vi "Main.vi"() -> ()   [LabVIEW 2018]
uses:
  <vilib>/picture/picture.llb/imagedata.ctl
  <vilib>/Utility/miscctls.llb/LVPoint32TypeDef.ctl
  <vilib>/Utility/miscctls.llb/LVMouseTypeDef.ctl
  <vilib>/Utility/miscctls.llb/LVPositionTypeDef.ctl
  <vilib>/Utility/miscctls.llb/LVPointTypeDef.ctl
  <vilib>/Utility/miscctls.llb/LVRectTypeDef.ctl
  Shared Variables/Alarm Cluster (UI).ctl
  Shared Variables/Alarm Cluster.ctl
  Drag and Drop/State Cluster.ctl
  support/Message Queue/Message Cluster.ctl
  Drag and Drop/Thumbnail Cluster.ctl
  Drag and Drop/Object Cluster.ctl
  Drag and Drop/Object Type Enum.ctl
  Config Module/Controls/Main Config Cluster.ctl
  OPC/OPC Module Config.ctl
  Scale Module Folder/Measure Instrument/State Enum.ctl
  OPC/OPC Settings.ctl
  OPC/Variable Data Cluster.ctl
  <vilib>/OPCUA/controls/NodeId.ctl
  <vilib>/OPCUA/controls/OPC UA StatusCode.ctl
  <vilib>/OPCUA/controls/Subscription ID.ctl
  <vilib>/OPCUA/controls/OPC UA Client Refnum.ctl
  <vilib>/OPCUA/controls/Subscription Data Change.ctl
  <vilib>/OPCUA/controls/Data Type.ctl
  OPC/OPC Tag Data.ctl
  Feed Module/Controls/Feed Module Config Cluster.ctl
  Feed Module/Controls/Feed Module Settings Cluster.ctl
  Ismatec ISM 831C/Controls/Ismatech ISM831C Settings Cluster.ctl
  Masterflex 7550-30/Controls/Settings Cluster.ctl
  Mettler Toledo/Controls/Settings Cluster.ctl
  Bronkhorst M13 Flow Meter/Settings Cluster.ctl
  Measure Instrument/PID 2 Parameters Cluster.ctl
  Measure Instrument/PID Input Enum.ctl
  Measure Instrument/PID 2 Output Enum.ctl
  Tacmina QI/Tacmina QI DAQ Setting.ctl
  KNF Pump/Settings Cluster plus SIMDOS.ctl
  ASIA Pump/Pump Settings.ctl
  VICI M50 Party Mode/Settings Cluster.ctl
  FLOM Pump/Settings Cluster.ctl
  SSI PR Class/SSI PR or LD Settings Cluster.ctl
  Masterflex 75211/Masterflex 75211 DAQ Setting.ctl
  SSI PR Class/SSI P40 Settings Cluster.ctl
  Ismatec 78001/Ismatec 4083.ctl
  Bronkhorst M14 Flow Meter/Settings Cluster.ctl
  TT Module/Controls/TT Module Config Cluster.ctl
  Tag VIs/Numeric Alarm Settings Cluster.ctl
  Acquisition/Hardware Configuration.ctl
  Acquisition/Task Cluster.ctl
  PT Module/Controls/PT Module Config Cluster.ctl
  Scale Module Folder/Feed Module/Controls/Scale Module Config Cluster.ctl
  Scale Module Folder/Feed Module/Controls/Scale Module Settings Cluster.ctl
  Pump Module Folder/Pump Module Config Cluster.ctl
  Pump Module Folder/Pump Module Settings Cluster.ctl
  LabJack Module/Controls/U3 Module Config Cluster.ctl
  Decoration Module/Decoration Module Config Cluster.ctl
  Flow Module Folder/Feed Module/Controls/Flow Module Config Cluster.ctl
  Flow Module Folder/Feed Module/Controls/Flow Module Settings Cluster.ctl
  TCU Module/TCU Module Folder/TCU Module Config Cluster.ctl
  TCU Module/TCU Module Folder/TCU Module Settings Cluster.ctl
  TCU Module/TCU Module Folder/Measure Instrument/Output Devices.ctl
  Huber TCU/Huber Settings.ctl
  Lauda Integral XT-150 TCU/Lauda Settings.ctl
  Julabo Type 1 TCU/Julabo Type 1 TCU Folder/Julabo FP-50 Settings.ctl
  Huber Unistat 410 TCU/Huber Unistat 410 RS485 Settings.ctl
  D-O Module Folder/Not Sure Where this is Used.ctl
  Sequencing/Squence Control.ctl
  D-O Module Folder/D-O Module Config Cluster.ctl
  D-O Module Folder/Valve Clusters.ctl
  D-O Module Folder/D-O Module Settings Cluster.ctl
  D-O Module Folder/D-O Device Settings Cluster.ctl
  VICI Electronic Actuator/VICI Electronic Actuator Settings.ctl
  Pressure Regulator Control Module/Pressure Regulator/Controls/4-20mA Module Config Cluster.ctl
  Pressure Regulator Control Module/Pressure Regulator/Controls/4-20mA Module Settings Cluster.ctl
  Pressure Transmitter/Pressure Transmitter Device Settings.ctl
  Pressure Reg Module/Pressure Regulator Device Settings.ctl
  Sonicator Module Folder/Feed Module/Controls/Sonicator Module Config Cluster.ctl
  Sonicator Module Folder/Feed Module/Controls/Sonicator Module Settings Cluster.ctl
  Sonic Systems P100/Sonic Systems P100 Settings.ctl
  Agitator Module Folder/Feed Module/Controls/Agitator Module Config Cluster.ctl
  Agitator Module Folder/Feed Module/Controls/Agitator Module Settings Cluster.ctl
  Tag VIs/Tag FGV Operation Enum.ctl
  Shared Variables/Alarm Log Operation Enum.ctl
  Drag and Drop/Drop Parameters Cluster.ctl
  Drag and Drop/Module Instance Number Operation Enum.ctl
  Drag and Drop/Module Type Enum.ctl
  <vilib>/Utility/error.llb/DialogType.ctl
  Config Module/Controls/Config File Operation Enum.ctl
  Waveform Loop/Start Params Cluster.ctl
  Ismatec 78001/Ismatec 4083 Global.ctl
  Ismatec 78001/Ismatec 4083 Global Element.ctl
  Pump Calibration Program/Pump Calibration Config.ctl
  support/Message Queue/Enqueue Message (Single).vi
  <vilib>/Utility/cursorutil.llb/Set Cursor (Icon Pict).vi
  Main/Main Globals.vi
  LabJack Module/U3 (Main).vit
  D-O Module Folder/D-O Module (Main).vi
  TCU Module/TCU Module Folder/TCU Module (Main).vi
  Flow Module Folder/Flow Module (Main).vi
  Sonicator Module Folder/Sonicator Module (Main).vi
  Agitator Module Folder/Agitator Module (Main).vi
  <vilib>/Utility/cursorutil.llb/Set Cursor (Cursor ID).vi
  support/Message Queue/Message Queue.lvlib
  support/User Event - Stop/User Event - Stop.lvlib
  support/Support Library.lvlib
  Drag and Drop/Drag and Drop.lvlib
  Feed Module/Feed Module.lvlib
  TT Module/TT Module.lvlib
  History Graph/History Graph.lvlib
  Waveform Loop/Waveform Loop.lvlib
  CSV Log/CSV Log.lvlib
  TDMS Log/TDMS Log.lvlib
  Shared Variables/Dynamic Shared Variables.lvlib
  DAQ/DAQ.lvlib
  Config Module/Config Module.lvlib
  Bronkhorst M13 Flow Meter/Bronkhorst M13 Flow Meter.lvlib
  Mettler Toledo/Mettler Toledo.lvlib
  Masterflex 7550-30/Masterflex 7550-30.lvlib
  Ismatec ISM 831C/Ismatec ISM 831C.lvlib
  PT Module/PT Module.lvlib
  Scale Module Folder/Scale Module.lvlib
  Pump Module Folder/Pump Module.lvlib
  <vilib>/lvdsc/NI_DSC.lvlib
  LabJack Module/U3 Module.lvlib
  Flow Module Folder/Flow Module.lvlib
  Tacmina QI/Tacmina QI.lvlib
  KNF Pump/KNF SIMDOS.lvlib
  Huber TCU/Huber Ministat 230 TCU.lvlib
  TCU Module/TCU Module Folder/TCU Module.lvlib
  Lauda Integral XT-150 TCU/Lauda TCU.lvlib
  Julabo Type 1 TCU/Julabo Type 1 TCU Folder/Julabo Type FP-50 TCU.lvlib
  ASIA Pump.lvlib
  Sequencing/Sequencing Library.lvlib
  VICI M50 Party Mode/VICI M6 M50 Party Mode.lvlib
  D-O Module Folder/D-O Module.lvlib
  Pressure Regulator Control Module/Pressure Regulator/4-20mA Module.lvlib
  Pressure Reg Module/Pressure Regulator Library.lvlib
  Pressure Transmitter/Pressure Transmitter Library.lvlib
  FLOM Pump/FLOM Pump.lvlib
  support/Command Log VIs/Command Logging.lvlib
  Calibration VIs/Calibration.lvlib
  Lauda Integral XT-150 TCU/TCP Library.lvlib
  SSI PR Class/SSI PR or LD Pump.lvlib
  Scale Module Folder/Measure Instrument/Scale Module Engine.lvlib
  OPC/OPC UA.lvlib
  D-O Module Folder/DIO Valve/VICI Electronic Actuator.lvlib
  subVIs/Main SubVIs.lvlib
  Masterflex 75211/Masterflex 75211.lvlib
  SSI PR Class/SSI P40 Pump.lvlib
  Huber Unistat 410 TCU/Huber Unistat 410 TCU.lvlib
  Ismatec 78001/Ismatec 4308.lvlib
  Bronkhorst M14 Flow Meter/Bronkhorst M14 Flow Meter.lvlib
  Sonicator Module Folder/Sonicator Module.lvlib
  Sonic Systems P100/Sonic Systems P100.lvlib
  Agitator Module Folder/Agitator Module.lvlib
panel:
  out "Cluster":T1 {"Main Config"."PR Module Configs"."Settings"."PID 2 Parameters"."output range"."output low" format="%.2f"; "Main Config"."PR Module Configs"."Settings"."PID 2 Parameters"."output range"."output high" min=0.0 max=100.0 format="%.2f"; "Main Config"."PR Module Configs"."Settings"."PID 2 Parameters"."PID gains"."derivative time (Td, min)" format="%.3f"; "Main Config"."PR Module Configs"."Settings"."PID 2 Parameters"."PID gains"."integral time (Ti, min)" format="%.3f"; "Main Config"."PR Module Configs"."Settings"."PID 2 Parameters"."PID gains"."proportional gain (Kc)" format="%.3f"; "Main Config"."Steps"."Control" items=["Pump %", "Setpoint"]; "Main Config"."TCU Module Configs"."Settings"."Huber Unistat 410 Settings"."Address" min=0 max=99 format="%02.0f"; "Main Config"."TCU Module Configs"."Settings"."Julabo FP-50 Settings"."Pump Power" min=0 max=8 step=1; "Main Config"."TCU Module Configs"."Settings"."Lauda Settings"."Pump Power" min=0 max=8 step=1; "Main Config"."Flow Module Configs"."Settings"."Bronkhorst M14 Settings"."Smoothing Steps" min=1 step=1; "Main Config"."Flow Module Configs"."Settings"."Bronkhorst M13 Settings"."Smoothing Steps" min=1 step=1; "Main Config"."Pump Module Configs"."Settings"."Ismatech 3 Channel Settings"."Channel Number" min=0 max=3; "Main Config"."Pump Module Configs"."Settings"."Ismatech 3 Channel Settings"."Pump Number" min=1; "Main Config"."Pump Module Configs"."Settings"."ASIA Pump C"."channel" min=0 max=1 step=1; "Main Config"."Pump Module Configs"."Settings"."Masterflex"."Pump Number" min=1.0 max=20.0 step=1.0; "Main Config"."Pump Module Configs"."Settings"."Ismatech"."Pump Number" min=1.0 max=20.0 step=1.0; "Main Config"."Feed Module Configs"."Settings"."Bronkhorst M14 Settings"."Smoothing Steps" min=1 step=1; "Main Config"."Feed Module Configs"."Settings"."Ismatech 3 Channel Settings"."Channel Number" min=0 max=3; "Main Config"."Feed Module Configs"."Settings"."Ismatech 3 Channel Settings"."Pump Number" min=1; "Main Config"."Feed Module Configs"."Settings"."output range"."output low" min=0.0 max=100.0 format="%.2f"; "Main Config"."Feed Module Configs"."Settings"."output range"."output high" format="%.2f"; "Main Config"."Feed Module Configs"."Settings"."PID 2 Parameters"."PID gains"."derivative time (Td, min)" format="%.3f"; "Main Config"."Feed Module Configs"."Settings"."PID 2 Parameters"."PID gains"."integral time (Ti, min)" format="%.3f"; "Main Config"."Feed Module Configs"."Settings"."PID 2 Parameters"."PID gains"."proportional gain (Kc)" format="%.3f"; "Main Config"."Feed Module Configs"."Settings"."Bronkhorst M13 Flow Meter"."Smoothing Steps" min=1 step=1; "Main Config"."Feed Module Configs"."Settings"."ASIA Pump C"."channel" min=0 max=1 step=1; "Main Config"."Feed Module Configs"."Settings"."Ismatech"."Pump Number" min=1.0 max=20.0 step=1.0; "Main Config"."Feed Module Configs"."Settings"."Masterflex"."Pump Number" min=1.0 max=20.0 step=1.0}
  in  "Alarm History Button":bool
  out "Alarm Model":T73[](array[typedef]) {"Alarm"."value" format="%.2f"; "Alarm"."setpoint" format="%.2f"; "Alarm"."clear time" format="%<%X\n%x>T"; "Alarm"."ack time" format="%<%X\n%x>T"; "Alarm"."set time" format="%<%X\n%x>T"}
  in  "UI Alarms":T74[](array[typedef])
  out "Message Data":variant
  out "data":errorcluster
  in  "End Program":bool
  out "CSV Log File":path
  out "error out":errorcluster
  in  "E-Stop":bool
  out "x-y":T4
  out "Front Panel Window:Panel Bounds":T4
  out "Drop Offset":T6
  out "Origin":T75
  out "Position":T6
  out "output cluster":cluster{"Coords":T10, "Mouse":T76}
  out "Mouse Position":cluster{"X":i32, "Y":i32}
  out "Path":path
  out "index of element":i32
  out "image data":T77
  in  "Notebook":string="Test"
  in  "Exit":bool
  in  "Settings":bool
  in  "Pause Log Button":bool
  in  "Force Trigger":bool
  in  "Start Log":bool
  out "Canvas":picture
  out "Palette":picture
  in  "?":T1 {"Main Config"."PR Module Configs"."Settings"."PID 2 Parameters"."output range"."output low" format="%.2f"; "Main Config"."PR Module Configs"."Settings"."PID 2 Parameters"."output range"."output high" min=0.0 max=100.0 format="%.2f"; "Main Config"."PR Module Configs"."Settings"."PID 2 Parameters"."PID gains"."derivative time (Td, min)" format="%.3f"; "Main Config"."PR Module Configs"."Settings"."PID 2 Parameters"."PID gains"."integral time (Ti, min)" format="%.3f"; "Main Config"."PR Module Configs"."Settings"."PID 2 Parameters"."PID gains"."proportional gain (Kc)" format="%.3f"; "Main Config"."Steps"."Control" items=["Pump %", "Setpoint"]; "Main Config"."TCU Module Configs"."Settings"."Huber Unistat 410 Settings"."Address" min=0 max=99 format="%02.0f"; "Main Config"."TCU Module Configs"."Settings"."Julabo FP-50 Settings"."Pump Power" min=0 max=8 step=1; "Main Config"."TCU Module Configs"."Settings"."Lauda Settings"."Pump Power" min=0 max=8 step=1; "Main Config"."Flow Module Configs"."Settings"."Bronkhorst M14 Settings"."Smoothing Steps" min=1 step=1; "Main Config"."Flow Module Configs"."Settings"."Bronkhorst M13 Settings"."Smoothing Steps" min=1 step=1; "Main Config"."Pump Module Configs"."Settings"."Ismatech 3 Channel Settings"."Channel Number" min=0 max=3; "Main Config"."Pump Module Configs"."Settings"."Ismatech 3 Channel Settings"."Pump Number" min=1; "Main Config"."Pump Module Configs"."Settings"."ASIA Pump C"."channel" min=0 max=1 step=1; "Main Config"."Pump Module Configs"."Settings"."Masterflex"."Pump Number" min=1.0 max=20.0 step=1.0; "Main Config"."Pump Module Configs"."Settings"."Ismatech"."Pump Number" min=1.0 max=20.0 step=1.0; "Main Config"."Feed Module Configs"."Settings"."Bronkhorst M14 Settings"."Smoothing Steps" min=1 step=1; "Main Config"."Feed Module Configs"."Settings"."Ismatech 3 Channel Settings"."Channel Number" min=0 max=3; "Main Config"."Feed Module Configs"."Settings"."Ismatech 3 Channel Settings"."Pump Number" min=1; "Main Config"."Feed Module Configs"."Settings"."output range"."output low" min=0.0 max=100.0 format="%.2f"; "Main Config"."Feed Module Configs"."Settings"."output range"."output high" format="%.2f"; "Main Config"."Feed Module Configs"."Settings"."PID 2 Parameters"."PID gains"."derivative time (Td, min)" format="%.3f"; "Main Config"."Feed Module Configs"."Settings"."PID 2 Parameters"."PID gains"."integral time (Ti, min)" format="%.3f"; "Main Config"."Feed Module Configs"."Settings"."PID 2 Parameters"."PID gains"."proportional gain (Kc)" format="%.3f"; "Main Config"."Feed Module Configs"."Settings"."Bronkhorst M13 Flow Meter"."Smoothing Steps" min=1 step=1; "Main Config"."Feed Module Configs"."Settings"."ASIA Pump C"."channel" min=0 max=1 step=1; "Main Config"."Feed Module Configs"."Settings"."Ismatech"."Pump Number" min=1.0 max=20.0 step=1.0; "Main Config"."Feed Module Configs"."Settings"."Masterflex"."Pump Number" min=1.0 max=20.0 step=1.0}
  # "little pump\ncentrifigual pump\nflow rate\npressure\nS or P to the left\nsolvent or process"
  # "Question: how do we make the live VI, such as the feed module graphic\nsized right for the picture that is loaded?\n\nProbably should standarize each module size. Then the  flow sheet\ndrawings will all just match the size and we don't have to worry about\nscale."
  # "Tasks\n1. Load graphic\n2. Drag and drop onto picture control\n3. Picture control draws hot spot\n4. If drag and drop on picture control, then resize and redraw the nearest hotspot\n5. When operator turns \"ON\" the system, then the hotspots are replaced with actual VIs."
  # "vertical or horizontal lines\nextendable"
  # "as much drawing room as possible"
  # "Agitator Settings"
  # "Sonicator Settings"
  # "Instrument Settings"
  # "Instrument Settings"
  # "Output Instruments"
  # "Flow Meter Settings"
  # "Output Instruments"
  # "Scale Settings"
  # "Output Instruments"
  # "Input Instruments"
  # "Agitator Settings"
  # "Sonicator Settings"
  # "Instrument Settings"
  # "Instrument Settings"
  # "Output Instruments"
  # "Flow Meter Settings"
  # "Output Instruments"
  # "Scale Settings"
  # "Output Instruments"
  # "Input Instruments"
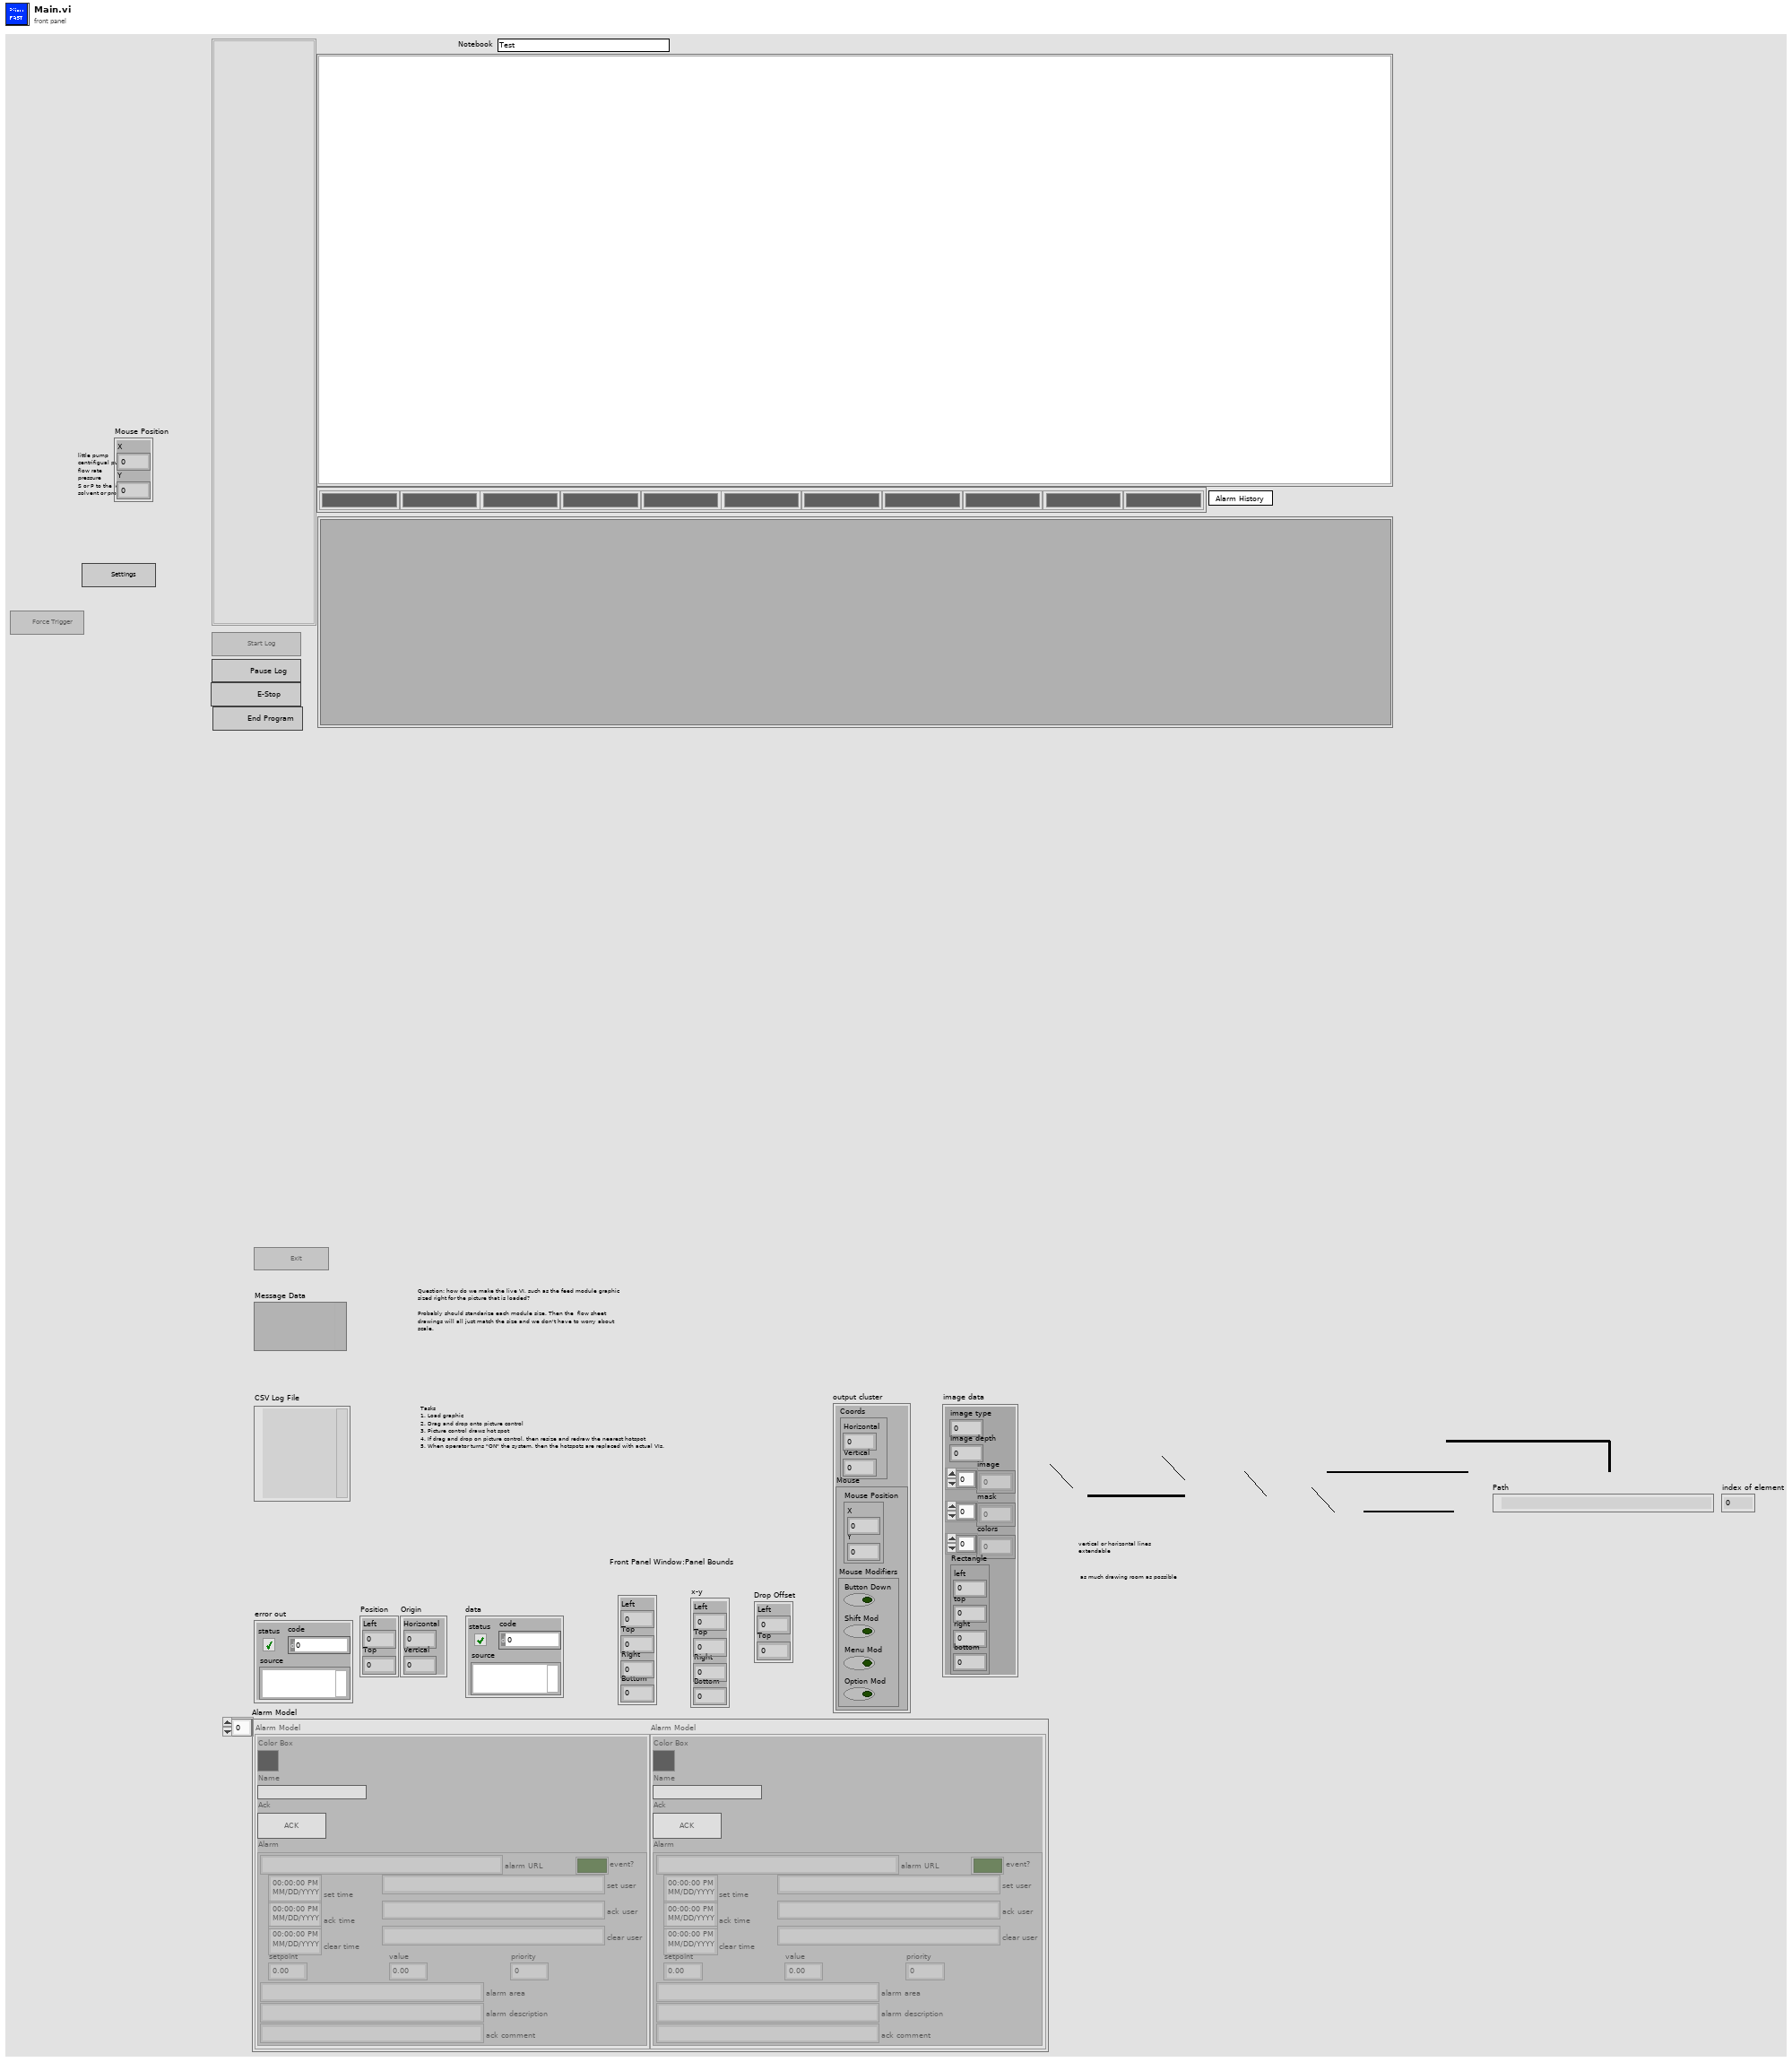
[diagram p1: front panel]
types:
  T1 = typedef "Drag and Drop.lvlib/State Cluster.ctl" = cluster{"VI refs":refnum<vi>[], "Queues":refnum<queue>[], "[Thumbnails]":T2[], "Drag Object Idx":i32, "[Objects]":T3[], "Active Object":i32, "Drop Offset":T6, "Process Name":string, "Main Config":T7, "Campaign Filepath":path, "Config Changed?":bool}
  T2 = typedef "Thumbnail Cluster.ctl" = cluster{"Path":path, "Rectangle":cluster{"left":i16, "top":i16, "right":i16, "bottom":i16}}
  T3 = typedef "Object Cluster.ctl" = cluster{"BMP Path":path, "Anchor Position":cluster{"X":i32, "Y":i32}, "Hot Spot":T4, "Type":T5, "Parameters":variant}
  T4 = typedef "LVRectTypeDef.ctl" = cluster{"Left":i16, "Top":i16, "Right":i16, "Bottom":i16}
  T5 = typedef "Object Type Enum.ctl" = enum16{"Icon", "Line", "Text", "Feed Module"}
  T6 = typedef "LVPositionTypeDef.ctl" = cluster{"Left":i32, "Top":i32}
  T7 = typedef "Config Module.lvlib/Main Config Cluster.ctl" = cluster{"Notebook":string, "OPC Module Configs":T8[], "Feed Module Configs":T18[], "Log File Path":path, "TT Module Configs":T37[], "DAQ Config":T39, "PT Module Configs":T41[], "Scale Module Configs":T42[], "Pump Module Configs":T44[], "U3 Module Configs":T46[], "Decoration Module Configs":T47[], "Flow Module Configs":T48[], "TCU Module Configs":T50[], "Steps":T57, "Abort":bool, "DO Module Configs":T59[], "PR Module Configs":T64[], "SC Module Configs":T68[], "AM Module Configs":T71[], "Cycle Period":dbl}
  T8 = typedef "OPC UA.lvlib/OPC Module Config.ctl" = cluster{"State":T9, "GUID":string, "Drop Coords":T10, "Configuration":T11, "First Iteration":bool, "Data":cluster{"Object Name":string, "Variable Array":T12[]}[], "Process Name":string, "Load Count":i32, "Log Started":bool, "subscription ID out":T15, "OPC UA client refnum out":T16, "Event Registration Refnum":refnum<event-registration>, "Start Time":timestamp, "Current Time":timestamp, "Tag Data":T17[]}
  T9 = typedef "Scale Module.lvlib/Scale Module Engine.lvlib/State Enum.ctl" = enum16{"Measuring", "Idle"}
  T10 = typedef "LVPoint32TypeDef.ctl" = cluster{"Horizontal":i32, "Vertical":i32}
  T11 = typedef "OPC UA.lvlib/OPC Settings.ctl" = cluster{"Cycle Period":dbl, "server endpoint URL":string, "security policy":cluster{"message mode":enum16{"None", "Sign", "Sign and Encrypt"}, "security":enum16{"Basic256", "Basic128Rsa15"}}, "Trust Any Server":bool}
  T12 = typedef "OPC UA.lvlib/Variable Data Cluster.ctl" = cluster{"node ID":T13, "browse name":string, "status":T14, "timestamp":timestamp, "value ":variant}
  T13 = typedef "NodeId.ctl" = string
  T14 = typedef "OPC UA StatusCode.ctl" = u32
  T15 = typedef "Subscription ID.ctl" = u32
  T16 = typedef "OPC UA Client Refnum.ctl" = refnum<k21>
  T17 = typedef "OPC UA.lvlib/OPC Tag Data.ctl" = cluster{"Include this Device":bool, "Device Name":string, "OPC Tag Data":cluster{"Tag":string, "Value":variant, "Time Stamp":timestamp}[]}
  T18 = typedef "Feed Module.lvlib/Feed Module Config Cluster.ctl" = cluster{"GUID":string, "Drop Coords":T10, "Process Name":string, "Queue Name":string, "Settings":T19, "Settings Load Count":i32, "OP Load Count":i32}
  T19 = typedef "Feed Module.lvlib/Feed Module Settings Cluster.ctl" = cluster{"Cycle Period":dbl, "Ismatech":T20, "Masterflex":T21, "Mettler":T22, "Bronkhorst M13 Flow Meter":T23, "PID 2 Parameters":T24, "Manual Entry":dbl, "Auto?":bool, "output range":cluster{"output high":dbl, "output low":dbl}, "Tacmina Settings":T27, "KNF SIMDOS Settings":T28, "ASIA Pump C":T29, "VICI Settings":T30, "FLOM Settings":T31, "SSI PR/LD Settings":T32, "Masterflex 75211 Settings":T33, "SSI P40 Settings":T34, "Ismatech 3 Channel Settings":T35, "Bronkhorst M14 Settings":T36}
  T20 = typedef "Ismatec ISM 831C.lvlib/Ismatech ISM831C Settings Cluster.ctl" = cluster{"VISA resource name":refnum<visa-resource-name>, "Simulated?":bool, "Pump Number":dbl, "Reverse?":bool}
  T21 = typedef "Masterflex 7550-30.lvlib/Settings Cluster.ctl" = cluster{"VISA resource name":refnum<visa-resource-name>, "Simulated?":bool, "Pump Number":dbl, "Reverse?":bool}
  T22 = typedef "Mettler Toledo.lvlib/Settings Cluster.ctl" = cluster{"VISA resource name":refnum<visa-resource-name>, "Simulated?":bool}
  T23 = typedef "Bronkhorst M13 Flow Meter.lvlib/Settings Cluster.ctl" = cluster{"VISA resource name":refnum<visa-resource-name>, "Simulated?":bool, "Smoothing Steps":i32}
  T24 = typedef "PID 2 Parameters Cluster.ctl" = cluster{"Input Device":T25, "Output Device":T26, "Setpoint":dbl, "PID gains":cluster{"proportional gain (Kc)":dbl, "integral time (Ti, min)":dbl, "derivative time (Td, min)":dbl}}
  T25 = typedef "PID Input Enum.ctl" = enum16{"Default", "Bronkhorst M13", "Bronkhorst M14", "Scale Rate of Change"}
  T26 = typedef "PID 2 Output Enum.ctl" = enum16{"Default", "Ismatec ISM 4308", "Ismatec ISM 831C", "Masterflex 7550-30", "VICI", "Tacmina QI", "KNF SIMDOS", "ASIA Type C", "FLOM UI-22-11", "SSI PR/LD", "SSI P40", "Masterflex 75211-70"}
  T27 = typedef "Tacmina QI.lvlib/Tacmina QI DAQ Setting.ctl" = cluster{"Analog DAQ Task":refnum<k21>, "Digital DAQ Task":refnum<k21>}
  T28 = typedef "KNF SIMDOS.lvlib/Settings Cluster plus SIMDOS.ctl" = cluster{"VISA resource name":refnum<visa-resource-name>, "Simulated?":bool}
  T29 = typedef "ASIA Pump.lvlib/Pump Settings.ctl" = cluster{"ASIA Pump #":i32, "channel":i32, "Simulated":bool}
  T30 = typedef "VICI M6 M50 Party Mode.lvlib/Settings Cluster.ctl" = cluster{"VISA resource name":refnum<visa-resource-name>, "Simulated?":bool, "Pump Letter":string, "Reverse?":bool}
  T31 = typedef "FLOM Pump.lvlib/Settings Cluster.ctl" = cluster{"VISA resource name":refnum<visa-resource-name>, "Simulated?":bool, "Pump Number":dbl}
  T32 = typedef "SSI PR or LD Pump.lvlib/SSI PR or LD Settings Cluster.ctl" = cluster{"VISA resource name":refnum<visa-resource-name>, "Simulated?":bool}
  T33 = typedef "Masterflex 75211.lvlib/Masterflex 75211 DAQ Setting.ctl" = cluster{"Analog DAQ Task":refnum<k21>, "Digital DAQ Task":refnum<k21>}
  T34 = typedef "SSI P40 Pump.lvlib/SSI P40 Settings Cluster.ctl" = cluster{"VISA resource name":refnum<visa-resource-name>, "Simulated?":bool}
  T35 = typedef "Ismatec 4308.lvlib/Ismatec 4083.ctl" = cluster{"VISA resource name":refnum<visa-resource-name>, "Pump Number":i16, "Channel Number":i16, "Simulated?":bool, "Reverse?":bool}
  T36 = typedef "Bronkhorst M14 Flow Meter.lvlib/Settings Cluster.ctl" = cluster{"VISA resource name":refnum<visa-resource-name>, "Simulated?":bool, "Smoothing Steps":i32}
  T37 = typedef "TT Module.lvlib/TT Module Config Cluster.ctl" = cluster{"GUID":string, "Drop Coords":T10, "Input Channel Tag Name ":string, "Process Name":string, "Queue Name":string, "Input Channel Numeric Alarm Settings":T38[]}
  T38 = typedef "Numeric Alarm Settings Cluster.ctl" = cluster{"enable? (F)":bool, "name":string, "alarm type":enum16{"HI_HI", "HI", "LO", "LO_LO"}, "level/change":dbl, "deadband/time":dbl, "alarm delay":dbl, "priority":u32, "ack type":enum16{"Auto", "User", "None", "Each Occurrence"}, "area":string, "description":string, "log? (T)":bool}
  T39 = typedef "DAQ.lvlib/Hardware Configuration.ctl" = cluster{"Tasks":T40[]}
  T40 = typedef "Task Cluster.ctl" = cluster{"DAQmx Task":refnum<k21>, "Read-Write Radio":enum32{"Read", "Write"}}
  T41 = typedef "PT Module.lvlib/PT Module Config Cluster.ctl" = cluster{"GUID":string, "Drop Coords":T10, "Input Channel Tag Name ":string, "Process Name":string, "Queue Name":string, "Input Channel Numeric Alarm Settings":T38[]}
  T42 = typedef "Scale Module.lvlib/Scale Module Config Cluster.ctl" = cluster{"GUID":string, "Drop Coords":T10, "Process Name":string, "Queue Name":string, "Settings":T43, "Load Count":i32}
  T43 = typedef "Scale Module.lvlib/Scale Module Settings Cluster.ctl" = cluster{"Cycle Period":dbl, "Mettler":T22, "Scale Type":string}
  T44 = typedef "Pump Module.lvlib/Pump Module Config Cluster.ctl" = cluster{"GUID":string, "Drop Coords":T10, "Process Name":string, "Queue Name":string, "Settings":T45, "Load Count":i32}
  T45 = typedef "Pump Module.lvlib/Pump Module Settings Cluster.ctl" = cluster{"Cycle Period":dbl, "Manual Entry":dbl, "Output Device":T26, "Ismatech":T20, "Ismatech 3 Channel Settings":T35, "Masterflex":T21, "VICI Settings":T30, "Tacmina Settings":T27, "KNF SIMDOS Settings":T28, "ASIA Pump C":T29, "FLOM Settings":T31, "SSI PR/LD Settings":T32, "SSI P40 Settings":T32, "Masterflex 75211 Settings":T33, "Pump Calibration File":path, "Calibration Slope":dbl, "Calibration Y Intercept":dbl, "Pump Cal Enum":u16}
  T46 = typedef "U3 Module.lvlib/U3 Module Config Cluster.ctl" = cluster{"GUID":string, "Drop Coords":T10, "AI Channel Number":enum16{"Default", "AI0", "AI1", "AI2", "AI3", "AI4", "AI5", "AI6", "AI7"}, "Process Name":string, "Queue Name":string, "Input Channel Numeric Alarm Settings":T38[]}
  T47 = typedef "Decoration Module Config Cluster.ctl" = cluster{"GUID":string, "Drop Coords":T10, "Decoration Filepath":path}
  T48 = typedef "Flow Module.lvlib/Flow Module Config Cluster.ctl" = cluster{"GUID":string, "Drop Coords":T10, "Process Name":string, "Queue Name":string, "Settings":T49, "Load Count":i32}
  T49 = typedef "Flow Module.lvlib/Flow Module Settings Cluster.ctl" = cluster{"Cycle Period":dbl, "Flow Meter Type":string, "Bronkhorst M13 Settings":T23, "Bronkhorst M14 Settings":T36}
  T50 = typedef "TCU Module.lvlib/TCU Module Config Cluster.ctl" = cluster{"GUID":string, "Drop Coords":T10, "Process Name":string, "Queue Name":string, "Settings":T51, "Load Count":i32, "Power Level Changed":bool}
  T51 = typedef "TCU Module.lvlib/TCU Module Settings Cluster.ctl" = cluster{"Cycle Period":dbl, "Setpoint Entry":dbl, "Output Device":T52, "Huber Ministat 230 Settings":T53, "Lauda Settings":T54, "Julabo FP-50 Settings":T55, "Internal Control?":bool, "Huber Unistat 410 Settings":T56}
  T52 = typedef "Output Devices.ctl" = enum16{"Default", "Huber Ministat 230", "Huber Unistat 410", "Lauda XT-150", "Julabo FP-50"}
  T53 = typedef "Huber Ministat 230 TCU.lvlib/Huber Settings.ctl" = cluster{"VISA resource name":refnum<visa-resource-name>, "Simulated?":bool}
  T54 = typedef "Lauda TCU.lvlib/Lauda Settings.ctl" = cluster{"VISA resource name":refnum<visa-resource-name>, "Simulated?":bool, "Pump Power":i32}
  T55 = typedef "Julabo Type FP-50 TCU.lvlib/Julabo FP-50 Settings.ctl" = cluster{"VISA resource name":refnum<visa-resource-name>, "Simulated?":bool, "Pump Power":i32}
  T56 = typedef "Huber Unistat 410 TCU.lvlib/Huber Unistat 410 RS485 Settings.ctl" = cluster{"VISA resource name":refnum<visa-resource-name>, "Address":i8, "Simulated?":bool}
  T57 = typedef "Not Sure Where this is Used.ctl" = T58[]
  T58 = typedef "Sequencing Library.lvlib/Squence Control.ctl" = cluster{"Module":string, "Control":u16, "Value":dbl, "Wait (sec)":dbl}
  T59 = typedef "D-O Module.lvlib/D-O Module Config Cluster.ctl" = cluster{"GUID":string, "Drop Coords":T10, "Process Name":string, "Queue Name":string, "Settings":T60, "Load Count":i32}
  T60 = typedef "D-O Module.lvlib/Valve Clusters.ctl" = cluster{"Valve Settings":T61, "Valve Type":enum16{"Default", "Digital Output Valve", "VICI Electronic Actuator"}, "Time On (Sec)":dbl, "Time Off (Sec)":dbl, "Run?":bool}
  T61 = typedef "D-O Module.lvlib/D-O Module Settings Cluster.ctl" = cluster{"D-O Settings":T62, "VICI Electronic Actuator":T63}
  T62 = typedef "D-O Module.lvlib/D-O Device Settings Cluster.ctl" = cluster{"DAQmx Task Name":refnum<k21>, "Output Channel":u16, "Output Channel Names":string[]}
  T63 = typedef "VICI Electronic Actuator.lvlib/VICI Electronic Actuator Settings.ctl" = cluster{"VISA resource name":refnum<visa-resource-name>, "Mode":enum16{"Two Positions With Stops", "Two Positions Without Stops", "Mutiposition"}, "Simulated":bool}
  T64 = typedef "4-20mA Module.lvlib/4-20mA Module Config Cluster.ctl" = cluster{"GUID":string, "Drop Coords":T10, "Process Name":string, "Queue Name":string, "Settings":T65, "Settings Load Count":i32}
  T65 = typedef "4-20mA Module.lvlib/4-20mA Module Settings Cluster.ctl" = cluster{"Cycle Period":dbl, "PID 2 Parameters":cluster{"Input Device":enum16{"Default", "4-20mA"}, "Output Device":enum16{"Default", "Equilibar Pressure Reg", "Flow Regulator"}, "Setpoint":dbl, "PID gains":cluster{"proportional gain (Kc)":dbl, "integral time (Ti, min)":dbl, "derivative time (Td, min)":dbl}, "output range":cluster{"output low":dbl, "output high":dbl}}, "Manual Entry":dbl, "Auto?":bool, "4-20mA Input Settings":T66, "4-20mA Out Settings":T67, "Input Channel Tag Name ":string}
  T66 = typedef "Pressure Transmitter Library.lvlib/Pressure Transmitter Device Settings.ctl" = cluster{"Input Channel ":u16}
  T67 = typedef "Pressure Regulator Library.lvlib/Pressure Regulator Device Settings.ctl" = cluster{"Output DAQ Task":refnum<k21>}
  T68 = typedef "Sonicator Module.lvlib/Sonicator Module Config Cluster.ctl" = cluster{"GUID":string, "Drop Coords":T10, "Process Name":string, "Queue Name":string, "Settings":T69, "Load Count":i32}
  T69 = typedef "Sonicator Module.lvlib/Sonicator Module Settings Cluster.ctl" = cluster{"Cycle Period":dbl, "Sonicator Type":string, "SS P100 Settings":T70, "Setpoint (µm)":dbl, "Cutoff (W)":dbl}
  T70 = typedef "Sonic Systems P100.lvlib/Sonic Systems P100 Settings.ctl" = cluster{"VISA resource name":refnum<visa-resource-name>, "Simulated?":bool}
  T71 = typedef "Agitator Module.lvlib/Agitator Module Config Cluster.ctl" = cluster{"GUID":string, "Drop Coords":T10, "Process Name":string, "Queue Name":string, "Settings":T72, "Load Count":i32}
  T72 = typedef "Agitator Module.lvlib/Agitator Module Settings Cluster.ctl" = cluster{"Cycle Period":dbl, "Agitator Type":string, "Setpoint (µm)":dbl}
  T73 = typedef "Dynamic Shared Variables.lvlib/Alarm Cluster.ctl" = cluster{"Color Box":u32, "Name":string, "Ack":bool, "Alarm":cluster{"alarm URL":string, "set time":timestamp, "set user":string, "ack time":timestamp, "ack user":string, "clear time":timestamp, "clear user":string, "setpoint":dbl, "value":dbl, "priority":u32, "alarm area":string, "alarm description":string, "ack comment":string, "event?":bool, "Refnum":u64}}
  T74 = typedef "Dynamic Shared Variables.lvlib/Alarm Cluster (UI).ctl" = cluster{"Color Box":u32, "Name":string, "Ack":bool}
  T75 = typedef "LVPointTypeDef.ctl" = cluster{"Horizontal":i16, "Vertical":i16}
  T76 = typedef "LVMouseTypeDef.ctl" = cluster{"Mouse Position":cluster{"X":i32, "Y":i32}, "Mouse Modifiers":cluster{"Button Down":bool, "Shift Mod":bool, "Menu Mod":bool, "Option Mod":bool}}
  T77 = typedef "imagedata.ctl" = cluster{"image type":i32, "image depth":i32, "image":u8[], "mask":u8[], "colors":u32[], "Rectangle":cluster{"left":i16, "top":i16, "right":i16, "bottom":i16}}
  T78 = typedef "Tag FGV Operation Enum.ctl" = enum16{"Init", "Set Notification Queue", "Create Tag", "Commit", "Write Tag (Numeric)", "Write Tag (Boolean)", "Read All Tags", "Read One Tag", "Delete Tag Category", "Set Alarm Parameters (Numeric)", "Set Alarm Parameters (Boolean)", "Enable All Alarms", "Disable All Alarms", "Delete All Tags", "Read Alarms", "Ack Alarm", "Read Alarm Parameters (Numeric)", "Read Alarm Parameters (Boolean)"}
  T79 = cluster{"Down":bool, "Mouse":T76, "Drag":bool, "Canvas":bool}
  T80 = cluster{"Busy":bool, "ChannelCnt":dbl, "Initialized":bool, "Current Channel":dbl, "Initialized Channels":dbl[]}[]
  T81 = cluster{"Busy":bool, "PumpCnt":dbl, "RemoteEntered":bool, "OverpressureSet":bool}[]
  T82 = typedef "Main Queue Cluster.ctl" = cluster{"UI":refnum<queue>, "Waveform Loop":refnum<queue>, "CSV Log":refnum<queue>, "TDMS Log":refnum<queue>, "Graphs":refnum<queue>[], "DAQ":refnum<queue>, "Sequence":refnum<queue>, "TCP Write":refnum<queue>, "Sequence UI":refnum<queue>, "OPC UA Log":refnum<queue>, "TCP Read":refnum<queue>}
  T83 = cluster{"Event Registration Refnum":refnum<event-registration>, "Stop Event Registration Refnum":refnum<event-registration>}
  T84 = typedef "Drag and Drop.lvlib/Module Type Enum.ctl" = enum16{"<unknown module>", "Feed", "TT", "PT", "Scale", "Flow", "Pump", "U3", "TCU", "DO", "PR", "OPC", "SC", "AM"}
  T85 = typedef "Module Instance Number Operation Enum.ctl" = enum16{"Init", "Next Instance Number"}
  T86 = typedef "Drop Parameters Cluster.ctl" = cluster{"Module VI Filepath":path, "Process Name":string, "Main UI Message Queue":refnum<queue>, "Drop Coords":T10, "Module Parameters":variant, "Name of Parent Window":string}
  T87 = enum8{"Enabled", "Disabled", "Disabled and Grayed Out"}
  T88 = typedef "Config Module.lvlib/Config File Operation Enum.ctl" = enum16{"Read", "Write"}
  T89 = typedef "Alarm Log Operation Enum.ctl" = enum16{"Create Log", "Log Alarm", "Close Log"}
  T90 = typedef "Waveform Loop.lvlib/Start Params Cluster.ctl" = cluster{"dt (seconds)":dbl, "CSV Logfile path":path, "TDMS Logfile path":path}
  T91 = typedef "Ismatec 4308.lvlib/Ismatec 4083 Global.ctl" = T92[]
  T92 = typedef "Ismatec 4308.lvlib/Ismatec 4083 Global Element.ctl" = cluster{"Busy":bool, "ChannelCnt":dbl, "Initialized":bool, "Current Channel":dbl, "Initialized Channels":dbl[]}
  T93 = typedef "Calibration.lvlib/Pump Calibration Config.ctl" = cluster{"Settings":cluster{"Cycle Period":dbl, "Ismatech":T20, "Masterflex":T21, "Bronkhorst M13 Settings":T23, "PID 2 Parameters":cluster{"Input Device":T25, "Output Device":T26}, "Tacmina Settings":T27, "KNF SIMDOS Settings":T28, "VICI M50 Settings":T30, "FLOM Settings":T31, "Calibration Limits":cluster{"Minimum (ml/min)":dbl, "Maximum (ml/min)":dbl, "Steps":dbl}, "SSI PR Settings":T32, "Ismatech 4308 Settings":T35, "Bronkhorst M14 Settings":T36}, "Flowmeter Output":dbl, "Density":dbl, "FL Temp":dbl, "Speed %":dbl, "File Refnum":refnum<file>, "Pump On?":enum16{"Off", "On", "Not Initialized"}}
  T94 = typedef "DialogType.ctl" = u16
  T95 = enum32{"Invalid", "Standard", "Closed", "Hidden", "Minimized", "Maximized"}
  T96 = cluster{"alarm URL":string, "set time":timestamp, "set user":string, "ack time":timestamp, "ack user":string, "clear time":timestamp, "clear user":string, "setpoint":dbl, "value":dbl, "priority":u32, "alarm area":string, "alarm description":string, "ack comment":string, "event?":bool, "Refnum":u64}[]
  T97 = cluster{"alarm URL":string, "set time":timestamp, "set user":string, "ack time":timestamp, "ack user":string, "clear time":timestamp, "clear user":string, "setpoint":dbl, "value":dbl, "priority":u32, "alarm area":string, "alarm description":string, "ack comment":string, "event?":bool, "Refnum":u64}
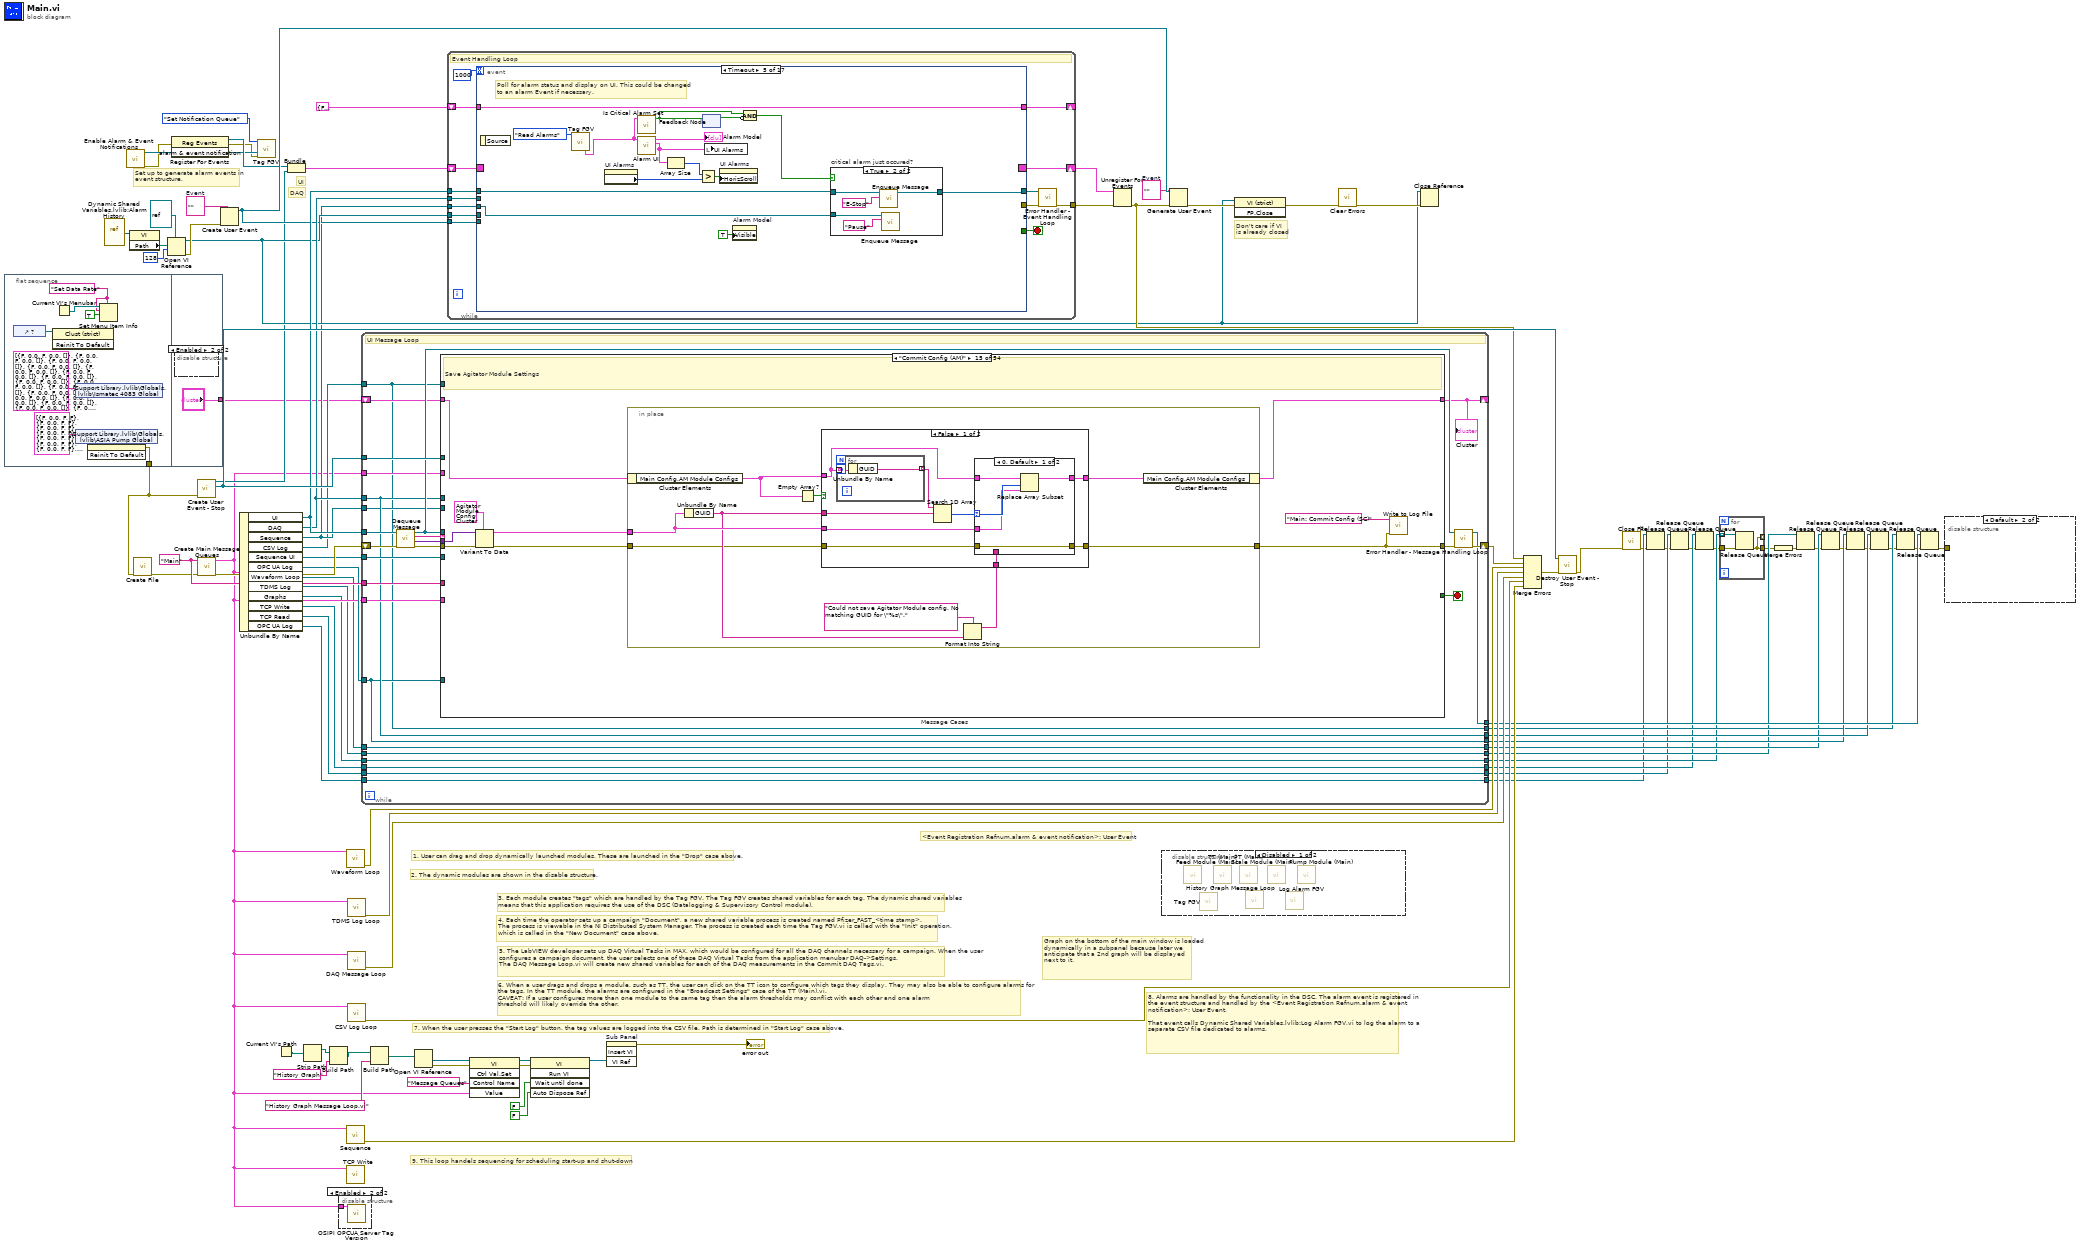
[diagram p0: block diagram]
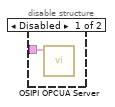
[diagram p2: hidden frame]
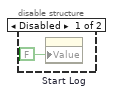
[diagram p3: hidden frame]
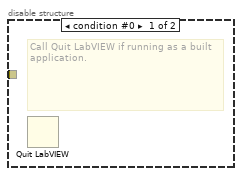
[diagram p4: hidden frame]
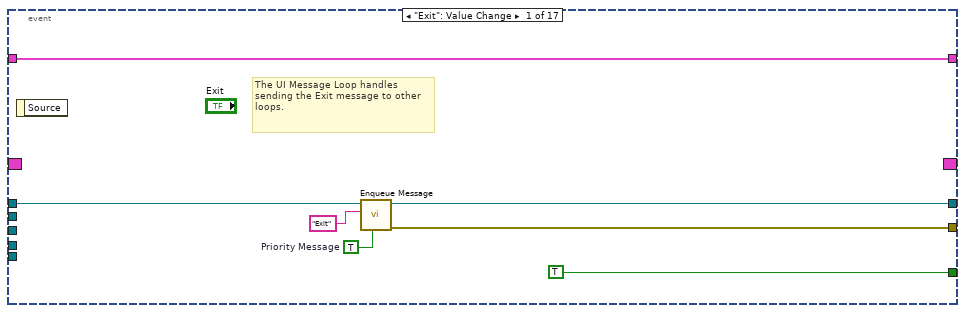
[diagram p6: hidden frame]
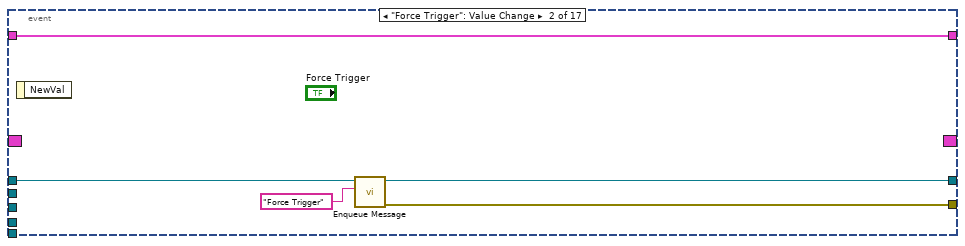
[diagram p7: hidden frame]
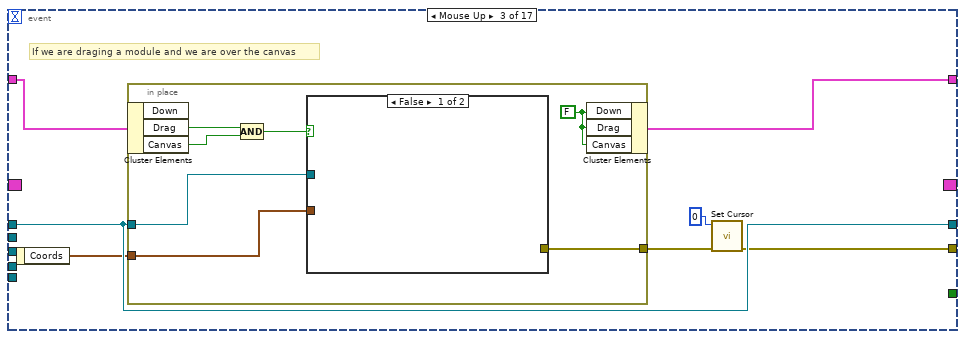
[diagram p8: hidden frame]
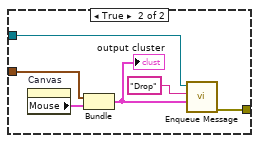
[diagram p9: hidden frame]
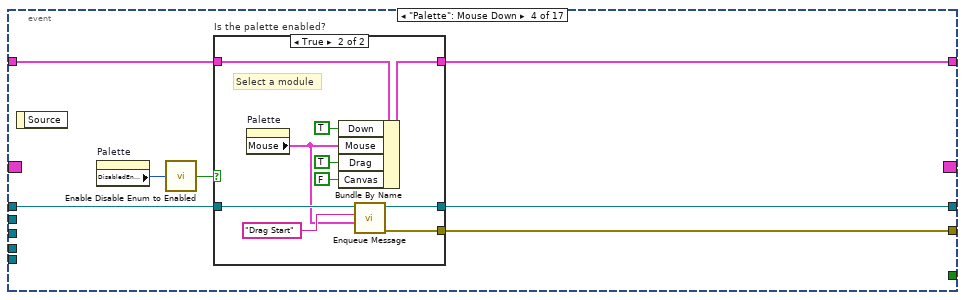
[diagram p10: hidden frame]
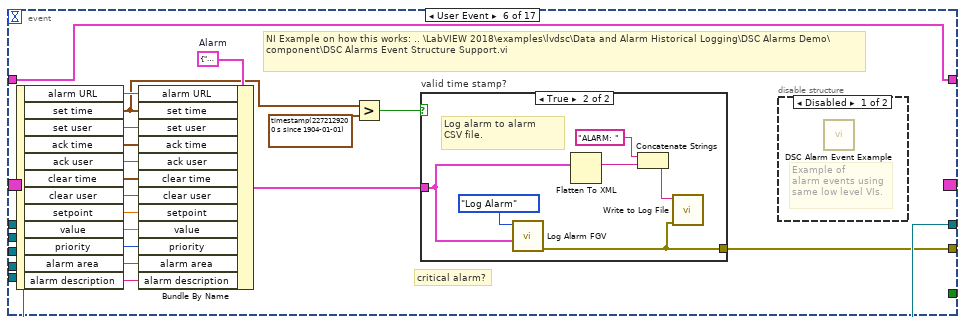
[diagram p13: hidden frame]
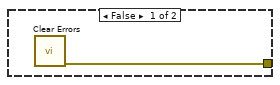
[diagram p15: hidden frame]
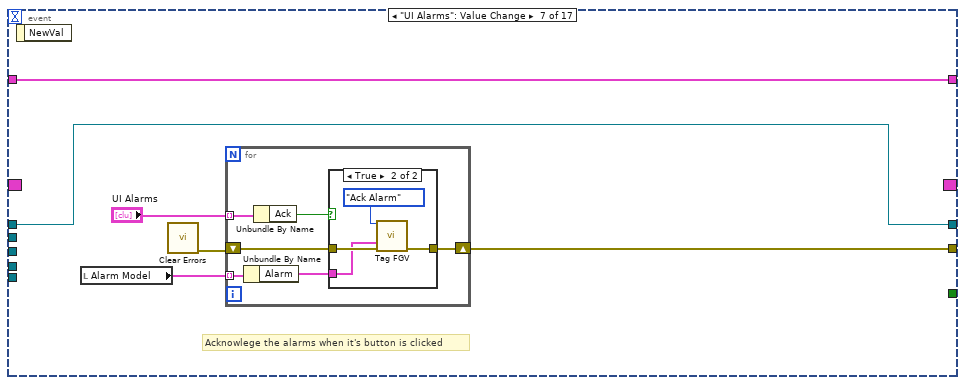
[diagram p16: hidden frame]
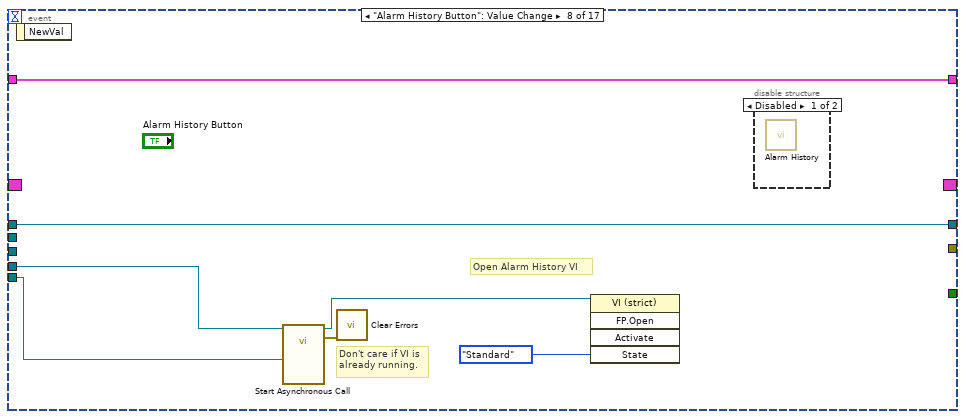
[diagram p18: hidden frame]
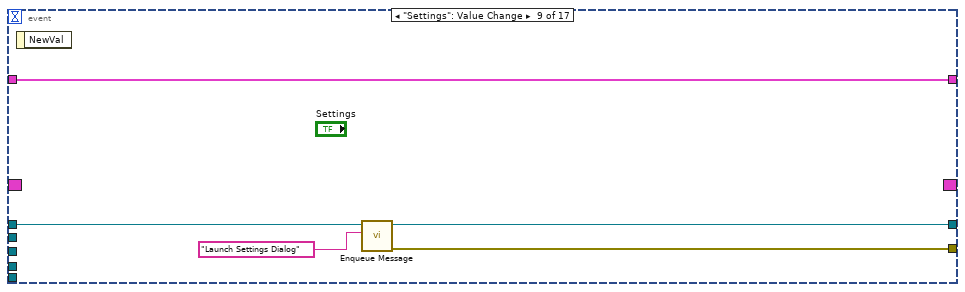
[diagram p20: hidden frame]
diagram:
  w50 = ""  # Event
  w57 = ""  # Event
  w80 = "Main" ("Process Name")
  # "<Event Registration Refnum.alarm & event notification>: User Event"
  # "9. This loop handels sequencing for scheduling start-up and shut-down"
  # "6. When a user drags and drops a module, such as TT, the user can click on the TT icon to configure which tags they display. They may also be able to configure alarms for\nthe tags. In the TT module, the alarms are configured in the \"Broadcast Settings\" case of the TT (Main).vi.\nCAVEAT: If a user configures more than one module to the same tag then the alarm thresholds may conflict with each other and one alarm\nthreshold will likely override the other."
  # "8. Alarms are handled by the functionality in the DSC. The alarm event is registered in the event structure and handled by the <Event Registration Refnum.alarm & event notification>: User Event.\n\nThat event calls Dynamic Shared Variables.lvlib:Log Alarm FGV.vi to log the alarm to a separate CSV file dedicated to alarms."
  # "Graph on the bottom of the main window is loaded dynamically in a subpanel because later we anticipate that a 2nd graph will be displayed\nnext to it."
  # "7. When the user presses the \"Start Log\" button, the tag values are logged into the CSV file. Path is determined in \"Start Log\" case above."
  # "5. The LabVIEW developer sets up DAQ Virtual Tasks in MAX, which would be configured for all the DAQ channels necessary for a campaign. When the user configures a campaign document, the user selects one of these DAQ Virtual Tasks from the application menubar DAQ->Settings.\nThe DAQ Message Loop.vi will create new shared variables for each of the DAQ measurements in the Commit DAQ Tags.vi."
  # "4. Each time the operator sets up a campaign \"Document\", a new shared variable process is created named Pfizer_FAST_<time stamp>.\nThe process is viewable in the NI Distributed System Manager. The process is created each time the Tag FGV.vi is called with the \"Init\" operation,\nwhich is called in the \"New Document\" case above."
  # "3. Each module creates \"tags\" which are handled by the Tag FGV. The Tag FGV creates shared variables for each tag. The dynamic shared variables\nmeans that this application requires the use of the DSC (Datalogging & Supervisory Control module)."
  # "2. The dynamic modules are shown in the disable structure."
  # "1. User can drag and drop dynamically launched modules. These are launched in the \"Drop\" case above."
  # "Set up to generate alarm events in\nevent structure."
  # "Don't care if VI\nis already closed"
  # "DAQ"
  # "UI"
  n1 = flat-sequence {
    tunnel: [w92] -> w39
    tunnel: ["?"] -> w40
    frame #0 {
      w90 = "Set Data Rate" ("item tag")
      n2 = control-ref of="?"() -> (w94:refnum<vi>)
      n3 = invoke class="Clust (strict)" method="Reinit To Default"(reference=w94) -> ()  [unwired: 2 in, 3 out]
      n4 = Current VI's Menubar() -> (w91:refnum<k9>)
      n5 = shared-variable ".\\Support Library.lvlib\\Globals.lvlib\\Ismatec 4083 Global"(T80 [{"Busy"=FALSE, "ChannelCnt"=0.0, "Initialized"=FALSE, "Current Channel"=0.0, "Initialized Channels"=[]}, {"Busy"=FALSE, "ChannelCnt"=0.0, "Initialized"=FALSE, "Current Channel"=0.0, "Initialized Channels"=[]}, {"Busy"=FALSE, "ChannelCnt"=0.0, "Initialized"=FALSE, "Current Channel"=0.0, "Initialized Channels"=[]}, {"Busy"=FALSE, "ChannelCnt"=0.0, "Initialized"=FALSE, "Current Channel"=0.0, "Initialized Channels"=[]}, {"Busy"=FALSE, "ChannelCnt"=0.0, "Initialized"=FALSE, "Current Channel"=0.0, "Initialized Channels"=[]}, {"Busy"=FALSE, "ChannelCnt"=0.0, "Initialized"=FALSE, "Current Channel"=0.0, "Initialized Channels"=[]}, {"Busy"=FALSE, "ChannelCnt"=0.0, "Initialized"=FALSE, "Current Channel"=0.0, "Initialized Channels"=[]}, {"Busy"=FALSE, "ChannelCnt"=0.0, "Initialized"=FALSE, "Current Channel"=0.0, "Initialized Channels"=[]}, {"Busy"=FALSE, "ChannelCnt"=0.0, "Initialized"=FALSE, "Current Channel"=0.0, "Initialized Channels"=[]}, {"Busy"=FALSE, "ChannelCnt"=0.0, "Initialized"=FALSE, "Current Channel"=0.0, "Initialized Channels"=[]}, {"Busy"=FALSE, "ChannelCnt"=0.0, "Initialized"=FALSE, "Current Channel"=0.0, "Initialized Channels"=[]}, {"Busy"=FALSE, "ChannelCnt"=0.0, "Initialized"=FALSE, "Current Channel"=0.0, "Initialized Channels"=[]}, {"Busy"=FALSE, "ChannelCnt"=0.0, "Initialized"=FALSE, "Current Channel"=0.0, "Initialized Channels"=[]}, {"Busy"=FALSE, "ChannelCnt"=0.0, "Initialized"=FALSE, "Current Channel"=0.0, "Initialized Channels"=[]}, {"Busy"=FALSE, "ChannelCnt"=0.0, "Initialized"=FALSE, "Current Channel"=0.0, "Initialized Channels"=[]}, {"Busy"=FALSE, "ChannelCnt"=0.0, "Initialized"=FALSE, "Current Channel"=0.0, "Initialized Channels"=[]}] ("Ismatec 4083 Global")) -> ()  [unwired: 1 in, 1 out]
      n6 = shared-variable ".\\Support Library.lvlib\\Globals.lvlib\\ASIA Pump Global"(T81 [{"Busy"=FALSE, "PumpCnt"=0.0, "RemoteEntered"=FALSE, "OverpressureSet"=FALSE}, {"Busy"=FALSE, "PumpCnt"=0.0, "RemoteEntered"=FALSE, "OverpressureSet"=FALSE}, {"Busy"=FALSE, "PumpCnt"=0.0, "RemoteEntered"=FALSE, "OverpressureSet"=FALSE}, {"Busy"=FALSE, "PumpCnt"=0.0, "RemoteEntered"=FALSE, "OverpressureSet"=FALSE}, {"Busy"=FALSE, "PumpCnt"=0.0, "RemoteEntered"=FALSE, "OverpressureSet"=FALSE}, {"Busy"=FALSE, "PumpCnt"=0.0, "RemoteEntered"=FALSE, "OverpressureSet"=FALSE}, {"Busy"=FALSE, "PumpCnt"=0.0, "RemoteEntered"=FALSE, "OverpressureSet"=FALSE}, {"Busy"=FALSE, "PumpCnt"=0.0, "RemoteEntered"=FALSE, "OverpressureSet"=FALSE}, {"Busy"=FALSE, "PumpCnt"=0.0, "RemoteEntered"=FALSE, "OverpressureSet"=FALSE}, {"Busy"=FALSE, "PumpCnt"=0.0, "RemoteEntered"=FALSE, "OverpressureSet"=FALSE}, {"Busy"=FALSE, "PumpCnt"=0.0, "RemoteEntered"=FALSE, "OverpressureSet"=FALSE}] ("ASIA Pump Global")) -> ()  [unwired: 1 in, 1 out]
      n7 = invoke class="Clust (strict)" method="Reinit To Default"() -> (error out=w92:errorcluster)  [unwired: 3 in, 2 out]
      n8 = Set Menu Item Info(7:w90, 9:TRUE ("enabled"), 10:w90, 11:w91) -> ()  [unwired: 3 in, 2 out]
    }
    frame #1 {
      n9 = disable-structure shown="Enabled" {
        frame Disabled {
          n10 = property on="Start Log" class="Bool"("Value"=FALSE) -> ()  [unwired: 2 in, 2 out]
        }
        frame Enabled {
        }
      }
    }
  }
  n11 = vi-ref "Dynamic Shared Variables.lvlib:Alarm History.vi"() -> (w61:refnum<vi>)
  n12 = call <vilib>:"Enable Alarm & Event Notifications.vi"() -> ("error out"=w44:errorcluster, "alarm & event notification"=w45:refnum<user-event>)  [unwired: 10 in]
  n13 = property class="VI"(reference=w61) -> ("Path"=w62:path)  [unwired: 1 in, 2 out]
  n14 = call "Create File.vi"("error in"=w39) -> ("error out"=w37:errorcluster)  [unwired: 10 in]
  n15 = Open VI Reference(type specifier VI Refnum (for type only)=refnum<vi> refnum, vi path=w62, options=128) -> (vi reference=w52:refnum<vi>, error out=w58:errorcluster)  [unwired: 3 in]
  n16 = register-events(error in=w44, w45) -> (reference out=w49:refnum<event-registration>, error out=w43:errorcluster)  [unwired: 1 in]
  n17 = call "Create User Event - Stop.vi"("error in (no error)"=w39) -> ("User Event - Stop"=w84:refnum<user-event>, "Stop Event Registration Refnum"=w48:refnum<event-registration>)  [unwired: 8 in, 1 out]
  n18 = call "Create Main Message Queues.vi"("error in (no error)"=w37, "Process Name"=w80) -> ("error out"=w81:errorcluster, "Message Queues out"=w29:T82)  [unwired: 8 in]
  n19 = Create User Event(user event datatype=w57, error in=w58) -> (user event=w51:refnum<user-event>)  [unwired: 1 out]
  n20 = Unbundle By Name(w29) -> ("UI"=w82:refnum<queue>, "DAQ"=w64:refnum<queue>, "Sequence"=w42:refnum<queue>, "CSV Log"=w41:refnum<queue>, "Sequence UI"=w31:refnum<queue>, "OPC UA Log"=w30:refnum<queue>, "Waveform Loop"=w24:refnum<queue>, "TDMS Log"=w23:refnum<queue>, "Graphs"=w22:refnum<queue>[], "TCP Write"=w21:refnum<queue>, "TCP Read"=w20:refnum<queue>, "OPC UA Log"=w19:refnum<queue>)
  n21 = call "Tag FGV.vi"("Operation"=Tag_FGV_Operation_Enum."Set Notification Queue", "Data"=w45, "error in (no error)"=w43) -> ()  [unwired: 5 in, 8 out]
  n22 = Current VI's Path() -> (path=w78:path)
  n23 = Bundle("Event Registration Refnum"=w49, "Stop Event Registration Refnum"=w48) -> (w47:T83)  [unwired: 1 in]
  n24 = Strip Path(path=w78) -> (stripped path=w68:path)  [unwired: 1 out]
  n25 = Build Path(base path=w68, name or relative path="History Graph") -> (appended path=w66:path)
  n26 = disable-structure shown="Enabled" {
    disable-tunnel: w29 -> [w97 w98]
    frame Disabled {
      n27 = call "OSIPI OPCUA Server.vi"("Main Queue Cluster"=w97) -> ()  [unwired: 11 in]
    }
    frame Enabled {
      n28 = call "OSIPI OPCUA Server Tag Version.vi"("Main Queue Cluster"=w98) -> ()  [unwired: 11 in]
    }
  }
  n29 = call "Sequence.vi"("Message Queues in"=w29) -> ("error out"=w32:errorcluster)  [unwired: 10 in]
  n30 = call "Waveform Loop.vi"("Message Queues out"=w29) -> ("error out"=w36:errorcluster)  [unwired: 10 in]
  n31 = call "TCP Write.vi"("Message Queues out"=w29) -> ()  [unwired: 11 in]
  n32 = call "TDMS Log Loop.vi"("Message Queues"=w29) -> ("error out"=w35:errorcluster)  [unwired: 10 in]
  n33 = call "DAQ Message Loop.vi"("Message Queues"=w29) -> ("error out"=w34:errorcluster)  [unwired: 10 in]
  n34 = call "CSV Log Loop.vi"("Message Queues"=w29) -> ("error out"=w33:errorcluster)  [unwired: 10 in]
  n35 = while {
    tunnel: w82 -> [w119]
    tunnel: w84 -> [w124]
    shift-right: [w117] -> w87
    shift-left: w81 -> [w123]
    tunnel: w80 -> [w115]
    tunnel: w29 -> [w114]
    shift-right: [w112] -> _
    shift-left: w40 -> [w113]
    tunnel: w29 -> [w111]
    tunnel: w64 -> [w108]
    tunnel: w42 -> [w107]
    tunnel: w41 -> [w105]
    tunnel: w31 -> [w109]
    tunnel: w30 -> [w106]
    tunnel: [w110] -> w28
    tunnel: [w108] -> w27
    tunnel: [w106] -> w26
    tunnel: [w105] -> w25
    tunnel: w24 -> [w104]
    tunnel: w23 -> [w103]
    tunnel: w22 -> [w102]
    tunnel: w21 -> [w101]
    tunnel: w20 -> [w100]
    tunnel: w19 -> [w99]
    tunnel: [w104] -> w18
    tunnel: [w103] -> w17
    tunnel: [w102] -> w16
    tunnel: [w101] -> w15
    tunnel: [w100] -> w14
    tunnel: [w99] -> w13
    stop <- w125 stop-if-true
    # "UI Message Loop"
    n36 = call "Dequeue Message.vi"("error in (no error)"=w123, "Message Queue"=w119) -> ("error out"=w122:errorcluster, "Message Data"=w120:variant, "Message"=w121:string, "dup Message Queue"=w116:refnum<queue>)  [unwired: 6 in]
    n37 = case "Message Cases" shown="\"Commit Config (AM)\"" w121 {
      selector: w121 -> [_ _ _ _ _ _ _ _ _ _ _ _ _ _ _ _ _ _ _ _ _ _ _ _ _ _ _ _ _ _ _ _ _ _ _ _ _ _ _ _ _ _ w1337 _ _ _ _ _ _ _ _ _ w1550 _]
      tunnel: w116 -> [_ _ _ _ _ _ _ _ _ _ _ _ _ _ _ _ _ w738 w762 w786 w810 w834 w858 w882 w906 w930 w954 w978 w1002 w1026 _ _ w1088 _ w1153 _ _ w1223 _ w1270 w1317 _ _ w1376 _ _ _ _ _ _ _ _ _ _]
      tunnel: w122 -> [w128 w136 w155 w200 w245 w290 w332 w375 w418 w461 w503 w546 w589 w633 w676 w720 w730 w737 w761 w785 w809 w833 w857 w881 w905 w929 w953 w977 w1001 w1025 w1049 w1080 w1095 w1136 _ w1175 w1210 w1222 w1259 w1283 _ w1327 w1343 w1379 w1457 w1463 w1475 w1507 w1511 w1516 w1541 w1547 _ w1559]
      tunnel: [w127 w129 w147 w192 w237 w282 w327 w370 w413 w456 w499 w542 w585 w629 w672 w714 w728 w735 w759 w783 w807 w831 w855 w879 w903 w927 w951 w975 w999 w1023 w1047 w1066 w1087 w1134 w1145 w1167 w1206 w1214 w1253 w1268 w1313 w1322 w1331 w1372 w1449 w1463 w1465 w1506 w1510 w1514 w1539 w1543 w1549 w1559] -> w118
      tunnel: [_ _ _ _ _ _ _ _ _ _ _ _ _ _ _ _ _ _ _ _ _ _ _ _ _ _ _ _ _ _ _ _ _ FALSE _ TRUE _ _ _ _ _ _ _ _ _ _ _ _ _ _ _ _ _ _] -> w125
      tunnel: w120 -> [_ w137 w156 w201 w246 w291 w333 w376 w419 w462 w504 w547 w590 w634 w677 w721 _ _ _ _ _ _ _ _ _ _ _ _ _ _ _ w1079 w1097 _ w1155 _ _ _ _ _ _ _ _ _ _ _ _ _ _ _ _ _ _ _]
      tunnel: w124 -> [_ _ _ _ _ _ _ _ _ _ _ _ _ _ _ _ _ _ _ _ _ _ _ _ _ _ _ _ _ _ _ _ _ _ _ w1191 _ _ _ _ _ _ _ _ _ _ _ _ _ _ _ _ _ _]
      tunnel: w115 -> [_ _ _ _ _ _ _ _ _ _ _ _ _ _ _ _ _ _ _ _ _ _ _ _ _ _ _ _ _ _ _ _ _ _ _ _ _ _ _ _ _ _ _ _ _ _ _ _ _ _ _ _ _ _]
      tunnel: w114 -> [_ _ _ _ _ _ _ _ _ _ _ _ _ _ _ _ _ _ _ _ _ _ _ _ _ _ _ _ _ _ _ _ _ _ _ _ _ _ _ _ _ _ _ _ _ _ _ _ _ _ _ _ _ _]
      tunnel: w113 -> [w126 w134 w146 w191 w236 w281 w326 w369 w412 w455 w498 w541 w584 w628 w671 w713 w732 w741 w765 w789 w813 w837 w861 w885 w909 w933 w957 w981 w1005 w1029 w1050 w1071 w1094 w1139 w1151 w1179 w1209 w1211 w1267 w1273 w1316 w1325 w1330 w1370 w1458 w1462 w1468 w1504 w1509 w1522 w1538 w1546 w1558 w1561]
      tunnel: [w126 w135 w145 w190 w235 w280 w325 w368 w411 w454 w497 w540 w583 w627 w670 w712 w732 w742 w766 w790 w814 w838 w862 w886 w910 w934 w958 w982 w1006 w1030 w1050 w1072 w1082 w1138 w1151 w1161 w1205 w1245 w1267 w1274 w1316 w1326 w1338 w1370 w1458 w1462 w1472 w1505 w1509 w1522 w1538 w1546 w1558 w1561] -> w112
      tunnel: w111 -> [_ _ _ _ _ _ _ _ _ _ _ _ _ _ _ _ _ _ _ _ _ _ _ _ _ _ _ _ _ _ _ _ _ _ _ w1190 _ _ _ _ _ _ _ w1382 w1460 _ _ _ w1512 _ _ _ _ _]
      tunnel: w108 -> [_ _ _ _ _ _ _ _ _ _ _ _ _ _ _ _ w733 _ _ _ _ _ _ _ _ _ _ _ _ _ _ _ _ _ _ _ _ _ w1263 w1269 _ _ _ _ _ _ _ _ _ _ _ _ _ _]
      tunnel: w107 -> [_ _ _ _ _ _ _ _ _ _ _ _ _ _ _ _ _ _ _ _ _ _ _ _ _ _ _ _ _ _ _ _ _ _ _ _ _ _ _ _ _ _ _ _ _ _ w1470 _ _ _ _ _ _ _]
      tunnel: w105 -> [_ _ _ _ _ _ _ _ _ _ _ _ _ _ _ _ _ _ _ _ _ _ _ _ _ _ _ _ _ _ _ _ _ _ _ _ _ _ _ _ _ _ _ _ _ _ _ _ _ _ _ w1548 _ _]
      tunnel: w109 -> [_ _ _ _ _ _ _ _ _ _ _ _ _ _ _ _ _ _ _ _ _ _ _ _ _ _ _ _ _ _ _ _ _ _ _ _ _ _ _ _ _ _ _ _ _ _ w1464 _ _ _ _ _ _ _]
      tunnel: w106 -> [_ _ _ _ _ _ _ _ _ _ _ _ _ _ _ _ _ _ _ _ _ _ _ _ _ _ _ _ _ _ _ _ _ _ _ _ _ _ _ _ _ _ _ w1371 _ _ _ _ _ _ _ _ _ _]
      frame "---Copy This Frame---" {
        # "Duplicate this frame when creating new messages.  Change this comment in the duplicated frame to describe this message."
        n38 = Merge Errors(w128) -> (w127:errorcluster)
      }
      frame "Commit Config (DAQ)" {
        # "Save DAQ Settings"
        n39 = Unbundle By Name(w134) -> ("Main Config.DAQ Config"=w133:T39)
        n40 = Variant To Data(error in=w136, type=w133, Variant=w137) -> (data=w131:T39, error out=w132:errorcluster)
        n41 = case shown="No Error" w132 {
          selector: w132 -> [w138 w143]
          tunnel: [w142 w144] -> w135
          tunnel: w134 -> [w141 w144]
          tunnel: w131 -> [w140 _]
          tunnel: [w138 w143] -> w129
          frame No Error {
            n42 = Bundle By Name(cluster=w141, "Main Config.DAQ Config"=w140, "Config Changed?"=TRUE) -> (w142:T1)
          }
          frame Error {
          }
        }
        n43 = call "Write to Log File.vi"("error in"=w129, "text"="Main: Commit Config (DAQ)") -> ()  [unwired: 9 in, 1 out]
      }
      frame "Commit Config (Feed Module)" {
        # "Save Feed Module Settings"
        n44 = Variant To Data(error in=w155, type=T18 {"GUID"="", "Drop Coords"={"Horizontal"=0, "Vertical"=0}, "Process Name"="", "Queue Name"="", "Settings"={"Cycle Period"=500.0, "Ismatech"={"VISA resource name"="", "Simulated?"=TRUE, "Pump Number"=1.0, "Reverse?"=FALSE}, "Masterflex"={"VISA resource name"="", "Simulated?"=TRUE, "Pump Number"=1.0, "Reverse?"=FALSE}, "Mettler"={"VISA resource name"="", "Simulated?"=FALSE}, "Bronkhorst M13 Flow Meter"={"VISA resource name"="", "Simulated?"=TRUE, "Smoothing Steps"=1}, "PID 2 Parameters"={"Input Device"=enum."Default", "Output Device"=enum."Default", "Setpoint"=0.0, "PID gains"={"proportional gain (Kc)"=1.0, "integral time (Ti, min)"=0.01, "derivative time (Td, min)"=0.0}}, "Manual Entry"=0.0, "Auto?"=TRUE, "output range"={"output high"=100.0, "output low"=0.0}, "Tacmina Settings"={"Analog DAQ Task"="", "Digital DAQ Task"=""}, "KNF SIMDOS Settings"={"VISA resource name"="", "Simulated?"=TRUE}, "ASIA Pump C"={"ASIA Pump #"=0, "channel"=0, "Simulated"=FALSE}, "VICI Settings"={"VISA resource name"="", "Simulated?"=TRUE, "Pump Letter"="", "Reverse?"=FALSE}, "FLOM Settings"={"VISA resource name"="", "Simulated?"=TRUE, "Pump Number"=0.0}, "SSI PR/LD Settings"={"VISA resource name"="", "Simulated?"=FALSE}, "Masterflex 75211 Settings"={"Analog DAQ Task"="", "Digital DAQ Task"=""}, "SSI P40 Settings"={"VISA resource name"="", "Simulated?"=TRUE}, "Ismatech 3 Channel Settings"={"VISA resource name"="", "Pump Number"=1, "Channel Number"=0, "Simulated?"=TRUE, "Reverse?"=FALSE}, "Bronkhorst M14 Settings"={"VISA resource name"="", "Simulated?"=FALSE, "Smoothing Steps"=1}}, "Settings Load Count"=0, "OP Load Count"=0} ("Feed Module Config"), Variant=w156) -> (data=w154:T18, error out=w150:errorcluster)
        n45 = Unbundle By Name(w154) -> ("GUID"=w151:string)
        n46 = Format Into String(format string="Could not save Feed Module config. No matching GUID for \"%s\"." ("error message (\"\")"), w151) -> (resulting string=w152:string)  [unwired: 2 in, 1 out]
        n47 = in-place {
          in-place-border: w154 -> [w163]
          in-place-border: w152 -> [w162]
          in-place-border: w151 -> [w161]
          in-place-border: w150 -> [w160]
          in-place-border: [w159] -> w147
          n48 = in-place-cluster #1(w146) -> ("Main Config.Feed Module Configs"=w158:T18[])
          n49 = Empty Array?(array=w158) -> (empty?=w164:bool)
          n50 = case shown="False" w164 {
            tunnel: w161 -> [w172 _]
            tunnel: w158 -> [w170 w189]
            tunnel: w163 -> [w169 w188]
            tunnel: [w168 w187] -> w157
            tunnel: w162 -> [w167 _]
            tunnel: w160 -> [w166 w186]
            tunnel: [w165 w186] -> w159
            frame False {
              n51 = for {
                tunnel: w170 -> [w185] mode=indexing
                tunnel: [w184] -> w173 mode=indexing
                n52 = Unbundle By Name(w185) -> ("GUID"=w184:string)
              }
              n53 = Search 1D Array(1D array=w173, element=w172) -> (index of element=w171:i32)  [unwired: 1 in]
              n54 = case shown="0, Default" w171 {
                selector: w171 -> [w177 _]
                tunnel: w170 -> [w178 w183]
                tunnel: w169 -> [w176 _]
                tunnel: [w175 w183] -> w168
                tunnel: w167 -> [_ w181]
                tunnel: w166 -> [w174 w180]
                tunnel: [w174 w179] -> w165
                frame 0, Default {
                  n55 = Replace Array Subset(array=w178, new element=w176, index=w177) -> (w175:T18[])
                }
                frame -1 {
                  n56 = call <vilib>:"Error Cluster From Error Code.vi"("error in (no error)"=w180, "error message (\"\")"=w181, "error code (0)"=7004) -> ("error out"=w179:errorcluster)  [unwired: 6 in]
                }
              }
            }
            frame True {
              n57 = Build Array (concatenate)(w189, w188) -> (w187:T18[])
            }
          }
          n58 = in-place-cluster #1("Main Config.Feed Module Configs"=w157) -> (w145:T1)
        }
        n59 = call "Write to Log File.vi"("error in"=w147, "text"="Main: Commit Config (Feed Module)") -> ()  [unwired: 9 in, 1 out]
      }
      frame "Commit Config (OPC Module)" {
        # "Save Feed Module Settings"
        n60 = Variant To Data(error in=w200, type=T8 {"State"=enum."Idle", "GUID"="", "Drop Coords"={"Horizontal"=0, "Vertical"=0}, "Configuration"={"Cycle Period"=500.0, "server endpoint URL"="opc.tcp://10.131.1.22:4840", "security policy"={"message mode"=enum."Sign", "security"=enum."Basic256"}, "Trust Any Server"=FALSE}, "First Iteration"=FALSE, "Data"=[], "Process Name"="", "Load Count"=0, "Log Started"=FALSE, "subscription ID out"=0, "OPC UA client refnum out"="", "Event Registration Refnum"=refnum, "Start Time"=timestamp(0 s since 1904-01-01), "Current Time"=timestamp(0 s since 1904-01-01), "Tag Data"=[]} ("OPC Module Config"), Variant=w201) -> (data=w199:T8, error out=w195:errorcluster)
        n61 = Unbundle By Name(w199) -> ("GUID"=w196:string)
        n62 = Format Into String(format string="Could not save OPCUA Module config. No matching GUID for \"%s\"." ("error message (\"\")"), w196) -> (resulting string=w197:string)  [unwired: 2 in, 1 out]
        n63 = in-place {
          in-place-border: w199 -> [w208]
          in-place-border: w197 -> [w207]
          in-place-border: w196 -> [w206]
          in-place-border: w195 -> [w205]
          in-place-border: [w204] -> w192
          n64 = in-place-cluster #2(w191) -> ("Main Config.OPC Module Configs"=w203:T8[])
          n65 = Empty Array?(array=w203) -> (empty?=w209:bool)
          n66 = case shown="False" w209 {
            tunnel: w206 -> [w217 _]
            tunnel: w203 -> [w215 w234]
            tunnel: w208 -> [w214 w233]
            tunnel: [w213 w232] -> w202
            tunnel: w207 -> [w212 _]
            tunnel: w205 -> [w211 w231]
            tunnel: [w210 w231] -> w204
            frame False {
              n67 = for {
                tunnel: w215 -> [w230] mode=indexing
                tunnel: [w229] -> w218 mode=indexing
                workers-P: _ -> [_]
                n68 = Unbundle By Name(w230) -> ("GUID"=w229:string)
              }
              n69 = Search 1D Array(1D array=w218, element=w217) -> (index of element=w216:i32)  [unwired: 1 in]
              n70 = case shown="0, Default" w216 {
                selector: w216 -> [w222 _]
                tunnel: w215 -> [w223 w228]
                tunnel: w214 -> [w221 _]
                tunnel: [w220 w228] -> w213
                tunnel: w212 -> [_ w226]
                tunnel: w211 -> [w219 w225]
                tunnel: [w219 w224] -> w210
                frame 0, Default {
                  n71 = Replace Array Subset(array=w223, new element=w221, index=w222) -> (w220:T8[])
                }
                frame -1 {
                  n72 = call <vilib>:"Error Cluster From Error Code.vi"("error in (no error)"=w225, "error message (\"\")"=w226, "error code (0)"=7004) -> ("error out"=w224:errorcluster)  [unwired: 6 in]
                }
              }
            }
            frame True {
              n73 = Build Array (concatenate)(w234, w233) -> (w232:T8[])
            }
          }
          n74 = in-place-cluster #2("Main Config.OPC Module Configs"=w202) -> (w190:T1)
        }
        n75 = call "Write to Log File.vi"("error in"=w192, "text"="Main: Commit Config (Feed Module)") -> ()  [unwired: 9 in, 1 out]
      }
      frame "Commit Config (Pump Module)" {
        # "Save Pump Module Settings"
        n76 = Variant To Data(error in=w245, type=T44 {"GUID"="", "Drop Coords"={"Horizontal"=0, "Vertical"=0}, "Process Name"="", "Queue Name"="", "Settings"={"Cycle Period"=500.0, "Manual Entry"=0.0, "Output Device"=enum."Default", "Ismatech"={"VISA resource name"="", "Simulated?"=TRUE, "Pump Number"=1.0, "Reverse?"=FALSE}, "Ismatech 3 Channel Settings"={"VISA resource name"="", "Pump Number"=1, "Channel Number"=0, "Simulated?"=TRUE, "Reverse?"=FALSE}, "Masterflex"={"VISA resource name"="", "Simulated?"=TRUE, "Pump Number"=1.0, "Reverse?"=FALSE}, "VICI Settings"={"VISA resource name"="", "Simulated?"=TRUE, "Pump Letter"="", "Reverse?"=FALSE}, "Tacmina Settings"={"Analog DAQ Task"="", "Digital DAQ Task"=""}, "KNF SIMDOS Settings"={"VISA resource name"="", "Simulated?"=TRUE}, "ASIA Pump C"={"ASIA Pump #"=0, "channel"=0, "Simulated"=FALSE}, "FLOM Settings"={"VISA resource name"="", "Simulated?"=TRUE, "Pump Number"=0.0}, "SSI PR/LD Settings"={"VISA resource name"="", "Simulated?"=FALSE}, "SSI P40 Settings"={"VISA resource name"="", "Simulated?"=FALSE}, "Masterflex 75211 Settings"={"Analog DAQ Task"="", "Digital DAQ Task"=""}, "Pump Calibration File"=path "", "Calibration Slope"=0.0, "Calibration Y Intercept"=0.0, "Pump Cal Enum"=0}, "Load Count"=0} ("Pump Module Config"), Variant=w246) -> (data=w239:T44, error out=w241:errorcluster)
        n77 = Unbundle By Name(w239) -> ("GUID"=w242:string)
        n78 = Format Into String(format string="Could not save Pump Module config. No matching GUID for \"%s\"." ("error message (\"\")"), w242) -> (resulting string=w243:string)  [unwired: 2 in, 1 out]
        n79 = in-place {
          in-place-border: w243 -> [w253]
          in-place-border: w242 -> [w252]
          in-place-border: w241 -> [w251]
          in-place-border: w239 -> [w250]
          in-place-border: [w249] -> w237
          n80 = in-place-cluster #3(w236) -> ("Main Config.Pump Module Configs"=w248:T44[])
          n81 = Empty Array?(array=w248) -> (empty?=w254:bool)
          n82 = case shown="True" w254 {
            tunnel: w252 -> [w262 _]
            tunnel: w248 -> [w260 w279]
            tunnel: w250 -> [w259 w276]
            tunnel: [w258 w278] -> w247
            tunnel: w253 -> [w257 _]
            tunnel: w251 -> [w256 w277]
            tunnel: [w255 w277] -> w249
            frame False {
              n83 = for {
                tunnel: w260 -> [w275] mode=indexing
                tunnel: [w274] -> w263 mode=indexing
                workers-P: _ -> [_]
                n84 = Unbundle By Name(w275) -> ("GUID"=w274:string)
              }
              n85 = Search 1D Array(1D array=w263, element=w262) -> (index of element=w261:i32)  [unwired: 1 in]
              n86 = case shown="0, Default" w261 {
                selector: w261 -> [w267 _]
                tunnel: w260 -> [w268 w273]
                tunnel: w259 -> [w264 _]
                tunnel: [w266 w273] -> w258
                tunnel: w257 -> [_ w271]
                tunnel: w256 -> [w265 w270]
                tunnel: [w265 w269] -> w255
                frame 0, Default {
                  n87 = Replace Array Subset(array=w268, new element=w264, index=w267) -> (w266:T44[])
                }
                frame -1 {
                  n88 = call <vilib>:"Error Cluster From Error Code.vi"("error in (no error)"=w270, "error message (\"\")"=w271, "error code (0)"=7004) -> ("error out"=w269:errorcluster)  [unwired: 6 in]
                }
              }
            }
            frame True {
              n89 = Build Array (concatenate)(w279, w276) -> (w278:T44[])
            }
          }
          n90 = in-place-cluster #3("Main Config.Pump Module Configs"=w247) -> (w235:T1)
        }
        n91 = call "Write to Log File.vi"("error in"=w237, "text"="Main: Commit Config (Pump Module)") -> ()  [unwired: 9 in, 1 out]
      }
      frame "Commit Config (DO)" {
        # "Save Digital Output Module Settings"
        n92 = Variant To Data(error in=w290, type=T59 {"GUID"="", "Drop Coords"={"Horizontal"=0, "Vertical"=0}, "Process Name"="", "Queue Name"="", "Settings"={"Valve Settings"={"D-O Settings"={"DAQmx Task Name"="", "Output Channel"=0, "Output Channel Names"=[]}, "VICI Electronic Actuator"={"VISA resource name"="", "Mode"=enum."Two Positions With Stops", "Simulated"=FALSE}}, "Valve Type"=enum."Default", "Time On (Sec)"=0.0, "Time Off (Sec)"=0.0, "Run?"=FALSE}, "Load Count"=0} ("D-O Module Config"), Variant=w291) -> (data=w289:T59, error out=w285:errorcluster)
        n93 = Unbundle By Name(w289) -> ("GUID"=w286:string)
        n94 = Format Into String(format string="Could not save Digital Out Module config. No matching GUID for \"%s\"." ("error message (\"\")"), w286) -> (resulting string=w287:string)  [unwired: 2 in, 1 out]
        n95 = in-place {
          in-place-border: w289 -> [w298]
          in-place-border: w287 -> [w297]
          in-place-border: w286 -> [w296]
          in-place-border: w285 -> [w295]
          in-place-border: [w294] -> w282
          n96 = in-place-cluster #4(w281) -> ("Main Config.DO Module Configs"=w293:T59[])
          n97 = Empty Array?(array=w293) -> (empty?=w299:bool)
          n98 = case shown="False" w299 {
            tunnel: w296 -> [w307 _]
            tunnel: w293 -> [w305 w324]
            tunnel: w298 -> [w304 w323]
            tunnel: [w303 w322] -> w292
            tunnel: w297 -> [w302 _]
            tunnel: w295 -> [w301 w321]
            tunnel: [w300 w321] -> w294
            frame False {
              n99 = for {
                tunnel: w305 -> [w320] mode=indexing
                tunnel: [w319] -> w308 mode=indexing
                workers-P: _ -> [_]
                n100 = Unbundle By Name(w320) -> ("GUID"=w319:string)
              }
              n101 = Search 1D Array(1D array=w308, element=w307) -> (index of element=w306:i32)  [unwired: 1 in]
              n102 = case shown="0, Default" w306 {
                selector: w306 -> [w312 _]
                tunnel: w305 -> [w313 w318]
                tunnel: w304 -> [w311 _]
                tunnel: [w310 w318] -> w303
                tunnel: w302 -> [_ w316]
                tunnel: w301 -> [w309 w315]
                tunnel: [w309 w314] -> w300
                frame 0, Default {
                  n103 = Replace Array Subset(array=w313, new element=w311, index=w312) -> (w310:T59[])
                }
                frame -1 {
                  n104 = call <vilib>:"Error Cluster From Error Code.vi"("error in (no error)"=w315, "error message (\"\")"=w316, "error code (0)"=7004) -> ("error out"=w314:errorcluster)  [unwired: 6 in]
                }
              }
            }
            frame True {
              n105 = Build Array (concatenate)(w324, w323) -> (w322:T59[])
            }
          }
          n106 = in-place-cluster #4("Main Config.DO Module Configs"=w292) -> (w280:T1)
        }
        n107 = call "Write to Log File.vi"("error in"=w282, "text"="Main: Commit Config (DO)") -> ()  [unwired: 9 in, 1 out]
      }
      frame "Commit Config (PR Module)" {
        # "Save Pressure Regulator Module Settings"
        n108 = Variant To Data(error in=w332, type=T64 {"GUID"="", "Drop Coords"={"Horizontal"=0, "Vertical"=0}, "Process Name"="", "Queue Name"="", "Settings"={"Cycle Period"=500.0, "PID 2 Parameters"={"Input Device"=enum."Default", "Output Device"=enum."Default", "Setpoint"=0.0, "PID gains"={"proportional gain (Kc)"=1.0, "integral time (Ti, min)"=0.01, "derivative time (Td, min)"=0.0}, "output range"={"output low"=0.0, "output high"=100.0}}, "Manual Entry"=0.0, "Auto?"=TRUE, "4-20mA Input Settings"={"Input Channel "=0}, "4-20mA Out Settings"={"Output DAQ Task"=""}, "Input Channel Tag Name "=""}, "Settings Load Count"=0} ("Feed Module Config"), Variant=w333) -> (data=w331:T64, error out=w330:errorcluster)
        n109 = in-place {
          in-place-border: w331 -> [w341]
          in-place-border: w330 -> [w337]
          in-place-border: [w336] -> w327
          n110 = in-place-cluster #5(w326) -> ("Main Config.PR Module Configs"=w335:T64[])
          n111 = Unbundle By Name(w341) -> ("GUID"=w338:string)
          n112 = Empty Array?(array=w335) -> (empty?=w342:bool)
          n113 = Format Into String(format string="Could not save Digital Out Module config. No matching GUID for \"%s\"." ("error message (\"\")"), w338) -> (resulting string=w339:string)  [unwired: 2 in, 1 out]
          n114 = case shown="True" w342 {
            tunnel: w338 -> [w350 _]
            tunnel: w335 -> [w348 w367]
            tunnel: w341 -> [w347 w364]
            tunnel: [w346 w366] -> w334
            tunnel: w339 -> [w345 _]
            tunnel: w337 -> [w344 w365]
            tunnel: [w343 w365] -> w336
            frame False {
              n115 = for {
                tunnel: w348 -> [w363] mode=indexing
                tunnel: [w362] -> w351 mode=indexing
                workers-P: _ -> [_]
                n116 = Unbundle By Name(w363) -> ("GUID"=w362:string)
              }
              n117 = Search 1D Array(1D array=w351, element=w350) -> (index of element=w349:i32)  [unwired: 1 in]
              n118 = case shown="-1" w349 {
                selector: w349 -> [w355 _]
                tunnel: w348 -> [w356 w361]
                tunnel: w347 -> [w354 _]
                tunnel: [w353 w361] -> w346
                tunnel: w345 -> [_ w359]
                tunnel: w344 -> [w352 w358]
                tunnel: [w352 w357] -> w343
                frame 0, Default {
                  n119 = Replace Array Subset(array=w356, new element=w354, index=w355) -> (w353:T64[])
                }
                frame -1 {
                  n120 = call <vilib>:"Error Cluster From Error Code.vi"("error in (no error)"=w358, "error message (\"\")"=w359, "error code (0)"=7004) -> ("error out"=w357:errorcluster)  [unwired: 6 in]
                }
              }
            }
            frame True {
              n121 = Build Array (concatenate)(w367, w364) -> (w366:T64[])
            }
          }
          n122 = in-place-cluster #5("Main Config.PR Module Configs"=w334) -> (w325:T1)
        }
        n123 = call "Write to Log File.vi"("error in"=w327, "text"="Main: Commit Config (PR Module)") -> ()  [unwired: 9 in, 1 out]
      }
      frame "Commit Config (TCU Module)" {
        # "Save Temperature Control Unit Module Settings"
        n124 = Variant To Data(error in=w375, type=T50 {"GUID"="", "Drop Coords"={"Horizontal"=0, "Vertical"=0}, "Process Name"="", "Queue Name"="", "Settings"={"Cycle Period"=500.0, "Setpoint Entry"=0.0, "Output Device"=enum."Default", "Huber Ministat 230 Settings"={"VISA resource name"="", "Simulated?"=FALSE}, "Lauda Settings"={"VISA resource name"="", "Simulated?"=FALSE, "Pump Power"=2}, "Julabo FP-50 Settings"={"VISA resource name"="", "Simulated?"=FALSE, "Pump Power"=2}, "Internal Control?"=FALSE, "Huber Unistat 410 Settings"={"VISA resource name"="", "Address"=0, "Simulated?"=FALSE}}, "Load Count"=0, "Power Level Changed"=FALSE} ("TCU Module Config"), Variant=w376) -> (data=w374:T50, error out=w373:errorcluster)
        n125 = in-place {
          in-place-border: w374 -> [w384]
          in-place-border: w373 -> [w380]
          in-place-border: [w379] -> w370
          n126 = in-place-cluster #6(w369) -> ("Main Config.TCU Module Configs"=w378:T50[])
          n127 = Unbundle By Name(w384) -> ("GUID"=w381:string)
          n128 = Empty Array?(array=w378) -> (empty?=w385:bool)
          n129 = Format Into String(format string="Could not save TCU Module config. No matching GUID for \"%s\"." ("error message (\"\")"), w381) -> (resulting string=w382:string)  [unwired: 2 in, 1 out]
          n130 = case shown="False" w385 {
            tunnel: w381 -> [w393 _]
            tunnel: w378 -> [w391 w410]
            tunnel: w384 -> [w390 w409]
            tunnel: [w389 w408] -> w377
            tunnel: w382 -> [w388 _]
            tunnel: w380 -> [w387 w407]
            tunnel: [w386 w407] -> w379
            frame False {
              n131 = for {
                tunnel: w391 -> [w406] mode=indexing
                tunnel: [w405] -> w394 mode=indexing
                workers-P: _ -> [_]
                n132 = Unbundle By Name(w406) -> ("GUID"=w405:string)
              }
              n133 = Search 1D Array(1D array=w394, element=w393) -> (index of element=w392:i32)  [unwired: 1 in]
              n134 = case shown="0, Default" w392 {
                selector: w392 -> [w398 _]
                tunnel: w391 -> [w399 w404]
                tunnel: w390 -> [w397 _]
                tunnel: [w396 w404] -> w389
                tunnel: w388 -> [_ w402]
                tunnel: w387 -> [w395 w401]
                tunnel: [w395 w400] -> w386
                frame 0, Default {
                  n135 = Replace Array Subset(array=w399, new element=w397, index=w398) -> (w396:T50[])
                }
                frame -1 {
                  n136 = call <vilib>:"Error Cluster From Error Code.vi"("error in (no error)"=w401, "error message (\"\")"=w402, "error code (0)"=7004) -> ("error out"=w400:errorcluster)  [unwired: 6 in]
                }
              }
            }
            frame True {
              n137 = Build Array (concatenate)(w410, w409) -> (w408:T50[])
            }
          }
          n138 = in-place-cluster #6("Main Config.TCU Module Configs"=w377) -> (w368:T1)
        }
        n139 = call "Write to Log File.vi"("error in"=w370, "text"="Main: Commit Config (TCU)") -> ()  [unwired: 9 in, 1 out]
      }
      frame "Commit Config (Scale Module)" {
        w415 = T42 {"GUID"="", "Drop Coords"={"Horizontal"=0, "Vertical"=0}, "Process Name"="", "Queue Name"="", "Settings"={"Cycle Period"=500.0, "Mettler"={"VISA resource name"="", "Simulated?"=FALSE}, "Scale Type"=""}, "Load Count"=0}  # Scale Module Config
        # "Save Scale Module Settings"
        n140 = Variant To Data(error in=w418, type=w415, Variant=w419) -> (data=w417:T42, error out=w416:errorcluster)
        n141 = in-place {
          in-place-border: w417 -> [w427]
          in-place-border: w416 -> [w423]
          in-place-border: [w422] -> w413
          n142 = in-place-cluster #7(w412) -> ("Main Config.Scale Module Configs"=w421:T42[])
          n143 = Unbundle By Name(w427) -> ("GUID"=w424:string)
          n144 = Empty Array?(array=w421) -> (empty?=w428:bool)
          n145 = Format Into String(format string="Could not save Scale Module config. No matching GUID for \"%s\"." ("error message (\"\")"), w424) -> (resulting string=w425:string)  [unwired: 2 in, 1 out]
          n146 = case shown="True" w428 {
            tunnel: w424 -> [w436 _]
            tunnel: w421 -> [w434 w453]
            tunnel: w427 -> [w433 w452]
            tunnel: [w432 w451] -> w420
            tunnel: w425 -> [w431 _]
            tunnel: w423 -> [w430 w450]
            tunnel: [w429 w450] -> w422
            frame False {
              n147 = for {
                tunnel: w434 -> [w449] mode=indexing
                tunnel: [w448] -> w437 mode=indexing
                workers-P: _ -> [_]
                n148 = Unbundle By Name(w449) -> ("GUID"=w448:string)
              }
              n149 = Search 1D Array(1D array=w437, element=w436) -> (index of element=w435:i32)  [unwired: 1 in]
              n150 = case shown="0, Default" w435 {
                selector: w435 -> [w441 _]
                tunnel: w434 -> [w442 w447]
                tunnel: w433 -> [w440 _]
                tunnel: [w439 w447] -> w432
                tunnel: w431 -> [_ w445]
                tunnel: w430 -> [w438 w444]
                tunnel: [w438 w443] -> w429
                frame 0, Default {
                  n151 = Replace Array Subset(array=w442, new element=w440, index=w441) -> (w439:T42[])
                }
                frame -1 {
                  n152 = call <vilib>:"Error Cluster From Error Code.vi"("error in (no error)"=w444, "error message (\"\")"=w445, "error code (0)"=7004) -> ("error out"=w443:errorcluster)  [unwired: 6 in]
                }
              }
            }
            frame True {
              n153 = Build Array (concatenate)(w453, w452) -> (w451:T42[])
            }
          }
          n154 = in-place-cluster #7("Main Config.Scale Module Configs"=w420) -> (w411:T1)
        }
        n155 = call "Write to Log File.vi"("error in"=w413, "text"="Main: Commit Config (Scale Module)") -> ()  [unwired: 9 in, 1 out]
      }
      frame "Commit Config (Flow Module)" {
        w458 = T48 {"GUID"="", "Drop Coords"={"Horizontal"=0, "Vertical"=0}, "Process Name"="", "Queue Name"="", "Settings"={"Cycle Period"=500.0, "Flow Meter Type"="", "Bronkhorst M13 Settings"={"VISA resource name"="", "Simulated?"=FALSE, "Smoothing Steps"=1}, "Bronkhorst M14 Settings"={"VISA resource name"="", "Simulated?"=FALSE, "Smoothing Steps"=1}}, "Load Count"=0}  # Flow Module Config
        # "Save Flow Module Settings"
        n156 = Variant To Data(error in=w461, type=w458, Variant=w462) -> (data=w460:T48, error out=w459:errorcluster)
        n157 = in-place {
          in-place-border: w460 -> [w470]
          in-place-border: w459 -> [w466]
          in-place-border: [w465] -> w456
          n158 = in-place-cluster #8(w455) -> ("Main Config.Flow Module Configs"=w463:T48[])
          n159 = Unbundle By Name(w470) -> ("GUID"=w467:string)
          n160 = Empty Array?(array=w463) -> (empty?=w471:bool)
          n161 = Format Into String(format string="Could not save Scale Module config. No matching GUID for \"%s\"." ("error message (\"\")"), w467) -> (resulting string=w468:string)  [unwired: 2 in, 1 out]
          n162 = case shown="True" w471 {
            tunnel: w467 -> [w479 _]
            tunnel: w463 -> [w477 w496]
            tunnel: w470 -> [w476 w495]
            tunnel: [w475 w494] -> w464
            tunnel: w468 -> [w474 _]
            tunnel: w466 -> [w473 w493]
            tunnel: [w472 w493] -> w465
            frame False {
              n163 = for {
                tunnel: w477 -> [w492] mode=indexing
                tunnel: [w491] -> w480 mode=indexing
                workers-P: _ -> [_]
                n164 = Unbundle By Name(w492) -> ("GUID"=w491:string)
              }
              n165 = Search 1D Array(1D array=w480, element=w479) -> (index of element=w478:i32)  [unwired: 1 in]
              n166 = case shown="0, Default" w478 {
                selector: w478 -> [w484 _]
                tunnel: w477 -> [w485 w490]
                tunnel: w476 -> [w483 _]
                tunnel: [w482 w490] -> w475
                tunnel: w474 -> [_ w488]
                tunnel: w473 -> [w481 w487]
                tunnel: [w481 w486] -> w472
                frame 0, Default {
                  n167 = Replace Array Subset(array=w485, new element=w483, index=w484) -> (w482:T48[])
                }
                frame -1 {
                  n168 = call <vilib>:"Error Cluster From Error Code.vi"("error in (no error)"=w487, "error message (\"\")"=w488, "error code (0)"=7004) -> ("error out"=w486:errorcluster)  [unwired: 6 in]
                }
              }
            }
            frame True {
              n169 = Build Array (concatenate)(w496, w495) -> (w494:T48[])
            }
          }
          n170 = in-place-cluster #8("Main Config.Flow Module Configs"=w464) -> (w454:T1)
        }
        n171 = call "Write to Log File.vi"("error in"=w456, "text"="Main: Commit Config (Flow Module)") -> ()  [unwired: 9 in, 1 out]
      }
      frame "Commit Config (TT)" {
        # "Save Temperature Transmitter Module Settings"
        n172 = Variant To Data(error in=w503, type=T37 {"GUID"="", "Drop Coords"={"Horizontal"=0, "Vertical"=0}, "Input Channel Tag Name "="", "Process Name"="", "Queue Name"="", "Input Channel Numeric Alarm Settings"=[]} ("TT Module Config"), Variant=w504) -> (data=w502:T37, error out=w501:errorcluster)
        n173 = in-place {
          in-place-border: w502 -> [w513]
          in-place-border: w501 -> [w509]
          in-place-border: [w508] -> w499
          n174 = in-place-cluster #9(w498) -> ("Main Config.TT Module Configs"=w506:T37[])
          n175 = Unbundle By Name(w513) -> ("GUID"=w510:string)
          n176 = Empty Array?(array=w506) -> (empty?=w514:bool)
          n177 = Format Into String(format string="Could not save TT Module config. No matching GUID for \"%s\"." ("error message (\"\")"), w510) -> (resulting string=w511:string)  [unwired: 2 in, 1 out]
          n178 = case shown="True" w514 {
            tunnel: w510 -> [w522 _]
            tunnel: w506 -> [w520 w539]
            tunnel: w513 -> [w519 w538]
            tunnel: [w518 w537] -> w507
            tunnel: w511 -> [w517 _]
            tunnel: w509 -> [w516 w536]
            tunnel: [w515 w536] -> w508
            frame False {
              n179 = for {
                tunnel: w520 -> [w535] mode=indexing
                tunnel: [w534] -> w523 mode=indexing
                workers-P: _ -> [_]
                n180 = Unbundle By Name(w535) -> ("GUID"=w534:string)
              }
              n181 = Search 1D Array(1D array=w523, element=w522) -> (index of element=w521:i32)  [unwired: 1 in]
              n182 = case shown="0, Default" w521 {
                selector: w521 -> [w527 _]
                tunnel: w520 -> [w528 w533]
                tunnel: w519 -> [w526 _]
                tunnel: [w525 w533] -> w518
                tunnel: w517 -> [_ w531]
                tunnel: w516 -> [w524 w530]
                tunnel: [w524 w529] -> w515
                frame 0, Default {
                  n183 = Replace Array Subset(array=w528, new element=w526, index=w527) -> (w525:T37[])
                }
                frame -1 {
                  n184 = call <vilib>:"Error Cluster From Error Code.vi"("error in (no error)"=w530, "error message (\"\")"=w531, "error code (0)"=7003) -> ("error out"=w529:errorcluster)  [unwired: 6 in]
                }
              }
            }
            frame True {
              n185 = Build Array (concatenate)(w539, w538) -> (w537:T37[])
            }
          }
          n186 = in-place-cluster #9("Main Config.TT Module Configs"=w507) -> (w497:T1)
        }
        n187 = call "Write to Log File.vi"("error in"=w499, "text"="Main: Commit Config (TT)") -> ()  [unwired: 9 in, 1 out]
      }
      frame "Commit Config (PT)" {
        # "Save Pressure Transmitter Module Settings"
        n188 = Variant To Data(error in=w546, type=T41 {"GUID"="", "Drop Coords"={"Horizontal"=0, "Vertical"=0}, "Input Channel Tag Name "="", "Process Name"="", "Queue Name"="", "Input Channel Numeric Alarm Settings"=[]} ("TT Module Config"), Variant=w547) -> (data=w545:T41, error out=w544:errorcluster)
        n189 = in-place {
          in-place-border: w545 -> [w556]
          in-place-border: w544 -> [w552]
          in-place-border: [w551] -> w542
          n190 = in-place-cluster #10(w541) -> ("Main Config.PT Module Configs"=w550:T41[])
          n191 = Unbundle By Name(w556) -> ("GUID"=w553:string)
          n192 = Empty Array?(array=w550) -> (empty?=w557:bool)
          n193 = Format Into String(format string="Could not save PT Module config. No matching GUID for \"%s\"." ("error message (\"\")"), w553) -> (resulting string=w554:string)  [unwired: 2 in, 1 out]
          n194 = case shown="True" w557 {
            tunnel: w553 -> [w565 _]
            tunnel: w550 -> [w563 w582]
            tunnel: w556 -> [w562 w581]
            tunnel: [w561 w580] -> w549
            tunnel: w554 -> [w560 _]
            tunnel: w552 -> [w559 w579]
            tunnel: [w558 w579] -> w551
            frame False {
              n195 = for {
                tunnel: w563 -> [w578] mode=indexing
                tunnel: [w577] -> w566 mode=indexing
                workers-P: _ -> [_]
                n196 = Unbundle By Name(w578) -> ("GUID"=w577:string)
              }
              n197 = Search 1D Array(1D array=w566, element=w565) -> (index of element=w564:i32)  [unwired: 1 in]
              n198 = case shown="0, Default" w564 {
                selector: w564 -> [w570 _]
                tunnel: w563 -> [w571 w576]
                tunnel: w562 -> [w569 _]
                tunnel: [w568 w576] -> w561
                tunnel: w560 -> [_ w574]
                tunnel: w559 -> [w567 w573]
                tunnel: [w567 w572] -> w558
                frame 0, Default {
                  n199 = Replace Array Subset(array=w571, new element=w569, index=w570) -> (w568:T41[])
                }
                frame -1 {
                  n200 = call <vilib>:"Error Cluster From Error Code.vi"("error in (no error)"=w573, "error message (\"\")"=w574, "error code (0)"=7005) -> ("error out"=w572:errorcluster)  [unwired: 6 in]
                }
              }
            }
            frame True {
              n201 = Build Array (concatenate)(w582, w581) -> (w580:T41[])
            }
          }
          n202 = in-place-cluster #10("Main Config.PT Module Configs"=w549) -> (w540:T1)
        }
        n203 = call "Write to Log File.vi"("error in"=w542, "text"="Main: Commit Config (PT)") -> ()  [unwired: 9 in, 1 out]
      }
      frame "Commit Config (U3)" {
        # "Save LabJack U3 Module Settings"
        n204 = Variant To Data(error in=w589, type=T46 {"GUID"="", "Drop Coords"={"Horizontal"=0, "Vertical"=0}, "AI Channel Number"=enum."Default", "Process Name"="", "Queue Name"="", "Input Channel Numeric Alarm Settings"=[]} ("TT Module Config"), Variant=w590) -> (data=w588:T46, error out=w587:errorcluster)
        n205 = in-place {
          in-place-border: w588 -> [w599]
          in-place-border: w587 -> [w595]
          in-place-border: [w594] -> w585
          n206 = in-place-cluster #11(w584) -> ("Main Config.U3 Module Configs"=w593:T46[])
          n207 = Unbundle By Name(w599) -> ("GUID"=w596:string)
          n208 = Empty Array?(array=w593) -> (empty?=w600:bool)
          n209 = Format Into String(format string="Could not save U3 Module config. No matching GUID for \"%s\"." ("error message (\"\")"), w596) -> (resulting string=w597:string)  [unwired: 2 in, 1 out]
          n210 = case shown="True" w600 {
            tunnel: w596 -> [w608 _]
            tunnel: w593 -> [w606 w625]
            tunnel: w599 -> [w605 w624]
            tunnel: [w604 w623] -> w592
            tunnel: w597 -> [w603 _]
            tunnel: w595 -> [w602 w622]
            tunnel: [w601 w622] -> w594
            frame False {
              n211 = for {
                tunnel: w606 -> [w621] mode=indexing
                tunnel: [w620] -> w609 mode=indexing
                workers-P: _ -> [_]
                n212 = Unbundle By Name(w621) -> ("GUID"=w620:string)
              }
              n213 = Search 1D Array(1D array=w609, element=w608) -> (index of element=w607:i32)  [unwired: 1 in]
              n214 = case shown="-1" w607 {
                selector: w607 -> [w613 _]
                tunnel: w606 -> [w614 w619]
                tunnel: w605 -> [w612 _]
                tunnel: [w611 w619] -> w604
                tunnel: w603 -> [_ w617]
                tunnel: w602 -> [w610 w616]
                tunnel: [w610 w615] -> w601
                frame 0, Default {
                  n215 = Replace Array Subset(array=w614, new element=w612, index=w613) -> (w611:T46[])
                }
                frame -1 {
                  n216 = call <vilib>:"Error Cluster From Error Code.vi"("error in (no error)"=w616, "error message (\"\")"=w617, "error code (0)"=7005) -> ("error out"=w615:errorcluster)  [unwired: 6 in]
                }
              }
            }
            frame True {
              n217 = Build Array (concatenate)(w625, w624) -> (w623:T46[])
            }
          }
          n218 = in-place-cluster #11("Main Config.U3 Module Configs"=w592) -> (w583:T1)
        }
        n219 = call "Write to Log File.vi"("error in"=w585, "text"="Main: Commit Config (U3)") -> ()  [unwired: 9 in, 1 out]
      }
      frame "Commit Config (SC)" {
        # "Save Sonicator Module Settings"
        n220 = Variant To Data(error in=w633, type=T68 {"GUID"="", "Drop Coords"={"Horizontal"=0, "Vertical"=0}, "Process Name"="", "Queue Name"="", "Settings"={"Cycle Period"=500.0, "Sonicator Type"="", "SS P100 Settings"={"VISA resource name"="", "Simulated?"=FALSE}, "Setpoint (µm)"=0.0, "Cutoff (W)"=0.0}, "Load Count"=0} ("Scale Module Config"), Variant=w634) -> (data=w632:T68, error out=w631:errorcluster)
        n221 = in-place {
          in-place-border: w632 -> [w642]
          in-place-border: w631 -> [w638]
          in-place-border: [w637] -> w629
          n222 = in-place-cluster #12(w628) -> ("Main Config.SC Module Configs"=w636:T68[])
          n223 = Unbundle By Name(w642) -> ("GUID"=w639:string)
          n224 = Empty Array?(array=w636) -> (empty?=w643:bool)
          n225 = Format Into String(format string="Could not save SC Module config. No matching GUID for \"%s\"." ("error message (\"\")"), w639) -> (resulting string=w640:string)  [unwired: 2 in, 1 out]
          n226 = case shown="True" w643 {
            tunnel: w639 -> [w651 _]
            tunnel: w636 -> [w649 w668]
            tunnel: w642 -> [w648 w667]
            tunnel: [w647 w666] -> w635
            tunnel: w640 -> [w646 _]
            tunnel: w638 -> [w645 w665]
            tunnel: [w644 w665] -> w637
            frame False {
              n227 = for {
                tunnel: w649 -> [w664] mode=indexing
                tunnel: [w663] -> w652 mode=indexing
                workers-P: _ -> [_]
                n228 = Unbundle By Name(w664) -> ("GUID"=w663:string)
              }
              n229 = Search 1D Array(1D array=w652, element=w651) -> (index of element=w650:i32)  [unwired: 1 in]
              n230 = case shown="-1" w650 {
                selector: w650 -> [w656 _]
                tunnel: w649 -> [w657 w662]
                tunnel: w648 -> [w655 _]
                tunnel: [w654 w662] -> w647
                tunnel: w646 -> [_ w660]
                tunnel: w645 -> [w653 w659]
                tunnel: [w653 w658] -> w644
                frame 0, Default {
                  n231 = Replace Array Subset(array=w657, new element=w655, index=w656) -> (w654:T68[])
                }
                frame -1 {
                  n232 = call <vilib>:"Error Cluster From Error Code.vi"("error in (no error)"=w659, "error message (\"\")"=w660, "error code (0)"=7005) -> ("error out"=w658:errorcluster)  [unwired: 6 in]
                }
              }
            }
            frame True {
              n233 = Build Array (concatenate)(w668, w667) -> (w666:T68[])
            }
          }
          n234 = in-place-cluster #12("Main Config.SC Module Configs"=w635) -> (w627:T1)
        }
        n235 = call "Write to Log File.vi"("error in"=w629, "text"="Main: Commit Config (SC)") -> ()  [unwired: 9 in, 1 out]
      }
      frame "Commit Config (AM)" {
        # "Save Agitator Module Settings"
        n236 = Variant To Data(error in=w676, type=T71 {"GUID"="", "Drop Coords"={"Horizontal"=0, "Vertical"=0}, "Process Name"="", "Queue Name"="", "Settings"={"Cycle Period"=500.0, "Agitator Type"="", "Setpoint (µm)"=0.0}, "Load Count"=0} ("Agitator Module Config"), Variant=w677) -> (data=w675:T71, error out=w674:errorcluster)
        n237 = in-place {
          in-place-border: w675 -> [w685]
          in-place-border: w674 -> [w681]
          in-place-border: [w680] -> w672
          n238 = in-place-cluster #13(w671) -> ("Main Config.AM Module Configs"=w679:T71[])
          n239 = Unbundle By Name(w685) -> ("GUID"=w682:string)
          n240 = Empty Array?(array=w679) -> (empty?=w686:bool)
          n241 = Format Into String(format string="Could not save Agitator Module config. No matching GUID for \"%s\"." ("error message (\"\")"), w682) -> (resulting string=w683:string)  [unwired: 2 in, 1 out]
          n242 = case shown="False" w686 {
            tunnel: w682 -> [w694 _]
            tunnel: w679 -> [w692 w711]
            tunnel: w685 -> [w691 w710]
            tunnel: [w690 w709] -> w678
            tunnel: w683 -> [w689 _]
            tunnel: w681 -> [w688 w708]
            tunnel: [w687 w708] -> w680
            frame False {
              n243 = for {
                tunnel: w692 -> [w707] mode=indexing
                tunnel: [w706] -> w695 mode=indexing
                workers-P: _ -> [_]
                n244 = Unbundle By Name(w707) -> ("GUID"=w706:string)
              }
              n245 = Search 1D Array(1D array=w695, element=w694) -> (index of element=w693:i32)  [unwired: 1 in]
              n246 = case shown="0, Default" w693 {
                selector: w693 -> [w699 _]
                tunnel: w692 -> [w700 w705]
                tunnel: w691 -> [w698 _]
                tunnel: [w697 w705] -> w690
                tunnel: w689 -> [_ w703]
                tunnel: w688 -> [w696 w702]
                tunnel: [w696 w701] -> w687
                frame 0, Default {
                  n247 = Replace Array Subset(array=w700, new element=w698, index=w699) -> (w697:T71[])
                }
                frame -1 {
                  n248 = call <vilib>:"Error Cluster From Error Code.vi"("error in (no error)"=w702, "error message (\"\")"=w703, "error code (0)"=7005) -> ("error out"=w701:errorcluster)  [unwired: 6 in]
                }
              }
            }
            frame True {
              n249 = Build Array (concatenate)(w711, w710) -> (w709:T71[])
            }
          }
          n250 = in-place-cluster #13("Main Config.AM Module Configs"=w678) -> (w670:T1)
        }
        n251 = call "Write to Log File.vi"("error in"=w672, "text"="Main: Commit Config (SC)") -> ()  [unwired: 9 in, 1 out]
      }
      frame "Delete Module" {
        w722 = ""  # GUID
        # "This message is called when a user deletes a module from the canvas. The GUID for the module is passed here and we delete it from the list."
        n252 = Variant To Data(error in=w720, type=w722, Variant=w721) -> (data=w717:string, error out=w719:errorcluster)
        n253 = in-place {
          in-place-border: w719 -> [w727]
          in-place-border: w717 -> [w726]
          in-place-border: [w725] -> w714
          n254 = in-place-cluster #14(w713) -> ("Main Config"=w724:T7)
          n255 = call "Delete GUID Module.vi"("error in (no error)"=w727, "GUID"=w726, "Main Config in"=w724) -> ("error out"=w725:errorcluster, "Main Config out"=w723:T7)  [unwired: 7 in]
          n256 = in-place-cluster #14("Main Config"=w723) -> (w712:T1)
        }
        n257 = Concatenate Strings("Main: GUID " ("string"), w717, " Deleted" ("string")) -> (w718:string)
        n258 = call "Write to Log File.vi"("error in"=w714, "text"=w718) -> ()  [unwired: 9 in, 1 out]
      }
      frame "Update Config (DAQ)" {
        n259 = Unbundle By Name(w732) -> ("Main Config.DAQ Config"=w731:T39)
        n260 = call-poly "Enqueue Message.vi"("error in (no error)"=w730, "Message Data"=w731, "Message"="DAQ-Update Settings", "Message Queue"=w733) -> ("error out"=w728:errorcluster)  [unwired: 6 in, 1 out]
        n261 = call "Write to Log File.vi"("error in"=w728, "text"="Main: Update Config (DAQ)") -> ()  [unwired: 9 in, 1 out]
      }
      frame "Update Config (TT)" {
        # "Create TT Modules and \"drop\" them on the Picture Control and assign configs"
        n262 = Unbundle By Name(w741) -> ("Main Config.TT Module Configs"=w740:T37[])
        n263 = property class="VI"() -> ("Front Panel.Title"=w739:string)  [unwired: 2 in, 2 out]
        n264 = for {
          shift-right: [w758] -> w742
          shift-left: w741 -> [w757]
          tunnel: w740 -> [w754] mode=indexing
          tunnel: w739 -> [w751]
          tunnel: w738 -> [w749]
          shift-right: [w748] -> w735
          shift-left: w737 -> [w747]
          # "TT (Main).vit"
          n265 = vi-ref "TT (Main).vi"() -> (w746:refnum<vi>)
          n266 = Unbundle By Name(w754) -> ("Process Name"=w753:string, "Drop Coords"=w750:T10)
          n267 = To Variant(anything=w754) -> (Variant=w755:variant)
          n268 = property class="VI"(reference=w746) -> ("Path"=w745:path)  [unwired: 1 in, 2 out]
          n269 = Bundle By Name(cluster=T86 {"Module VI Filepath"=path "", "Process Name"="", "Main UI Message Queue"=refnum, "Drop Coords"={"Horizontal"=0, "Vertical"=0}, "Module Parameters"=variant, "Name of Parent Window"=""} ("Drop Parameters"), "Module VI Filepath"=w745, "Module Parameters"=w755, "Process Name"=w753, "Main UI Message Queue"=w749, "Drop Coords"=w750, "Name of Parent Window"=w751) -> (w752:T86)
          n270 = call "Next Instance Number.vi"("Module Type"=Module_Type_Enum."TT", "Operation"=Module_Instance_Number_Operation_Enum."Next Instance Number") -> ()  [unwired: 8 in, 2 out]
          n271 = call "Drop Start VI.vi"("error in (no error)"=w747, "Drop Parameters"=w752, "State in"=w757) -> ("error out"=w748:errorcluster, "State out"=w758:T1)  [unwired: 7 in]
        }
        n272 = call "Write to Log File.vi"("error in"=w735, "text"="Main: Update Config (TT)") -> ()  [unwired: 9 in, 1 out]
      }
      frame "Update Config (PT)" {
        # "Create PT Modules and \"drop\" them on the Picture Control and assign configs"
        n273 = Unbundle By Name(w765) -> ("Main Config.PT Module Configs"=w764:T41[])
        n274 = property class="VI"() -> ("Front Panel.Title"=w763:string)  [unwired: 2 in, 2 out]
        n275 = for {
          shift-right: [w782] -> w766
          shift-left: w765 -> [w781]
          tunnel: w764 -> [w778] mode=indexing
          tunnel: w763 -> [w775]
          tunnel: w762 -> [w773]
          shift-right: [w772] -> w759
          shift-left: w761 -> [w771]
          n276 = vi-ref "PT (Main).vi"() -> (w770:refnum<vi>)
          n277 = To Variant(anything=w778) -> (Variant=w779:variant)
          n278 = Unbundle By Name(w778) -> ("Process Name"=w777:string, "Drop Coords"=w774:T10)
          n279 = property class="VI"(reference=w770) -> ("Path"=w769:path)  [unwired: 1 in, 2 out]
          n280 = Bundle By Name(cluster=T86 {"Module VI Filepath"=path "", "Process Name"="", "Main UI Message Queue"=refnum, "Drop Coords"={"Horizontal"=0, "Vertical"=0}, "Module Parameters"=variant, "Name of Parent Window"=""} ("Drop Parameters"), "Module VI Filepath"=w769, "Module Parameters"=w779, "Process Name"=w777, "Main UI Message Queue"=w773, "Drop Coords"=w774, "Name of Parent Window"=w775) -> (w776:T86)
          n281 = call "Drop Start VI.vi"("error in (no error)"=w771, "Drop Parameters"=w776, "State in"=w781) -> ("error out"=w772:errorcluster, "State out"=w782:T1)  [unwired: 7 in]
          n282 = call "Next Instance Number.vi"("Module Type"=Module_Type_Enum."PT", "Operation"=Module_Instance_Number_Operation_Enum."Next Instance Number") -> ()  [unwired: 8 in, 2 out]
        }
        n283 = call "Write to Log File.vi"("error in"=w759, "text"="Main: Update Config (PT)") -> ()  [unwired: 9 in, 1 out]
      }
      frame "Update Config (U3)" {
        # "Create U3 Modules and \"drop\" them on the Picture Control and assign configs"
        n284 = Unbundle By Name(w789) -> ("Main Config.U3 Module Configs"=w788:T46[])
        n285 = property class="VI"() -> ("Front Panel.Title"=w787:string)  [unwired: 2 in, 2 out]
        n286 = for {
          shift-right: [w806] -> w790
          shift-left: w789 -> [w805]
          tunnel: w788 -> [w802] mode=indexing
          tunnel: w787 -> [w799]
          tunnel: w786 -> [w797]
          shift-right: [w796] -> w783
          shift-left: w785 -> [w795]
          n287 = vi-ref "U3 Module.lvlib:U3 (Main).vit"() -> (w794:refnum<vi>)
          n288 = Unbundle By Name(w802) -> ("Process Name"=w801:string, "Drop Coords"=w798:T10)
          n289 = To Variant(anything=w802) -> (Variant=w803:variant)
          n290 = property class="VI"(reference=w794) -> ("Path"=w793:path)  [unwired: 1 in, 2 out]
          n291 = Bundle By Name(cluster=T86 {"Module VI Filepath"=path "", "Process Name"="", "Main UI Message Queue"=refnum, "Drop Coords"={"Horizontal"=0, "Vertical"=0}, "Module Parameters"=variant, "Name of Parent Window"=""} ("Drop Parameters"), "Module VI Filepath"=w793, "Module Parameters"=w803, "Process Name"=w801, "Main UI Message Queue"=w797, "Drop Coords"=w798, "Name of Parent Window"=w799) -> (w800:T86)
          n292 = call "Drop Start VI.vi"("error in (no error)"=w795, "Drop Parameters"=w800, "State in"=w805) -> ("error out"=w796:errorcluster, "State out"=w806:T1)  [unwired: 7 in]
          n293 = call "Next Instance Number.vi"("Module Type"=Module_Type_Enum."U3", "Operation"=Module_Instance_Number_Operation_Enum."Next Instance Number") -> ()  [unwired: 8 in, 2 out]
        }
        n294 = call "Write to Log File.vi"("error in"=w783, "text"="Main: Update Config (U3)") -> ()  [unwired: 9 in, 1 out]
      }
      frame "Update Config (Feed)" {
        # "Create Feed Modules and \"drop\" them on the Picture Control and assign configs"
        n295 = Unbundle By Name(w813) -> ("Main Config.Feed Module Configs"=w812:T18[])
        n296 = property class="VI"() -> ("Front Panel.Title"=w811:string)  [unwired: 2 in, 2 out]
        n297 = for {
          shift-right: [w830] -> w814
          shift-left: w813 -> [w829]
          tunnel: w812 -> [w826] mode=indexing
          tunnel: w811 -> [w823]
          tunnel: w810 -> [w821]
          shift-right: [w820] -> w807
          shift-left: w809 -> [w819]
          # "Feed Module (Main.vit"
          n298 = vi-ref "Feed Module (Main).vi"() -> (w818:refnum<vi>)
          n299 = To Variant(anything=w826) -> (Variant=w827:variant)
          n300 = Unbundle By Name(w826) -> ("Process Name"=w825:string, "Drop Coords"=w822:T10)
          n301 = property class="VI"(reference=w818) -> ("Path"=w817:path)  [unwired: 1 in, 2 out]
          n302 = Bundle By Name(cluster=T86 {"Module VI Filepath"=path "", "Process Name"="", "Main UI Message Queue"=refnum, "Drop Coords"={"Horizontal"=0, "Vertical"=0}, "Module Parameters"=variant, "Name of Parent Window"=""} ("Drop Parameters"), "Module VI Filepath"=w817, "Module Parameters"=w827, "Process Name"=w825, "Main UI Message Queue"=w821, "Drop Coords"=w822, "Name of Parent Window"=w823) -> (w824:T86)
          n303 = call "Drop Start VI.vi"("error in (no error)"=w819, "Drop Parameters"=w824, "State in"=w829) -> ("error out"=w820:errorcluster, "State out"=w830:T1)  [unwired: 7 in]
          n304 = call "Next Instance Number.vi"("Module Type"=Module_Type_Enum."Feed", "Operation"=Module_Instance_Number_Operation_Enum."Next Instance Number") -> ()  [unwired: 8 in, 2 out]
        }
        n305 = call "Write to Log File.vi"("error in"=w807, "text"="Main: Update Config (Feed)") -> ()  [unwired: 9 in, 1 out]
      }
      frame "Update Config (OPC)" {
        # "Create Feed Modules and \"drop\" them on the Picture Control and assign configs"
        n306 = Unbundle By Name(w837) -> ("Main Config.OPC Module Configs"=w836:T8[])
        n307 = property class="VI"() -> ("Front Panel.Title"=w835:string)  [unwired: 2 in, 2 out]
        n308 = for {
          shift-right: [w854] -> w838
          shift-left: w837 -> [w853]
          tunnel: w836 -> [w850] mode=indexing
          tunnel: w835 -> [w847]
          tunnel: w834 -> [w845]
          shift-right: [w844] -> w831
          shift-left: w833 -> [w843]
          # "OPC Module (Main).vit"
          n309 = vi-ref "OPC Main.vi"() -> (w842:refnum<vi>)
          n310 = To Variant(anything=w850) -> (Variant=w851:variant)
          n311 = Unbundle By Name(w850) -> ("Process Name"=w849:string, "Drop Coords"=w846:T10)
          n312 = property class="VI"(reference=w842) -> ("Path"=w841:path)  [unwired: 1 in, 2 out]
          n313 = Bundle By Name(cluster=T86 {"Module VI Filepath"=path "", "Process Name"="", "Main UI Message Queue"=refnum, "Drop Coords"={"Horizontal"=0, "Vertical"=0}, "Module Parameters"=variant, "Name of Parent Window"=""} ("Drop Parameters"), "Module VI Filepath"=w841, "Module Parameters"=w851, "Process Name"=w849, "Main UI Message Queue"=w845, "Drop Coords"=w846, "Name of Parent Window"=w847) -> (w848:T86)
          n314 = call "Drop Start VI.vi"("error in (no error)"=w843, "Drop Parameters"=w848, "State in"=w853) -> ("error out"=w844:errorcluster, "State out"=w854:T1)  [unwired: 7 in]
          n315 = call "Next Instance Number.vi"("Module Type"=Module_Type_Enum."OPC", "Operation"=Module_Instance_Number_Operation_Enum."Next Instance Number") -> ()  [unwired: 8 in, 2 out]
        }
        n316 = call "Write to Log File.vi"("error in"=w831, "text"="Main: Update Config (Feed)") -> ()  [unwired: 9 in, 1 out]
      }
      frame "Update Config (Pump)" {
        # "Create Pump Modules and \"drop\" them on the Picture Control and assign configs"
        n317 = Unbundle By Name(w861) -> ("Main Config.Pump Module Configs"=w860:T44[])
        n318 = property class="VI"() -> ("Front Panel.Title"=w859:string)  [unwired: 2 in, 2 out]
        n319 = for {
          shift-right: [w878] -> w862
          shift-left: w861 -> [w877]
          tunnel: w860 -> [w874] mode=indexing
          tunnel: w859 -> [w871]
          tunnel: w858 -> [w869]
          shift-right: [w868] -> w855
          shift-left: w857 -> [w867]
          # "Pump Module (Main).vit"
          n320 = vi-ref "Pump Module (Main).vi"() -> (w866:refnum<vi>)
          n321 = To Variant(anything=w874) -> (Variant=w875:variant)
          n322 = Unbundle By Name(w874) -> ("Process Name"=w873:string, "Drop Coords"=w870:T10)
          n323 = property class="VI"(reference=w866) -> ("Path"=w865:path)  [unwired: 1 in, 2 out]
          n324 = Bundle By Name(cluster=T86 {"Module VI Filepath"=path "", "Process Name"="", "Main UI Message Queue"=refnum, "Drop Coords"={"Horizontal"=0, "Vertical"=0}, "Module Parameters"=variant, "Name of Parent Window"=""} ("Drop Parameters"), "Module VI Filepath"=w865, "Module Parameters"=w875, "Process Name"=w873, "Main UI Message Queue"=w869, "Drop Coords"=w870, "Name of Parent Window"=w871) -> (w872:T86)
          n325 = call "Drop Start VI.vi"("error in (no error)"=w867, "Drop Parameters"=w872, "State in"=w877) -> ("error out"=w868:errorcluster, "State out"=w878:T1)  [unwired: 7 in]
          n326 = call "Next Instance Number.vi"("Module Type"=Module_Type_Enum."Pump", "Operation"=Module_Instance_Number_Operation_Enum."Next Instance Number") -> ()  [unwired: 8 in, 2 out]
        }
        n327 = call "Write to Log File.vi"("error in"=w855, "text"="Main: Update Config (Pump)") -> ()  [unwired: 9 in, 1 out]
      }
      frame "Update Config (DO)" {
        # "Create DO Modules and \"drop\" them on the Picture Control and assign configs"
        n328 = Unbundle By Name(w885) -> ("Main Config.DO Module Configs"=w884:T59[])
        n329 = property class="VI"() -> ("Front Panel.Title"=w883:string)  [unwired: 2 in, 2 out]
        n330 = for {
          shift-right: [w902] -> w886
          shift-left: w885 -> [w901]
          tunnel: w884 -> [w898] mode=indexing
          tunnel: w883 -> [w895]
          tunnel: w882 -> [w893]
          shift-right: [w892] -> w879
          shift-left: w881 -> [w891]
          # "DO Module (Main).vit"
          n331 = vi-ref "D-O Module.lvlib:D-O Module (Main).vi"() -> (w890:refnum<vi>)
          n332 = To Variant(anything=w898) -> (Variant=w899:variant)
          n333 = Unbundle By Name(w898) -> ("Process Name"=w897:string, "Drop Coords"=w894:T10)
          n334 = property class="VI"(reference=w890) -> ("Path"=w889:path)  [unwired: 1 in, 2 out]
          n335 = Bundle By Name(cluster=T86 {"Module VI Filepath"=path "", "Process Name"="", "Main UI Message Queue"=refnum, "Drop Coords"={"Horizontal"=0, "Vertical"=0}, "Module Parameters"=variant, "Name of Parent Window"=""} ("Drop Parameters"), "Module VI Filepath"=w889, "Module Parameters"=w899, "Process Name"=w897, "Main UI Message Queue"=w893, "Drop Coords"=w894, "Name of Parent Window"=w895) -> (w896:T86)
          n336 = call "Drop Start VI.vi"("error in (no error)"=w891, "Drop Parameters"=w896, "State in"=w901) -> ("error out"=w892:errorcluster, "State out"=w902:T1)  [unwired: 7 in]
          n337 = call "Next Instance Number.vi"("Module Type"=Module_Type_Enum."Pump", "Operation"=Module_Instance_Number_Operation_Enum."Next Instance Number") -> ()  [unwired: 8 in, 2 out]
        }
        n338 = call "Write to Log File.vi"("error in"=w879, "text"="Main: Update Config (DO)") -> ()  [unwired: 9 in, 1 out]
      }
      frame "Update Config (PR)" {
        # "Create Pressure Regulator Modules and \"drop\" them on the Picture Control and assign configs"
        n339 = Unbundle By Name(w909) -> ("Main Config.PR Module Configs"=w908:T64[])
        n340 = property class="VI"() -> ("Front Panel.Title"=w907:string)  [unwired: 2 in, 2 out]
        n341 = for {
          shift-right: [w926] -> w910
          shift-left: w909 -> [w925]
          tunnel: w908 -> [w922] mode=indexing
          tunnel: w907 -> [w919]
          tunnel: w906 -> [w917]
          shift-right: [w916] -> w903
          shift-left: w905 -> [w915]
          # "PR Module (Main).vit"
          n342 = vi-ref "4-20mA Module (Main).vi"() -> (w914:refnum<vi>)
          n343 = To Variant(anything=w922) -> (Variant=w923:variant)
          n344 = Unbundle By Name(w922) -> ("Process Name"=w921:string, "Drop Coords"=w918:T10)
          n345 = property class="VI"(reference=w914) -> ("Path"=w913:path)  [unwired: 1 in, 2 out]
          n346 = Bundle By Name(cluster=T86 {"Module VI Filepath"=path "", "Process Name"="", "Main UI Message Queue"=refnum, "Drop Coords"={"Horizontal"=0, "Vertical"=0}, "Module Parameters"=variant, "Name of Parent Window"=""} ("Drop Parameters"), "Module VI Filepath"=w913, "Module Parameters"=w923, "Process Name"=w921, "Main UI Message Queue"=w917, "Drop Coords"=w918, "Name of Parent Window"=w919) -> (w920:T86)
          n347 = call "Drop Start VI.vi"("error in (no error)"=w915, "Drop Parameters"=w920, "State in"=w925) -> ("error out"=w916:errorcluster, "State out"=w926:T1)  [unwired: 7 in]
          n348 = call "Next Instance Number.vi"("Module Type"=Module_Type_Enum."Pump", "Operation"=Module_Instance_Number_Operation_Enum."Next Instance Number") -> ()  [unwired: 8 in, 2 out]
        }
        n349 = call "Write to Log File.vi"("error in"=w903, "text"="Main: Update Config (PR)") -> ()  [unwired: 9 in, 1 out]
      }
      frame "Update Config (TCU)" {
        # "Create TCU Modules and \"drop\" them on the Picture Control and assign configs"
        n350 = Unbundle By Name(w933) -> ("Main Config.TCU Module Configs"=w932:T50[])
        n351 = property class="VI"() -> ("Front Panel.Title"=w931:string)  [unwired: 2 in, 2 out]
        n352 = for {
          shift-right: [w950] -> w934
          shift-left: w933 -> [w949]
          tunnel: w932 -> [w946] mode=indexing
          tunnel: w931 -> [w943]
          tunnel: w930 -> [w941]
          shift-right: [w940] -> w927
          shift-left: w929 -> [w939]
          # "TCU Module (Main).vit"
          n353 = vi-ref "TCU Module.lvlib:TCU Module (Main).vi"() -> (w938:refnum<vi>)
          n354 = To Variant(anything=w946) -> (Variant=w947:variant)
          n355 = Unbundle By Name(w946) -> ("Process Name"=w945:string, "Drop Coords"=w942:T10)
          n356 = property class="VI"(reference=w938) -> ("Path"=w937:path)  [unwired: 1 in, 2 out]
          n357 = Bundle By Name(cluster=T86 {"Module VI Filepath"=path "", "Process Name"="", "Main UI Message Queue"=refnum, "Drop Coords"={"Horizontal"=0, "Vertical"=0}, "Module Parameters"=variant, "Name of Parent Window"=""} ("Drop Parameters"), "Module VI Filepath"=w937, "Module Parameters"=w947, "Process Name"=w945, "Main UI Message Queue"=w941, "Drop Coords"=w942, "Name of Parent Window"=w943) -> (w944:T86)
          n358 = call "Drop Start VI.vi"("error in (no error)"=w939, "Drop Parameters"=w944, "State in"=w949) -> ("error out"=w940:errorcluster, "State out"=w950:T1)  [unwired: 7 in]
          n359 = call "Next Instance Number.vi"("Module Type"=Module_Type_Enum."TCU", "Operation"=Module_Instance_Number_Operation_Enum."Next Instance Number") -> ()  [unwired: 8 in, 2 out]
        }
        n360 = call "Write to Log File.vi"("error in"=w927, "text"="Main: Update Config (TCU)") -> ()  [unwired: 9 in, 1 out]
      }
      frame "Update Config (Scale)" {
        # "Create Scale Modules and \"drop\" them on the Picture Control and assign configs"
        n361 = Unbundle By Name(w957) -> ("Main Config.Scale Module Configs"=w956:T42[])
        n362 = property class="VI"() -> ("Front Panel.Title"=w955:string)  [unwired: 2 in, 2 out]
        n363 = for {
          shift-right: [w974] -> w958
          shift-left: w957 -> [w973]
          tunnel: w956 -> [w970] mode=indexing
          tunnel: w955 -> [w967]
          tunnel: w954 -> [w965]
          shift-right: [w964] -> w951
          shift-left: w953 -> [w963]
          # "Scale Module (Main).vit"
          n364 = vi-ref "Scale Module (Main).vi"() -> (w962:refnum<vi>)
          n365 = To Variant(anything=w970) -> (Variant=w971:variant)
          n366 = Unbundle By Name(w970) -> ("Process Name"=w969:string, "Drop Coords"=w966:T10)
          n367 = property class="VI"(reference=w962) -> ("Path"=w961:path)  [unwired: 1 in, 2 out]
          n368 = Bundle By Name(cluster=T86 {"Module VI Filepath"=path "", "Process Name"="", "Main UI Message Queue"=refnum, "Drop Coords"={"Horizontal"=0, "Vertical"=0}, "Module Parameters"=variant, "Name of Parent Window"=""} ("Drop Parameters"), "Module VI Filepath"=w961, "Module Parameters"=w971, "Process Name"=w969, "Main UI Message Queue"=w965, "Drop Coords"=w966, "Name of Parent Window"=w967) -> (w968:T86)
          n369 = call "Drop Start VI.vi"("error in (no error)"=w963, "Drop Parameters"=w968, "State in"=w973) -> ("error out"=w964:errorcluster, "State out"=w974:T1)  [unwired: 7 in]
          n370 = call "Next Instance Number.vi"("Module Type"=Module_Type_Enum."Scale", "Operation"=Module_Instance_Number_Operation_Enum."Next Instance Number") -> ()  [unwired: 8 in, 2 out]
        }
        n371 = call "Write to Log File.vi"("error in"=w951, "text"="Main: Update Config (Scale)") -> ()  [unwired: 9 in, 1 out]
      }
      frame "Update Config (Flow)" {
        # "Create Flow Modules and \"drop\" them on the Picture Control and assign configs"
        n372 = Unbundle By Name(w981) -> ("Main Config.Flow Module Configs"=w980:T48[])
        n373 = property class="VI"() -> ("Front Panel.Title"=w979:string)  [unwired: 2 in, 2 out]
        n374 = for {
          shift-right: [w998] -> w982
          shift-left: w981 -> [w997]
          tunnel: w980 -> [w994] mode=indexing
          tunnel: w979 -> [w991]
          tunnel: w978 -> [w989]
          shift-right: [w988] -> w975
          shift-left: w977 -> [w987]
          # "Flow Module (Main).vit"
          n375 = vi-ref "Flow Module.lvlib:Flow Module (Main).vi"() -> (w986:refnum<vi>)
          n376 = To Variant(anything=w994) -> (Variant=w995:variant)
          n377 = Unbundle By Name(w994) -> ("Process Name"=w993:string, "Drop Coords"=w990:T10)
          n378 = property class="VI"(reference=w986) -> ("Path"=w985:path)  [unwired: 1 in, 2 out]
          n379 = Bundle By Name(cluster=T86 {"Module VI Filepath"=path "", "Process Name"="", "Main UI Message Queue"=refnum, "Drop Coords"={"Horizontal"=0, "Vertical"=0}, "Module Parameters"=variant, "Name of Parent Window"=""} ("Drop Parameters"), "Module VI Filepath"=w985, "Module Parameters"=w995, "Process Name"=w993, "Main UI Message Queue"=w989, "Drop Coords"=w990, "Name of Parent Window"=w991) -> (w992:T86)
          n380 = call "Drop Start VI.vi"("error in (no error)"=w987, "Drop Parameters"=w992, "State in"=w997) -> ("error out"=w988:errorcluster, "State out"=w998:T1)  [unwired: 7 in]
          n381 = call "Next Instance Number.vi"("Module Type"=Module_Type_Enum."Flow", "Operation"=Module_Instance_Number_Operation_Enum."Next Instance Number") -> ()  [unwired: 8 in, 2 out]
        }
        n382 = call "Write to Log File.vi"("error in"=w975, "text"="Main: Update Config (Flow)") -> ()  [unwired: 9 in, 1 out]
      }
      frame "Update Config (SC)" {
        # "Create Sonicator Modules and \"drop\" them on the Picture Control and assign configs"
        n383 = Unbundle By Name(w1005) -> ("Main Config.SC Module Configs"=w1004:T68[])
        n384 = property class="VI"() -> ("Front Panel.Title"=w1003:string)  [unwired: 2 in, 2 out]
        n385 = for {
          shift-right: [w1022] -> w1006
          shift-left: w1005 -> [w1021]
          tunnel: w1004 -> [w1018] mode=indexing
          tunnel: w1003 -> [w1015]
          tunnel: w1002 -> [w1013]
          shift-right: [w1012] -> w999
          shift-left: w1001 -> [w1011]
          # "Sonicator Module (Main).vit"
          n386 = vi-ref "Sonicator Module.lvlib:Sonicator Module (Main).vi"() -> (w1010:refnum<vi>)
          n387 = To Variant(anything=w1018) -> (Variant=w1019:variant)
          n388 = Unbundle By Name(w1018) -> ("Process Name"=w1017:string, "Drop Coords"=w1014:T10)
          n389 = property class="VI"(reference=w1010) -> ("Path"=w1009:path)  [unwired: 1 in, 2 out]
          n390 = Bundle By Name(cluster=T86 {"Module VI Filepath"=path "", "Process Name"="", "Main UI Message Queue"=refnum, "Drop Coords"={"Horizontal"=0, "Vertical"=0}, "Module Parameters"=variant, "Name of Parent Window"=""} ("Drop Parameters"), "Module VI Filepath"=w1009, "Module Parameters"=w1019, "Process Name"=w1017, "Main UI Message Queue"=w1013, "Drop Coords"=w1014, "Name of Parent Window"=w1015) -> (w1016:T86)
          n391 = call "Drop Start VI.vi"("error in (no error)"=w1011, "Drop Parameters"=w1016, "State in"=w1021) -> ("error out"=w1012:errorcluster, "State out"=w1022:T1)  [unwired: 7 in]
          n392 = call "Next Instance Number.vi"("Module Type"=Module_Type_Enum."Flow", "Operation"=Module_Instance_Number_Operation_Enum."Next Instance Number") -> ()  [unwired: 8 in, 2 out]
        }
        n393 = call "Write to Log File.vi"("error in"=w999, "text"="Main: Update Config (SC)") -> ()  [unwired: 9 in, 1 out]
      }
      frame "Update Config (AM)" {
        # "Create Agitator Modules and \"drop\" them on the Picture Control and assign configs"
        n394 = Unbundle By Name(w1029) -> ("Main Config.AM Module Configs"=w1028:T71[])
        n395 = property class="VI"() -> ("Front Panel.Title"=w1027:string)  [unwired: 2 in, 2 out]
        n396 = for {
          shift-right: [w1046] -> w1030
          shift-left: w1029 -> [w1045]
          tunnel: w1028 -> [w1042] mode=indexing
          tunnel: w1027 -> [w1039]
          tunnel: w1026 -> [w1037]
          shift-right: [w1036] -> w1023
          shift-left: w1025 -> [w1035]
          # "Agitator Module (Main).vit"
          n397 = vi-ref "Agitator Module.lvlib:Agitator Module (Main).vi"() -> (w1034:refnum<vi>)
          n398 = To Variant(anything=w1042) -> (Variant=w1043:variant)
          n399 = Unbundle By Name(w1042) -> ("Process Name"=w1041:string, "Drop Coords"=w1038:T10)
          n400 = property class="VI"(reference=w1034) -> ("Path"=w1033:path)  [unwired: 1 in, 2 out]
          n401 = Bundle By Name(cluster=T86 {"Module VI Filepath"=path "", "Process Name"="", "Main UI Message Queue"=refnum, "Drop Coords"={"Horizontal"=0, "Vertical"=0}, "Module Parameters"=variant, "Name of Parent Window"=""} ("Drop Parameters"), "Module VI Filepath"=w1033, "Module Parameters"=w1043, "Process Name"=w1041, "Main UI Message Queue"=w1037, "Drop Coords"=w1038, "Name of Parent Window"=w1039) -> (w1040:T86)
          n402 = call "Drop Start VI.vi"("error in (no error)"=w1035, "Drop Parameters"=w1040, "State in"=w1045) -> ("error out"=w1036:errorcluster, "State out"=w1046:T1)  [unwired: 7 in]
          n403 = call "Next Instance Number.vi"("Module Type"=Module_Type_Enum."Flow", "Operation"=Module_Instance_Number_Operation_Enum."Next Instance Number") -> ()  [unwired: 8 in, 2 out]
        }
        n404 = call "Write to Log File.vi"("error in"=w1023, "text"="Main: Update Config (AM") -> ()  [unwired: 9 in, 1 out]
      }
      frame "Update Config (Decoration)" {
        # "Display all decorations (e.g. arrows, lines) that are in the campaign. Get the image path for the decoration and raw them on the canvas."
        n405 = Unbundle By Name(w1050) -> ("Main Config.Decoration Module Configs"=w1051:T47[])
        n406 = property class="VI"() -> ("Front Panel.Title"=w1052:string)  [unwired: 2 in, 2 out]
        n407 = Current VI's Path() -> (path=w1053:path)
        n408 = call "Image Folder.vi"("Main VI path"=w1053) -> ("Image Folder path"=w1054:path)  [unwired: 10 in]
        n409 = for "For every decoration (e.g. arrows, lines)" {
          tunnel: w1051 -> [w1065] mode=indexing
          tunnel: w1052 -> [_]
          shift-right: [w1055] -> w1047
          shift-left: w1049 -> [w1055]
          tunnel: w1054 -> [w1058]
          # "Use relative path of\nthe image in case\nthe image folder has\nchanged."
          n410 = Unbundle By Name(w1065) -> ("Decoration Filepath"=w1059:path, "Drop Coords"=w1060:T10)
          n411 = Strip Path(path=w1059) -> (name=w1057:string)  [unwired: 1 out]
          n412 = Build Path(base path=w1058, name or relative path=w1057) -> (appended path=w1056:path)
          n413 = Unbundle By Name(w1060) -> ("Horizontal"=w1062:i32, "Vertical"=w1061:i32)
          n414 = local read "Canvas"() -> (w1064:picture)
          n415 = call "Draw BMP at Location.vi"("top"=w1061, "left"=w1062, "selected path"=w1056, "picture in"=w1064) -> ("picture out"=w1063:picture)  [unwired: 5 in, 2 out]
          n416 = local write "Canvas"(w1063) -> ()
        }
        n417 = call "Write to Log File.vi"("error in"=w1047, "text"="Main: Update Config (Decoration)") -> ()  [unwired: 9 in, 1 out]
      }
      frame "Drag Start" {
        n418 = Variant To Data(error in=w1080, type=T76 {"Mouse Position"={"X"=0, "Y"=0}, "Mouse Modifiers"={"Button Down"=FALSE, "Shift Mod"=FALSE, "Menu Mod"=FALSE, "Option Mod"=FALSE}} ("Mouse"), Variant=w1079) -> (data=w1074:T76, error out=w1078:errorcluster)
        n419 = Unbundle By Name(w1074) -> ("Mouse Position"=w1073:cluster{"X":i32, "Y":i32})
        n420 = Unbundle By Name(w1071) -> ("[Thumbnails]"=w1077:T2[])
        n421 = call "Which Thumbnail.vi"("error in (no error)"=w1078, "Coords"=w1073, "[Thumbnails]"=w1077) -> ("error out"=w1068:errorcluster, "Path"=→"Path":path, "index of element"=w1067:i32)  [unwired: 6 in]
        "index of element" <- w1067
        n422 = call "Palette Cursors.vi"("error in (no error)"=w1068, "Index"=w1067) -> ("error out"=w1069:errorcluster, "cursor ID"=w1070:refnum<k1>)  [unwired: 7 in, 1 out]
        n423 = Bundle By Name(cluster=w1071, "Drag Object Idx"=w1067) -> (w1072:T1)
        n424 = call-poly <vilib>:"Set Cursor.vi"("error in (no error)"=w1069, "cursor ID"=w1070) -> ("error out"=w1066:errorcluster)  [unwired: 8 in, 1 out]
      }
      frame "Drop" {
        (unwired) T76 {"Mouse Position"={"X"=0, "Y"=0}, "Mouse Modifiers"={"Button Down"=FALSE, "Shift Mod"=FALSE, "Menu Mod"=FALSE, "Option Mod"=FALSE}} ("Mouse")
        n425 = Variant To Data(error in=w1095, type=cluster{"Coords":T10, "Mouse":T76} {"Coords"={"Horizontal"=0, "Vertical"=0}, "Mouse"={"Mouse Position"={"X"=0, "Y"=0}, "Mouse Modifiers"={"Button Down"=FALSE, "Shift Mod"=FALSE, "Menu Mod"=FALSE, "Option Mod"=FALSE}}} ("output cluster"), Variant=w1097) -> (data=w1092:cluster{"Coords":T10, "Mouse":T76}, error out=w1096:errorcluster)
        n426 = Unbundle By Name(w1094) -> ("Drag Object Idx"=w1093:i32, "Drop Offset"=w1090:T6)
        n427 = Unbundle By Name(w1092) -> ("Mouse.Mouse Position"=w1091:cluster{"X":i32, "Y":i32})
        "Mouse Position" <- w1091
        n428 = case shown="Default" w1093 {
          selector: w1093 -> [_ w1107]
          tunnel: w1094 -> [w1100 w1105]
          tunnel: [w1100 w1110] -> w1082
          tunnel: [w1099 w1109] -> w1087
          tunnel: w1096 -> [w1099 w1108]
          tunnel: w1091 -> [_ w1104]
          tunnel: w1090 -> [_ _]
          tunnel: w1088 -> [_ w1103]
          tunnel: [T86 {"Module VI Filepath"=path "", "Process Name"="Error", "Main UI Message Queue"=refnum, "Drop Coords"={"Horizontal"=0, "Vertical"=0}, "Module Parameters"=variant, "Name of Parent Window"=""} ("Drop Parameters") w1101] -> w1081
          frame -1 {
          }
          frame Default {
            n429 = call "Thumbnail Path.vi"("Drag Object Idx"=w1107, "Cluster"=w1105) -> ("Module Type"=w1102:T84, "Thumbnail Path"=w1106:path)  [unwired: 8 in]
            n430 = case "Module Type?" shown="\"Feed\"..\"AM\"" w1102 {
              selector: w1102 -> [_ w1124]
              tunnel: [w1114 w1133] -> w1110
              tunnel: [w1118 w1132] -> w1109
              tunnel: w1108 -> [w1118 w1129]
              tunnel: w1104 -> [w1116 w1128]
              tunnel: w1106 -> [w1113 _]
              tunnel: w1105 -> [w1115 w1126]
              tunnel: w1103 -> [w1112 w1127]
              tunnel: [T86 {"Module VI Filepath"=path "", "Process Name"="Error", "Main UI Message Queue"=refnum, "Drop Coords"={"Horizontal"=0, "Vertical"=0}, "Module Parameters"=variant, "Name of Parent Window"=""} ("Drop Parameters") w1123] -> w1101
              frame "<unknown module>" {
                # "Non functional module (i.e. decoration like an arrow or line) has been dropped\nby the user. Save the filepath of the image being drawn and the coordinates into the\ncampaign configuration so it can be saved and recalled later."
                n431 = property class="VI"() -> ("Front Panel.Title"=w1117:string)  [unwired: 2 in, 2 out]
                n432 = call "Drop Decoration Parameters.vi"("Main UI Message Queue"=w1112, "Mouse Position"=w1116, "Parent Window Title"=w1117, "Path to Decoration image"=w1113, "State in"=w1115) -> ("State out"=w1114:T1)  [unwired: 4 in, 2 out]
                n433 = local read "Canvas"() -> (w1122:picture)
                n434 = Unbundle By Name(w1116) -> ("X"=w1120:i32, "Y"=w1119:i32)
                n435 = call "Draw BMP at Location.vi"("top"=w1119, "left"=w1120, "selected path"=w1113, "picture in"=w1122) -> ("picture out"=w1121:picture)  [unwired: 5 in, 2 out]
                n436 = local write "Canvas"(w1121) -> ()
              }
              frame "Feed".."AM" {
                n437 = property class="VI"() -> ("Front Panel.Title"=w1125:string)  [unwired: 2 in, 2 out]
                n438 = call "Drop Parameters.vi"("Main UI Message Queue"=w1127, "Mouse Position"=w1128, "error in (no error)"=w1129, "Parent Window Title"=w1125, "Module Type"=w1124, "State in"=w1126) -> ("error out"=w1130:errorcluster, "Drop Parameters"=w1123:T86, "State out"=w1131:T1)  [unwired: 3 in]
                n439 = call "Drop Start VI.vi"("error in (no error)"=w1130, "Drop Parameters"=w1123, "State in"=w1131) -> ("error out"=w1132:errorcluster, "State out"=w1133:T1)  [unwired: 7 in]
              }
            }
          }
        }
        n440 = Unbundle By Name(w1081) -> ("Process Name"=w1084:string)
        n441 = Concatenate Strings("Main: " ("string"), w1084, " Dropped" ("text")) -> (w1086:string)
        n442 = call "Write to Log File.vi"("error in"=w1087, "text"=w1086) -> ()  [unwired: 9 in, 1 out]
      }
      frame "E-Stop" {
        # "Stop the VI?"
        # "Tell all the modules to do E-Stop"
        n443 = call "E-Stop.vi"("State in"=w1139) -> ("error out"=w1137:errorcluster, "State out"=w1138:T1)  [unwired: 9 in]
        n444 = Merge Errors(w1137, w1136) -> (w1134:errorcluster)
        n445 = call "Write to Log File.vi"("error in"=w1134, "text"="Main: E-STOP Activated") -> ()  [unwired: 9 in, 1 out]
      }
      frame "Error" {
        w1150 = T94 1 items=["no dialog", "OK message", "continue or stop message", "OK message + warnings", "continue/stop + warnings"] ("type of dialog (OK msg:1)")
        # "Error - Check the error message data and respond accordingly. This message is sent by the \"Error Handler\" VIs at the end of each loop in this application."
        n446 = Variant To Data(type=errorcluster {"status"=FALSE, "code"=0, "source"=""} ("error out"), Variant=w1155) -> (data=w1149:errorcluster, error out=w1148:errorcluster)  [unwired: 1 in]
        n447 = Merge Errors(w1149, w1148) -> (w1147:errorcluster)
        "data" <- w1147
        n448 = call <vilib>:"General Error Handler.vi"("type of dialog (OK msg:1)"=w1150, "error in (no error)"=w1147) -> ("message"=w1141:string, "error out"=w1143:errorcluster)  [unwired: 9 in, 3 out]
        n449 = disable-structure shown="Enabled" {
          disable-tunnel: w1153 -> [w1159 _]
          disable-tunnel: [w1156 _] -> w1152
          disable-tunnel: w1143 -> [_ _]
          frame Disabled {
            n450 = call-poly "Enqueue Message.vi"("Priority Message? (F)"=TRUE, "Message"="Exit", "Message Queue"=w1159) -> ("error out"=w1156:errorcluster)  [unwired: 7 in, 1 out]
          }
          frame Enabled {
            # "If infinite error loop, slow it down\nso user can exit"
            n451 = Wait (ms)(milliseconds to wait=u32 2000) -> ()  [unwired: 1 out]
          }
        }
        n452 = Merge Errors(w1152, w1148) -> (w1146:errorcluster)
        n453 = call <vilib>:"Clear Errors.vi"("error in (no error)"=w1146) -> ("error out"=w1145:errorcluster)  [unwired: 5 in, 1 out]
        n454 = Concatenate Strings("Main: Error in Main: " ("text"), w1141) -> (w1142:string)
        n455 = call "Write to Log File.vi"("error in"=w1145, "text"=w1142) -> ()  [unwired: 9 in, 1 out]
        "Message Data" <- w1155
      }
      frame "Exit" {
        # "Stop and close the dynamically launched modules\n(e.g. Feed Modules)"
        # "Don't stop the VI quite yet. Wait for the DAQ to\nstop so we can delete the tags/shared variables."
        # "Exit - Fire the User Event to stop the Event Handling Loop.  Also send Exit messages to the Acquisition and Logging loops."
        n456 = call "Fire User Event - Stop.vi"("User Event - Stop"=w1191) -> ("error out"=w1170:errorcluster)  [unwired: 10 in]
        n457 = Unbundle By Name(w1190) -> ("Waveform Loop"=w1186:refnum<queue>, "CSV Log"=w1189:refnum<queue>, "TDMS Log"=w1188:refnum<queue>, "Graphs"=w1173:refnum<queue>[], "DAQ"=w1176:refnum<queue>, "Sequence"=w1172:refnum<queue>)
        n458 = call "Palette Cursors.vi"() -> ("error out"=w1183:errorcluster, "Cursor IDs out"=w1184:refnum<k1>[])  [unwired: 9 in, 1 out]
        n459 = for {
          tunnel: w1184 -> [w1197] mode=indexing
          shift-right: [w1194] -> w1182
          shift-left: w1183 -> [w1196]
          n460 = call <vilib>:"Destroy Cursor.vi"("cursor ID"=w1197, "error in (no error)"=w1196) -> ("error out"=w1195:errorcluster)  [unwired: 8 in]
          n461 = call <vilib>:"Clear Errors.vi"("error in (no error)"=w1195) -> ("error out"=w1194:errorcluster)  [unwired: 5 in, 1 out]
        }
        n462 = Build Array (concatenate)(w1186, w1189, w1188, w1173, w1172) -> (w1187:refnum<queue>[])
        n463 = for "stop and close support VIs" {
          tunnel: w1187 -> [w1202] mode=indexing
          tunnel: [w1200] -> w1181 mode=indexing
          tunnel: w1170 -> [w1198]
          n464 = call-poly "Enqueue Message.vi"("error in (no error)"=w1198, "Message"="Stop", "Message Queue"=w1202) -> ("error out"=w1199:errorcluster, "dup Message Queue"=w1203:refnum<queue>)  [unwired: 7 in]
          n465 = call-poly "Enqueue Message.vi"("error in (no error)"=w1199, "Message"="Exit", "Message Queue"=w1203) -> ("error out"=w1200:errorcluster)  [unwired: 7 in, 1 out]
        }
        n466 = call-poly "Enqueue Message.vi"("Priority Message? (F)"=TRUE, "Message"="DAQ-Exit", "Message Queue"=w1176) -> ("error out"=w1178:errorcluster)  [unwired: 7 in, 1 out]
        n467 = Merge Errors(w1170, w1181, w1178) -> (w1180:errorcluster)
        n468 = call "Close VIs.vi"("error in (no error)"=w1180, "State in"=w1179) -> ("error out"=w1174:errorcluster, "State out"=w1161:T1)  [unwired: 8 in]
        n469 = flat-sequence {
          tunnel: w1174 -> [_]
          frame #0 {
            n470 = call "Tag FGV.vi"("Operation"=Tag_FGV_Operation_Enum."Delete All Tags") -> ()  [unwired: 7 in, 8 out]
          }
        }
        n471 = local read "CSV Log File"() -> (w1169:path)
        n472 = Strip Path(path=w1169) -> (stripped path=w1166:path, name=w1162:string)
        n473 = Strip Path(path=w1166) -> (stripped path=w1165:path)  [unwired: 1 out]
        n474 = Build Path(base path=w1165, name or relative path="SDC") -> (appended path=w1163:path)
        n475 = Merge Errors(w1175, w1174, w1182) -> (w1167:errorcluster)
        n476 = Build Path(base path=w1163, name or relative path=w1162) -> (appended path=w1168:path)
        n477 = Copy(10:w1168, 11:w1169) -> ()  [unwired: 3 in, 3 out]
        n478 = call "Write to Log File.vi"("error in"=w1167, "text"="Main: Exited") -> ()  [unwired: 9 in, 1 out]
      }
      frame "File-Settings" {
        # "Get the Process Name from the settings dialog"
        n479 = call "File-Settings-Dialog.vi"("error in (no error)"=w1210) -> ("error out"=w1206:errorcluster, "Process Name Out"=w1208:string)  [unwired: 9 in]
        n480 = Bundle By Name(cluster=w1209, "Process Name"=w1208) -> (w1205:T1)
        n481 = call "Write to Log File.vi"("error in"=w1206, "text"="Main: File-Settings") -> ()  [unwired: 9 in, 1 out]
      }
      frame "Initialize" {
        (unwired) "Thumbnail (Feed Module).bmp" ("name or relative path")
        # "Initialize - Get configuration settings, then message the UI to initialize, and broadcast the settings to the other message loops."
        n482 = call "Empty Picture"() -> ("empty picture"=w1243:picture)
        n483 = local write "Canvas"(w1243) -> ()
        n484 = call-poly "Enqueue Message.vi"("error in (no error)"=w1222, "Message"="New Document", "Message Queue"=w1223) -> ("error out"=w1215:errorcluster)  [unwired: 7 in, 1 out]
        n485 = property on="Start Log" class="Bool"("DisabledEnum"=T87."Enabled" ("Disabled")) -> ()  [unwired: 2 in, 2 out]
        n486 = property on="Pause Log Button" class="Bool (strict)"("DisabledEnum"=T87."Disabled and Grayed Out" ("Disabled")) -> ()  [unwired: 2 in, 2 out]
        n487 = property on="Palette" class="Pict"("DisabledEnum"=T87."Enabled" ("Disabled")) -> ()  [unwired: 2 in, 2 out]
        n488 = property class="VI"() -> ("Front Panel.PanelBounds"=w1235:T4, "Front Panel.WinBounds"=w1234:T4)  [unwired: 2 in, 2 out]
        "Front Panel Window:Panel Bounds" <- w1235
        n489 = property class="VI"() -> ("Panel"=w1228:refnum<vi>)  [unwired: 2 in, 2 out]
        n490 = Current VI's Path() -> (path=w1247:path)
        n491 = property on="Canvas" class="Pict"() -> ("Position"=w1233:T6)  [unwired: 2 in, 2 out]
        "Position" <- w1233
        n492 = property class="Pnl"(reference=w1228) -> ("Panes[]"=w1229:refnum<vi>[])  [unwired: 1 in, 2 out]
        n493 = call "Next Instance Number.vi"("Operation"=Module_Instance_Number_Operation_Enum."Init") -> ()  [unwired: 9 in, 2 out]
        n494 = disable-structure shown="Default" {
          disable-tunnel: w1247 -> [w1251 _]
          disable-tunnel: [w1250 w1252] -> w1216
          frame condition #0 (active) {
            n495 = Strip Path(path=w1251) -> (stripped path=w1250:path)  [unwired: 1 out]
          }
          frame condition #1 {
            n496 = Default Directory() -> (w1252:path)
          }
        }
        n497 = Index Array(array=w1229) -> (element=w1230:refnum<vi>)  [unwired: 1 in]
        n498 = property class="Pane"(reference=w1230) -> ("Origin"=w1231:T75)  [unwired: 1 in, 2 out]
        "Origin" <- w1231
        n499 = Build Path(base path=w1216, name or relative path="Images") -> (appended path=w1248:path)
        n500 = Subtract(x=w1234, y=w1235) -> (x-y=w1236:T4)
        "x-y" <- w1236
        n501 = Negate(x=w1231) -> (-x=w1232:T75)
        n502 = call "Load Palette Images.vi"("Palette Image Folder"=w1248) -> ("error out"=w1220:errorcluster, "Cursor IDs"=w1219:refnum<k1>[], "[Thumbnails]"=w1244:T2[], "new picture"=→"Palette":picture)  [unwired: 7 in]
        n503 = Unbundle By Name(w1236) -> ("Top"=w1237:i16)
        n504 = Add(x=w1232, y=w1233) -> (x+y=w1240:T6)
        n505 = Unbundle By Name(w1240) -> ("Top"=w1238:i32)
        n506 = Negate(x=w1237) -> (-x=w1241:i16)
        n507 = Add(x=w1241, y=w1238) -> (x+y=w1239:i32)
        n508 = Bundle By Name(cluster=w1240, "Top"=w1239) -> (w1227:T6)
        "Drop Offset" <- w1227
        n509 = call "Palette Cursors.vi"("error in (no error)"=w1220, "Initialize"=TRUE, "Cursor IDs in"=w1219) -> ()  [unwired: 6 in, 3 out]
        n510 = Bundle By Name(cluster=w1211, "[Thumbnails]"=w1244, "Active Object"=-1, "Drop Offset"=w1227, "Main Config.Cycle Period"=1.0) -> (w1245:T1)
        n511 = call "Write to Log File.vi"("error in"=w1215, "text"="Main: Initialized") -> ("error out"=w1214:errorcluster)  [unwired: 9 in]
      }
      frame "New Document" {
        # "Start DAQ. Don't wait for Start Log"
        # "DAQ task is cleared here"
        # "Reset all the tags."
        # "Called from initialize at the start of a run"
        n512 = call "Tag FGV.vi"("Operation"=Tag_FGV_Operation_Enum."Read All Tags", "error in (no error)"=w1259) -> ("error out"=w1260:errorcluster)  [unwired: 6 in, 7 out]
        n513 = call "Empty Picture"() -> ("empty picture"=w1262:picture)
        n514 = call "Tag FGV.vi"("Operation"=Tag_FGV_Operation_Enum."Init", "error in (no error)"=w1260) -> ("error out"=w1264:errorcluster)  [unwired: 6 in, 7 out]
        n515 = local write "Canvas"(w1262) -> ()
        n516 = call-poly "Enqueue Message.vi"("error in (no error)"=w1264, "Message"="DAQ-Initialize", "Message Queue"=w1263) -> ("error out"=w1256:errorcluster, "dup Message Queue"=w1257:refnum<queue>)  [unwired: 7 in]
        n517 = call-poly "Enqueue Message.vi"("error in (no error)"=w1256, "Message"="DAQ-Start", "Message Queue"=w1257) -> ("error out"=w1254:errorcluster)  [unwired: 7 in, 1 out]
        n518 = call "Write to Log File.vi"("error in"=w1254, "text"="Main: New Document") -> ("error out"=w1253:errorcluster)  [unwired: 9 in]
      }
      frame "Open Campaign" {
        # "Choose a saved campaign to load"
        # "Load a Campaign from a previous save"
        n519 = Unbundle By Name(w1273) -> ("Main Config"=w1284:T7, "Campaign Filepath"=w1277:path)
        n520 = call "Application Data Folder.vi"() -> ("Campaign Folder"=w1276:path)  [unwired: 7 in, 4 out]
        n521 = Empty String/Path?(string/path=w1277) -> (empty?=w1278:bool)
        n522 = Select(t=w1276, s=w1278, f=w1277) -> (s? t:f=w1275:path)
        n523 = call "File Dialog3"("start path"=w1275, "prompt"="Open campaign", "error in"=w1283, "pattern (all files)"="*.cfg") -> ("selected path"=w1281:path, "cancelled"=w1282:bool, "error out"=w1272:errorcluster)  [unwired: 8 in, 1 out]
        n524 = call <vilib>:"Clear Errors.vi"("error in (no error)"=w1272) -> ("error out"=w1271:errorcluster)  [unwired: 5 in, 1 out]
        n525 = case shown="False" w1282 {
          tunnel: w1284 -> [w1294 _]
          tunnel: w1271 -> [w1288 w1312]
          tunnel: [w1301 w1312] -> w1268
          tunnel: w1281 -> [w1305 _]
          tunnel: w1273 -> [w1296 w1311]
          tunnel: [w1303 w1311] -> w1274
          tunnel: w1270 -> [w1299 _]
          tunnel: w1269 -> [w1287 _]
          frame False {
            # "After the DAQ has executed its configuration, it will call the next case,\ni.e. Open Campaign-DAQ Commited\"\nwhich queues additional messages."
            # "close previously\nopened dynamic VIs"
            n526 = call "Empty Picture"() -> ("empty picture"=w1291:picture)
            n527 = call-poly "Enqueue Message.vi"("error in (no error)"=w1288, "Message"="DAQ-Stop", "Message Queue"=w1287) -> ("error out"=w1289:errorcluster)  [unwired: 7 in, 1 out]
            n528 = local write "Canvas"(w1291) -> ()
            n529 = call "Close VIs.vi"("error in (no error)"=w1289, "State in"=w1296) -> ("error out"=w1293:errorcluster, "State out"=w1297:T1)  [unwired: 8 in]
            n530 = call <vilib>:"Clear Errors.vi"("error in (no error)"=w1293) -> ("error out"=w1292:errorcluster)  [unwired: 5 in, 1 out]
            n531 = call "Clear Dynamic Module Configs.vi"("Main Config in"=w1294) -> ("Main Config out"=w1295:T7)  [unwired: 8 in, 1 out]
            n532 = call "Read-Write Config File.vi"("configuration file path"=w1305, "Main Config in"=w1295, "Mode"=Config_File_Operation_Enum."Read", "error in"=w1292) -> ("Config File Path"=w1304:path, "Main Config out"=w1286:T7, "error out"=w1302:errorcluster)  [unwired: 4 in]
            n533 = Unbundle By Name(w1286) -> ("Notebook"=w1285:string)
            n534 = Bundle By Name(cluster=w1297, "Campaign Filepath"=w1304, "Config Changed?"=FALSE, "Main Config"=w1286) -> (w1303:T1)
            n535 = for {
              tunnel: w1299 -> [w1308]
              shift-right: [w1309] -> w1301
              shift-left: w1302 -> [w1310]
              tunnel: string[] ["New Document", "Update Config (DAQ)"] -> [w1307] mode=indexing
              n536 = call-poly "Enqueue Message.vi"("error in (no error)"=w1310, "Message"=w1307, "Message Queue"=w1308) -> ("error out"=w1309:errorcluster)  [unwired: 7 in, 1 out]
            }
            n537 = property on="Notebook" class="Str"("Val(Sgnl)"=w1285) -> ()  [unwired: 2 in, 2 out]
          }
          frame True {
          }
        }
      }
      frame "Open Campaign-DAQ Commited" {
        # "Wait for DAQ Message Loop to commit its tags/shared variables before starting up the dynamic modules so that the dynamic modules that bind to tags/shared variables in the DAQ task will not error."
        n538 = for {
          tunnel: w1317 -> [w1319]
          shift-right: [w1320] -> w1313
          shift-left: _ -> [w1321]
          tunnel: string[] ["Update Config (TT)", "Update Config (Feed)", "Update Config (PT)", "Update Config (Pump)", "Update Config (Scale)", "Update Config (Flow)", "Update Config (U3)", "Update Config (Decoration)", "Update Config (TCU)", "Update Config (DO)", "Update Config (PR)", "Update Config (OPC)", "Update Config (SC)", "Update Config (AM)"] -> [w1318] mode=indexing
          n539 = call-poly "Enqueue Message.vi"("error in (no error)"=w1321, "Message"=w1318, "Message Queue"=w1319) -> ("error out"=w1320:errorcluster)  [unwired: 7 in, 1 out]
        }
        n540 = call "Write to Log File.vi"("error in"=w1313, "text"="Main: Campaign Opened") -> ()  [unwired: 9 in, 1 out]
      }
      frame "Read Config" {
        n541 = call "Read Main Config File.vi"("error in (no error)"=w1327) -> ("Main Config out"=w1324:T7, "error out"=w1322:errorcluster)  [unwired: 7 in, 1 out]
        n542 = Bundle By Name(cluster=w1325, "Main Config"=w1324) -> (w1326:T1)
        n543 = call "Write to Log File.vi"("error in"=w1322, "text"="Main: Read Config Completed") -> ()  [unwired: 9 in, 1 out]
      }
      frame "Save Campaign", "Save Campaign As" {
        n544 = local read "Notebook"() -> (w1329:string)
        n545 = Bundle By Name(cluster=w1330, "Main Config.Notebook"=w1329) -> (w1328:T1)
        n546 = Equal?(x=w1337, y="Save Campaign As") -> (x = y?=w1335:bool)
        n547 = call "Application Data Folder.vi"() -> ("Campaign Folder"=w1344:path)  [unwired: 7 in, 4 out]
        n548 = Unbundle By Name(w1328) -> ("Main Config"=w1345:T7, "Campaign Filepath"=w1339:path)
        n549 = Empty String/Path?(string/path=w1339) -> (empty?=w1334:bool)
        n550 = Or(x=w1334, y=w1335) -> (x .or. y?=w1333:bool)
        n551 = case shown="True" w1333 {
          tunnel: w1344 -> [_ w1356]
          tunnel: w1343 -> [w1348 w1353]
          tunnel: [w1348 w1349] -> w1342
          tunnel: [FALSE ("cancelled") w1352] -> w1341
          tunnel: [w1346 w1351] -> w1340
          tunnel: w1339 -> [w1346 _]
          frame False {
          }
          frame True {
            # "Choose a file name to save"
            n552 = call "File Dialog2"("start path"=w1356, "prompt"="Save campaign as", "error in"=w1353, "pattern (all files)"="*.cfg") -> ("selected path"=w1351:path, "cancelled"=w1352:bool, "error out"=w1350:errorcluster)  [unwired: 8 in, 1 out]
            n553 = call <vilib>:"Clear Errors.vi"("error in (no error)"=w1350) -> ("error out"=w1349:errorcluster)  [unwired: 5 in, 1 out]
          }
        }
        n554 = case shown="False" w1341 {
          tunnel: w1345 -> [w1363 _]
          tunnel: w1342 -> [w1362 w1366]
          tunnel: [w1361 w1366] -> w1331
          tunnel: w1340 -> [w1360 _]
          tunnel: w1328 -> [w1359 w1365]
          tunnel: [w1357 w1365] -> w1338
          frame False {
            n555 = call "Read-Write Config File.vi"("configuration file path"=w1360, "Main Config in"=w1363, "Mode"=Config_File_Operation_Enum."Write", "error in"=w1362) -> ("Config File Path"=w1358:path, "error out"=w1361:errorcluster)  [unwired: 4 in, 1 out]
            n556 = Bundle By Name(cluster=w1359, "Campaign Filepath"=w1358) -> (w1357:T1)
          }
          frame True {
          }
        }
        n557 = call "Write to Log File.vi"("error in"=w1331, "text"="Main: Campaign Saved") -> ()  [unwired: 9 in, 1 out]
      }
      frame "Start Log" {
        # "Set up the alarms, create the data and graphing files, create the data tags, and start the logging"
        n558 = Unbundle By Name(w1382) -> ("Waveform Loop"=w1378:refnum<queue>, "CSV Log"=w1367:refnum<queue>)
        n559 = Unbundle By Name(w1370) -> ("Queues"=w1377:refnum<queue>[])
        n560 = Unbundle By Name(w1370) -> ("Process Name"=w1381:string)
        n561 = Unbundle By Name(w1370) -> ("Main Config.Cycle Period"=w1368:dbl)
        n562 = Empty String/Path?(string/path=w1381) -> (empty?=w1380:bool)
        n563 = case "Is there a process name" shown="True" w1380 {
          tunnel: [w1443 w1448] -> w1375
          tunnel: w1381 -> [w1443 _]
          tunnel: [TRUE w1444] -> w1369
          frame False {
          }
          frame True {
            n564 = Empty String/Path?(string/path="Notebook") -> (empty?=w1445:bool)
            n565 = Concatenate Strings("Notebook", "" ("string")) -> (w1448:string)
            n566 = Not(x=w1445) -> (.not. x?=w1444:bool)
          }
        }
        n567 = Max & Min(x=w1368, y=1.0) -> (max(x,y)=w1373:dbl)  [unwired: 1 out]
        n568 = case shown="True" w1369 {
          tunnel: w1379 -> [w1383 w1410]
          tunnel: w1378 -> [_ w1406]
          tunnel: w1377 -> [_ w1405]
          tunnel: w1376 -> [_ w1404]
          tunnel: w1367 -> [_ w1403]
          tunnel: w1367 -> [_ w1399]
          tunnel: w1375 -> [_ w1398]
          tunnel: w1373 -> [_ w1393]
          tunnel: [w1383 w1392] -> w1372
          tunnel: w1371 -> [_ w1391]
          tunnel: w1370 -> [_ w1390]
          frame False {
            n569 = One Button Dialog(message="Enter a Notebook #") -> ()  [unwired: 1 in, 1 out]
          }
          frame True {
            w1387 = "Add Note" ("item name")
            w1395 = "Set Data Rate" ("item tag")
            # "Add the menu item when the Log is Started"
            # "The Cycle Rate cannot be changed mid run"
            n570 = call-poly "Enqueue Message.vi"("Message Data"=w1398, "Message"="Notebook", "Message Queue"=w1399) -> ()  [unwired: 7 in, 2 out]
            n571 = call "Logfile Paths.vi"("File Name"=w1398) -> ("Alarm CSV Logfile path"=w1407:path, "TDMS Logfile path"=w1416:path, "CSV Logfile path"=w1414:path)  [unwired: 8 in]
            "CSV Log File" <- w1414
            n572 = call-poly "Enqueue Message.vi"("Message Data"=w1390, "Message"="Start", "Message Queue"=w1391) -> ()  [unwired: 7 in, 2 out]
            n573 = Bundle By Name(cluster=T90 {"dt (seconds)"=0.1, "CSV Logfile path"=path "", "TDMS Logfile path"=path ""} ("Start Params"), "dt (seconds)"=w1393, "CSV Logfile path"=w1414, "TDMS Logfile path"=w1416) -> (w1415:T90)
            n574 = call "Log Alarm FGV.vi"("error in (no error)"=w1410, "Path"=w1407, "Operation"=Alarm_Log_Operation_Enum."Create Log") -> ("error out"=w1408:errorcluster)  [unwired: 8 in]
            n575 = flat-sequence {
              tunnel: w1405 -> [w1421]
              tunnel: w1408 -> [w1420]
              tunnel: [w1422] -> w1419
              tunnel: w1419 -> [w1431]
              tunnel: [w1430] -> w1418
              tunnel: w1404 -> [w1432]
              tunnel: w1390 -> [w1429]
              tunnel: w1418 -> [w1435]
              tunnel: w1415 -> [w1441]
              tunnel: w1406 -> [w1439]
              tunnel: [w1433] -> w1401
              tunnel: w1390 -> [w1437]
              tunnel: w1403 -> [w1436]
              frame #0 {
                n576 = for {
                  tunnel: w1421 -> [w1427] mode=indexing
                  tunnel: w1420 -> [w1426]
                  tunnel: [w1425] -> w1423 mode=indexing
                  n577 = Wait (ms)(milliseconds to wait=u32 250) -> ()  [unwired: 1 out]
                  n578 = call-poly "Enqueue Message.vi"("error in (no error)"=w1426, "Message"="Start Log", "Message Queue"=w1427) -> ("error out"=w1425:errorcluster)  [unwired: 7 in, 1 out]
                }
                n579 = Merge Errors(w1420, w1423) -> (w1422:errorcluster)
              }
              frame #1 {
                n580 = call "Check Module Tag Creation.vi"("error in (no error)"=w1431, "Cluster"=w1429, "UI"=w1432) -> ("error out"=w1430:errorcluster)  [unwired: 8 in]
              }
              frame #2 {
                n581 = call-poly "Enqueue Message.vi"("error in (no error)"=w1435, "Message Data"=w1437, "Message"="Log Settings", "Message Queue"=w1436) -> ("error out"=w1434:errorcluster)  [unwired: 6 in, 1 out]
                n582 = call-poly "Enqueue Message.vi"("error in (no error)"=w1434, "Message Data"=w1441, "Message"="Start", "Message Queue"=w1439) -> ("error out"=w1433:errorcluster)  [unwired: 6 in, 1 out]
              }
            }
            n583 = property on="Pause Log Button" class="Bool (strict)"("Val(Sgnl)"=FALSE ("Pause Log Button")) -> ()  [unwired: 2 in, 2 out]
            n584 = property on="Palette" class="Pict"("DisabledEnum"=T87."Disabled and Grayed Out" ("Disabled")) -> ()  [unwired: 2 in, 2 out]
            n585 = property on="Pause Log Button" class="Bool (strict)"("DisabledEnum"=T87."Enabled" ("Disabled")) -> ()  [unwired: 2 in, 2 out]
            n586 = property on="Start Log" class="Bool"("DisabledEnum"=T87."Disabled and Grayed Out" ("Disabled")) -> ()  [unwired: 2 in, 2 out]
            n587 = Current VI's Menubar() -> (w1388:refnum<k9>)
            n588 = Set Menu Item Info(7:w1387, 9:TRUE ("enabled"), 10:w1387, 11:w1388) -> ()  [unwired: 3 in, 2 out]
            n589 = Current VI's Menubar() -> (w1396:refnum<k9>)
            n590 = call "Tag FGV.vi"("Operation"=Tag_FGV_Operation_Enum."Enable All Alarms", "error in (no error)"=w1401) -> ("error out"=w1392:errorcluster)  [unwired: 6 in, 7 out]
            n591 = Set Menu Item Info(7:w1395, 9:FALSE ("enabled"), 10:w1395, 11:w1396) -> ()  [unwired: 3 in, 2 out]
            n592 = call "Write to Log File.vi"("error in"=w1392, "text"="Main: Data Log Started") -> ()  [unwired: 9 in, 1 out]
          }
        }
      }
      frame "Stop Log" {
        # "Stop Waveform loop,\nwhich stops the\nCSV Log and\nTDMS Log."
        # "Stop the logging"
        n593 = Unbundle By Name(w1460) -> ("Waveform Loop"=w1459:refnum<queue>)
        n594 = property on="Palette" class="Pict"("DisabledEnum"=T87."Enabled" ("Disabled")) -> ()  [unwired: 2 in, 2 out]
        n595 = call-poly "Enqueue Message.vi"("error in (no error)"=w1457, "Message"="Stop", "Message Queue"=w1459) -> ("error out"=w1455:errorcluster)  [unwired: 7 in, 1 out]
        n596 = property on="Start Log" class="Bool"("DisabledEnum"=T87."Enabled" ("Disabled")) -> ()  [unwired: 2 in, 2 out]
        n597 = property on="Pause Log Button" class="Bool (strict)"("DisabledEnum"=T87."Disabled and Grayed Out" ("Disabled")) -> ()  [unwired: 2 in, 2 out]
        n598 = call "Log Alarm FGV.vi"("error in (no error)"=w1455, "Operation"=Alarm_Log_Operation_Enum."Close Log") -> ("error out"=w1449:errorcluster)  [unwired: 9 in]
        n599 = call "Write to Log File.vi"("error in"=w1449, "text"="Main: Data Log Stopped") -> ()  [unwired: 9 in, 1 out]
      }
      frame "Timeout" {
        # "Prevent CPU from overloading in the case that this is called too often."
        n600 = Wait (ms)(milliseconds to wait=u32 5) -> ()  [unwired: 1 out]
      }
      frame "Launch Sequence Dialog" {
        # "Control the execution of the Sequencer"
        n601 = call "Sequence Dialog.vi"("error in (no error)"=w1475, "Sequence UI"=w1464, "State Cluster In"=w1468) -> ("error out"=w1471:errorcluster, "Start"=w1469:bool, "cancelled"=w1474:bool, "State Cluster Out"=w1473:T1, "Pause"=w1467:bool)  [unwired: 3 in, 1 out]
        n602 = case "Is it Cancelled?" shown="False" w1474 {
          tunnel: w1473 -> [w1482 _]
          tunnel: [w1482 w1502] -> w1472
          tunnel: w1471 -> [w1486 w1503]
          tunnel: w1470 -> [w1484 _]
          tunnel: [w1476 w1503] -> w1465
          tunnel: w1469 -> [w1483 _]
          tunnel: w1468 -> [_ w1502]
          tunnel: w1467 -> [w1481 _]
          frame False {
            n603 = call-poly "Enqueue Message.vi"("error in (no error)"=w1486, "Message Data"=w1482, "Message"="Update Sequence", "Message Queue"=w1484) -> ("error out"=w1477:errorcluster, "dup Message Queue"=w1478:refnum<queue>)  [unwired: 6 in]
            n604 = case "Is it Paused?" shown="True" w1481 {
              tunnel: w1477 -> [w1490 w1496]
              tunnel: [w1489 w1495] -> w1480
              tunnel: w1478 -> [w1488 w1494]
              tunnel: [w1487 w1492] -> w1479
              frame False {
                n605 = call-poly "Enqueue Message.vi"("error in (no error)"=w1490, "Message"="Resume Sequence", "Message Queue"=w1488) -> ("error out"=w1489:errorcluster, "dup Message Queue"=w1487:refnum<queue>)  [unwired: 7 in]
              }
              frame True {
                n606 = call-poly "Enqueue Message.vi"("error in (no error)"=w1496, "Message"="Pause Sequence", "Message Queue"=w1494) -> ("error out"=w1495:errorcluster, "dup Message Queue"=w1492:refnum<queue>)  [unwired: 7 in]
              }
            }
            n607 = case "Start?" shown="True" w1483 {
              tunnel: w1480 -> [w1497 w1501]
              tunnel: [w1497 w1500] -> w1476
              tunnel: w1479 -> [_ w1499]
              frame False {
              }
              frame True {
                n608 = call-poly "Enqueue Message.vi"("error in (no error)"=w1501, "Message"="Start Sequence", "Message Queue"=w1499) -> ("error out"=w1500:errorcluster)  [unwired: 7 in, 1 out]
              }
            }
          }
          frame True {
          }
        }
        n609 = call "Write to Log File.vi"("error in"=w1465, "text"="Main: Sequencer Opened") -> ()  [unwired: 9 in, 1 out]
      }
      frame "Launch Data Rate Dialog" {
        # "Control the execution of the Sequencer"
        n610 = call "Data Rate Dialog.vi"("error in (no error)"=w1507, 11:w1504) -> ("error out"=w1506:errorcluster, 3:w1505:T1)  [unwired: 8 in]
        n611 = call "Write to Log File.vi"("error in"=w1506, "text"="Main: Data Rate Dialog Opened") -> ()  [unwired: 9 in, 1 out]
      }
      frame "Launch TCP Setup Dialog" {
        # "Control the execution of the Sequencer"
        n612 = call "TCP Settings Dialog.vi"("Message Queues out"=w1512) -> ()  [unwired: 11 in]
        n613 = call "Write to Log File.vi"("error in"=w1511, "text"="Main: TCP Dialog Opened") -> ("error out"=w1510:errorcluster)  [unwired: 9 in]
      }
      frame "Reset Global Variables" {
        n614 = flat-sequence {
          tunnel: [w1532] -> w1521
          tunnel: w1516 -> [w1531]
          tunnel: w1521 -> [w1534]
          tunnel: [w1534] -> w1520
          tunnel: w1520 -> [w1536]
          tunnel: [w1535] -> w1517
          frame #0 {
            n615 = shared-variable ".\\Support Library.lvlib\\Globals.lvlib\\Ismatec 4083 Global"(T91 [{"Busy"=FALSE, "ChannelCnt"=0.0, "Initialized"=FALSE, "Current Channel"=0.0, "Initialized Channels"=[]}, {"Busy"=FALSE, "ChannelCnt"=0.0, "Initialized"=FALSE, "Current Channel"=0.0, "Initialized Channels"=[]}, {"Busy"=FALSE, "ChannelCnt"=0.0, "Initialized"=FALSE, "Current Channel"=0.0, "Initialized Channels"=[]}, {"Busy"=FALSE, "ChannelCnt"=0.0, "Initialized"=FALSE, "Current Channel"=0.0, "Initialized Channels"=[]}, {"Busy"=FALSE, "ChannelCnt"=0.0, "Initialized"=FALSE, "Current Channel"=0.0, "Initialized Channels"=[]}, {"Busy"=FALSE, "ChannelCnt"=0.0, "Initialized"=FALSE, "Current Channel"=0.0, "Initialized Channels"=[]}, {"Busy"=FALSE, "ChannelCnt"=0.0, "Initialized"=FALSE, "Current Channel"=0.0, "Initialized Channels"=[]}, {"Busy"=FALSE, "ChannelCnt"=0.0, "Initialized"=FALSE, "Current Channel"=0.0, "Initialized Channels"=[]}, {"Busy"=FALSE, "ChannelCnt"=0.0, "Initialized"=FALSE, "Current Channel"=0.0, "Initialized Channels"=[]}, {"Busy"=FALSE, "ChannelCnt"=0.0, "Initialized"=FALSE, "Current Channel"=0.0, "Initialized Channels"=[]}, {"Busy"=FALSE, "ChannelCnt"=0.0, "Initialized"=FALSE, "Current Channel"=0.0, "Initialized Channels"=[]}, {"Busy"=FALSE, "ChannelCnt"=0.0, "Initialized"=FALSE, "Current Channel"=0.0, "Initialized Channels"=[]}, {"Busy"=FALSE, "ChannelCnt"=0.0, "Initialized"=FALSE, "Current Channel"=0.0, "Initialized Channels"=[]}, {"Busy"=FALSE, "ChannelCnt"=0.0, "Initialized"=FALSE, "Current Channel"=0.0, "Initialized Channels"=[]}, {"Busy"=FALSE, "ChannelCnt"=0.0, "Initialized"=FALSE, "Current Channel"=0.0, "Initialized Channels"=[]}, {"Busy"=FALSE, "ChannelCnt"=0.0, "Initialized"=FALSE, "Current Channel"=0.0, "Initialized Channels"=[]}, {"Busy"=FALSE, "ChannelCnt"=0.0, "Initialized"=FALSE, "Current Channel"=0.0, "Initialized Channels"=[]}, {"Busy"=FALSE, "ChannelCnt"=0.0, "Initialized"=FALSE, "Current Channel"=0.0, "Initialized Channels"=[]}, {"Busy"=FALSE, "ChannelCnt"=0.0, "Initialized"=FALSE, "Current Channel"=0.0, "Initialized Channels"=[]}, {"Busy"=FALSE, "ChannelCnt"=0.0, "Initialized"=FALSE, "Current Channel"=0.0, "Initialized Channels"=[]}, {"Busy"=FALSE, "ChannelCnt"=0.0, "Initialized"=FALSE, "Current Channel"=0.0, "Initialized Channels"=[]}] ("Array"), error in=w1531) -> (error out=w1532:errorcluster)
          }
          frame #1 {
            n616 = Wait (ms)(milliseconds to wait=u32 100) -> ()  [unwired: 1 out]
          }
          frame #2 {
            n617 = shared-variable ".\\Support Library.lvlib\\Globals.lvlib\\Ismatec 4083 Global"(error in=w1536) -> (error out=w1535:errorcluster)  [unwired: 1 out]
          }
        }
        n618 = flat-sequence {
          tunnel: [w1525] -> w1519
          tunnel: w1516 -> [w1524]
          tunnel: w1519 -> [w1527]
          tunnel: [w1527] -> w1518
          tunnel: w1518 -> [w1529]
          tunnel: [w1528] -> w1515
          frame #0 {
            n619 = shared-variable ".\\Support Library.lvlib\\Globals.lvlib\\ASIA Pump Global"(T81 [{"Busy"=FALSE, "PumpCnt"=0.0, "RemoteEntered"=FALSE, "OverpressureSet"=FALSE}, {"Busy"=FALSE, "PumpCnt"=0.0, "RemoteEntered"=FALSE, "OverpressureSet"=FALSE}, {"Busy"=FALSE, "PumpCnt"=0.0, "RemoteEntered"=FALSE, "OverpressureSet"=FALSE}, {"Busy"=FALSE, "PumpCnt"=0.0, "RemoteEntered"=FALSE, "OverpressureSet"=FALSE}, {"Busy"=FALSE, "PumpCnt"=0.0, "RemoteEntered"=FALSE, "OverpressureSet"=FALSE}, {"Busy"=FALSE, "PumpCnt"=0.0, "RemoteEntered"=FALSE, "OverpressureSet"=FALSE}, {"Busy"=FALSE, "PumpCnt"=0.0, "RemoteEntered"=FALSE, "OverpressureSet"=FALSE}, {"Busy"=FALSE, "PumpCnt"=0.0, "RemoteEntered"=FALSE, "OverpressureSet"=FALSE}, {"Busy"=FALSE, "PumpCnt"=0.0, "RemoteEntered"=FALSE, "OverpressureSet"=FALSE}, {"Busy"=FALSE, "PumpCnt"=0.0, "RemoteEntered"=FALSE, "OverpressureSet"=FALSE}, {"Busy"=FALSE, "PumpCnt"=0.0, "RemoteEntered"=FALSE, "OverpressureSet"=FALSE}, {"Busy"=FALSE, "PumpCnt"=0.0, "RemoteEntered"=FALSE, "OverpressureSet"=FALSE}, {"Busy"=FALSE, "PumpCnt"=0.0, "RemoteEntered"=FALSE, "OverpressureSet"=FALSE}] ("ASIA Pump Global"), error in=w1524) -> (error out=w1525:errorcluster)
          }
          frame #1 {
            n620 = Wait (ms)(milliseconds to wait=u32 100) -> ()  [unwired: 1 out]
          }
          frame #2 {
            n621 = shared-variable ".\\Support Library.lvlib\\Globals.lvlib\\ASIA Pump Global"(error in=w1529) -> (error out=w1528:errorcluster)  [unwired: 1 out]
          }
        }
        n622 = Merge Errors(w1517, w1516, w1515) -> (w1514:errorcluster)
      }
      frame "Launch Calibration Dialog" {
        # "Run the Calibration Program"
        n623 = call "Calibration Main.vi"("error in (no error)"=w1541, "Pump Calibration Config in"=T93 {"Settings"={"Cycle Period"=500.0, "Ismatech"={"VISA resource name"="", "Simulated?"=TRUE, "Pump Number"=1.0, "Reverse?"=FALSE}, "Masterflex"={"VISA resource name"="", "Simulated?"=TRUE, "Pump Number"=1.0, "Reverse?"=FALSE}, "Bronkhorst M13 Settings"={"VISA resource name"="", "Simulated?"=TRUE, "Smoothing Steps"=1}, "PID 2 Parameters"={"Input Device"=enum."Default", "Output Device"=enum."Default"}, "Tacmina Settings"={"Analog DAQ Task"="", "Digital DAQ Task"=""}, "KNF SIMDOS Settings"={"VISA resource name"="", "Simulated?"=TRUE}, "VICI M50 Settings"={"VISA resource name"="", "Simulated?"=TRUE, "Pump Letter"="", "Reverse?"=FALSE}, "FLOM Settings"={"VISA resource name"="", "Simulated?"=TRUE, "Pump Number"=0.0}, "Calibration Limits"={"Minimum (ml/min)"=0.0, "Maximum (ml/min)"=0.0, "Steps"=0.0}, "SSI PR Settings"={"VISA resource name"="", "Simulated?"=FALSE}, "Ismatech 4308 Settings"={"VISA resource name"="", "Pump Number"=1, "Channel Number"=0, "Simulated?"=TRUE, "Reverse?"=FALSE}, "Bronkhorst M14 Settings"={"VISA resource name"="", "Simulated?"=FALSE, "Smoothing Steps"=1}}, "Flowmeter Output"=0.0, "Density"=0.0, "FL Temp"=0.0, "Speed %"=0.0, "File Refnum"=refnum, "Pump On?"=enum."Not Initialized"}) -> ("error out"=w1540:errorcluster)  [unwired: 8 in, 1 out]
        n624 = call "Write to Log File.vi"("error in"=w1540, "text"="Main: Calibration Opened") -> ("error out"=w1539:errorcluster)  [unwired: 9 in]
      }
      frame "Launch Note Dialog" {
        # "Open the dialog for adding notes to the data file"
        n625 = call-poly "Enqueue Message.vi"("error in (no error)"=w1547, "Message"="Add Note", "Message Queue"=w1548) -> ("error out"=w1543:errorcluster)  [unwired: 7 in, 1 out]
        n626 = call "Write to Log File.vi"("error in"=w1543, "text"="Main: Note Dialog Opened") -> ()  [unwired: 9 in, 1 out]
      }
      frame Default {
        # "'Default' case only runs if there is a message that isn't defined in any of the other cases.  Output a programming error."
        n627 = Concatenate Strings("The invalid message string " ("string"), w1550, " was received in Main." ("string")) -> (w1551:string)
        n628 = Bundle By Name(cluster=errorcluster {"status"=TRUE, "code"=1, "source"=""} ("error constant"), "source"=w1551) -> (w1549:errorcluster)
        n629 = call <vilib>:"General Error Handler.vi"("error in (no error)"=w1549) -> ("message"=w1555:string)  [unwired: 10 in, 4 out]
        n630 = Concatenate Strings("Main: Note Dialog Opened" ("text"), w1555) -> (w1556:string)
        n631 = call "Write to Log File.vi"("text"=w1556) -> ()  [unwired: 10 in, 1 out]
      }
      frame "Tags Created" {
        n632 = call "Write to Log File.vi"("error in"=w1559, "text"="Main: Tags Created") -> ()  [unwired: 9 in, 1 out]
      }
    }
    "Cluster" <- w112
    n633 = call "Error Handler - Message Handling Loop.vi"("error in (no error)"=w118, "Message Queue"=w116) -> ("dup error in"=w117:errorcluster, "dup Message Queue"=w110:refnum<queue>)  [unwired: 8 in]
  }
  n634 = Build Path(base path=w66, name or relative path="History Graph Message Loop.vi") -> (appended path=w65:path)
  n635 = Open VI Reference(vi path=w65) -> (vi reference=w72:refnum<vi>, error out=w70:errorcluster)  [unwired: 5 in]
  n636 = while {
    tunnel: w82 -> [w1564]
    tunnel: [w1573] -> w86
    shift-right: [w1571] -> w83
    shift-left: w47 -> [w1575]
    tunnel: w64 -> [w1563]
    shift-right: [w1569] -> _
    shift-left: T79 {"Down"=FALSE, "Mouse"={"Mouse Position"={"X"=0, "Y"=0}, "Mouse Modifiers"={"Button Down"=FALSE, "Shift Mod"=FALSE, "Menu Mod"=FALSE, "Option Mod"=FALSE}}, "Drag"=FALSE, "Canvas"=FALSE} -> [w1570]
    tunnel: w52 -> [w1567]
    tunnel: w51 -> [w1566]
    tunnel: w42 -> [w1562]
    stop <- w1572 stop-if-true
    # "Event Handling Loop"
    n637 = event shown="[4] Timeout" {
      selector: w1575 -> [_ _ _ _ _ _ _ _ _ _ _ _ _ _ _ _ _]
      dyn-events: [_ _ _ _ _ _ _ _ _ _ _ _ _ _ _ _ _] -> w1571
      timeout: 1000 -> [_ _ _ _ _ _ _ _ _ _ _ _ _ _ _ _ _]
      tunnel: w1564 -> [w1579 w1586 w1594 w1612 w1630 w1665 w1675 w1696 w1700 w1706 w1713 w1724 w1731 w1778 w1786 w1797 w1808]
      tunnel: [w1582 w1585 w1591 w1610 _ w1650 w1676 _ w1702 w1703 w1712 w1723 w1728 _ _ w1794 w1803] -> w1574
      tunnel: [TRUE _ _ _ _ _ _ _ _ _ FALSE FALSE w1730 _ _ TRUE TRUE] -> w1572
      tunnel: w1563 -> [_ _ _ _ _ _ _ _ _ _ _ _ w1729 _ _ _ _]
      tunnel: w1570 -> [w1576 w1583 w1589 w1614 w1641 w1666 w1674 w1697 w1698 w1704 w1708 w1720 w1727 w1780 w1788 w1796 w1804]
      tunnel: [w1576 w1583 w1588 w1613 w1641 w1666 w1674 w1697 w1698 w1704 w1708 w1720 w1727 w1779 w1789 w1796 w1804] -> w1569
      tunnel: [w1578 w1584 w1594 w1611 w1629 w1665 w1675 w1696 w1699 w1705 w1711 w1722 w1731 w1778 w1786 w1795 w1802] -> w1568
      tunnel: w1567 -> [_ _ _ _ _ _ _ w1692 _ _ _ _ _ _ _ _ _]
      tunnel: w1566 -> [_ _ _ _ _ _ _ w1691 _ _ _ _ _ _ _ _ _]
      tunnel: w1562 -> [_ _ _ _ w1627 _ _ _ _ _ _ _ _ _ _ _ _]
      event "Exit": Value Change {
        w1580 = TRUE  # Priority Message
        # "The UI Message Loop handles sending the Exit message to other loops."
        n638 = event-data() -> ()  [unwired: 1 in, 1 out]
        n639 = call-poly "Enqueue Message.vi"("Priority Message? (F)"=w1580, "Message"="Exit", "Message Queue"=w1579) -> ("error out"=w1582:errorcluster, "dup Message Queue"=w1578:refnum<queue>)  [unwired: 7 in]
      }
      event "Force Trigger": Value Change {
        n640 = event-data() -> ()  [unwired: 1 in, 1 out]
        n641 = call-poly "Enqueue Message.vi"("Message"="Force Trigger", "Message Queue"=w1586) -> ("error out"=w1585:errorcluster, "dup Message Queue"=w1584:refnum<queue>)  [unwired: 8 in]
      }
      event Mouse Up {
        # "If we are draging a module and we are over the canvas"
        n642 = event-data() -> ("Coords"=w1593:T10)  [unwired: 1 in]
        n643 = in-place {
          in-place-border: w1594 -> [w1601]
          in-place-border: w1593 -> [w1600]
          in-place-border: [w1599] -> w1592
          w1595 = FALSE ("Down")
          n644 = in-place-cluster #15(w1589) -> ("Drag"=w1597:bool, "Canvas"=w1596:bool)  [unwired: 1 out]
          n645 = Compound Arithmetic op=AND(w1597, w1596) -> (w1598:bool)
          n646 = case shown="False" w1598 {
            tunnel: [_ w1602] -> w1599
            tunnel: w1601 -> [_ w1605]
            tunnel: w1600 -> [_ w1604]
            frame False {
            }
            frame True {
              n647 = property on="Canvas" class="Pict"() -> ("Mouse"=w1607:T76)  [unwired: 2 in, 2 out]
              n648 = Bundle("Coords"=w1604, "Mouse"=w1607) -> (w1603:cluster{"Coords":T10, "Mouse":T76})  [unwired: 1 in]
              "output cluster" <- w1603
              n649 = call-poly "Enqueue Message.vi"("Message Data"=w1603, "Message"="Drop", "Message Queue"=w1605) -> ("error out"=w1602:errorcluster)  [unwired: 7 in, 1 out]
            }
          }
          n650 = in-place-cluster #15("Down"=w1595, "Drag"=w1595, "Canvas"=w1595) -> (w1588:T79)
        }
        n651 = call-poly <vilib>:"Set Cursor.vi"("error in (no error)"=w1592, "icon"=u16 0) -> ("error out"=w1591:errorcluster)  [unwired: 8 in, 1 out]
      }
      event "Palette": Mouse Down {
        n652 = event-data() -> ()  [unwired: 1 in, 1 out]
        n653 = property on="Palette" class="Pict"() -> ("DisabledEnum"=w1609:T87)  [unwired: 2 in, 2 out]
        n654 = call "Enable Disable Enum to Enabled.vi"("Disabled"=w1609) -> ("Enabled"=w1608:bool)
        n655 = case "Is the palette enabled?" shown="True" w1608 {
          tunnel: w1614 -> [w1615 w1626]
          tunnel: [w1615 w1624] -> w1613
          tunnel: w1612 -> [w1616 w1620]
          tunnel: [w1616 w1619] -> w1611
          tunnel: [_ w1618] -> w1610
          frame False {
          }
          frame True {
            # "Select a module"
            n656 = property on="Palette" class="Pict"() -> ("Mouse"=w1617:T76)  [unwired: 2 in, 2 out]
            n657 = Bundle By Name(cluster=w1626, "Down"=TRUE, "Mouse"=w1617, "Drag"=TRUE, "Canvas"=FALSE) -> (w1624:T79)
            n658 = call-poly "Enqueue Message.vi"("Message Data"=w1617, "Message"="Drag Start", "Message Queue"=w1620) -> ("error out"=w1618:errorcluster, "dup Message Queue"=w1619:refnum<queue>)  [unwired: 7 in]
          }
        }
      }
      event Timeout {
        # "Poll for alarm status and display on UI. This could be changed\nto an alarm Event if necessary."
        n659 = event-data() -> ()  [unwired: 1 in, 1 out]
        n660 = call "Tag FGV.vi"("Operation"=Tag_FGV_Operation_Enum."Read Alarms") -> ("alarms"=w1635:T96)  [unwired: 7 in, 7 out]
        n661 = property on="UI Alarms" class="Arr (strict)"() -> ("Number of Columns"=w1638:u32)  [unwired: 2 in, 2 out]
        n662 = call "Is Critical Alarm Set.vi"("alarms"=w1635) -> ("critical alarm?"=w1633:bool)  [unwired: 10 in]
        n663 = call "Alarm UI.vi"("alarms"=w1635) -> ("UI Alarms"=w1640:T74[], "Alarm Model"=→"Alarm Model":T73[])  [unwired: 9 in]
        n664 = Array Size(array=w1640) -> (size(s)=w1639:i32)
        n665 = Greater?(x=w1639, y=w1638) -> (0:w1637:bool)
        n666 = feedback #16() -> (w1634:bool)  [unwired: 1 in]
        n667 = feedback-in #16(w1633) -> ()
        n668 = local write "UI Alarms"(w1640) -> ()
        n669 = property on="UI Alarms" class="Arr (strict)"("HorizScroll"=w1637) -> ()  [unwired: 2 in, 2 out]
        n670 = property on="Alarm Model" class="Arr (strict)"("Visible"=TRUE) -> ()  [unwired: 2 in, 2 out]
        n671 = Compound Arithmetic op=AND(w1633, invert w1634) -> (w1632:bool)
        n672 = case "critical alarm just occured?" shown="True" w1632 {
          tunnel: [w1642 w1646] -> w1629
          tunnel: w1630 -> [w1642 w1645]
          tunnel: w1627 -> [_ w1643]
          frame False {
          }
          frame True {
            n673 = call-poly "Enqueue Message.vi"("Message"="E-Stop", "Message Queue"=w1645) -> ("dup Message Queue"=w1646:refnum<queue>)  [unwired: 8 in, 1 out]
            n674 = call-poly "Enqueue Message.vi"("Message"="Pause", "Message Queue"=w1643) -> ()  [unwired: 8 in, 2 out]
          }
        }
      }
      event User Event {
        w1663 = T97 {"alarm URL"="", "set time"=timestamp(0 s since 1904-01-01), "set user"="", "ack time"=timestamp(0 s since 1904-01-01), "ack user"="", "clear time"=timestamp(0 s since 1904-01-01), "clear user"="", "setpoint"=0.0, "value"=0.0, "priority"=0, "alarm area"="", "alarm description"="", "ack comment"="", "event?"=FALSE, "Refnum"=0}  # Alarm
        # "NI Example on how this works: .. \\LabVIEW 2018\\examples\\lvdsc\\Data and Alarm Historical Logging\\DSC Alarms Demo\\component\\DSC Alarms Event Structure Support.vi"
        # "critical alarm?"
        n675 = event-data() -> ("alarm URL"=w1662:string, "set time"=w1661:timestamp, "set user"=w1660:string, "ack time"=w1659:timestamp, "ack user"=w1658:string, "clear time"=w1657:timestamp, "clear user"=w1656:string, "setpoint"=w1655:dbl, "value"=w1654:dbl, "priority"=w1651:u32, "alarm area"=w1653:string, "alarm description"=w1652:string)  [unwired: 1 in]
        n676 = Bundle By Name(cluster=w1663, "alarm URL"=w1662, "set time"=w1661, "set user"=w1660, "ack time"=w1659, "ack user"=w1658, "clear time"=w1657, "clear user"=w1656, "setpoint"=w1655, "value"=w1654, "priority"=w1651, "alarm area"=w1653, "alarm description"=w1652) -> (w1649:T97)
        n677 = Greater?(x=w1661, y=timestamp(2272129200 s since 1904-01-01)) -> (0:w1648:bool)
        n678 = case "valid time stamp?" shown="True" w1648 {
          tunnel: [w1667 w1672] -> w1650
          tunnel: w1649 -> [_ w1668]
          frame False {
            n679 = call <vilib>:"Clear Errors.vi"() -> ("error out"=w1667:errorcluster)  [unwired: 6 in, 1 out]
          }
          frame True {
            # "Log alarm to alarm\nCSV file."
            n680 = call "Log Alarm FGV.vi"("Alarm"=w1668, "Operation"=Alarm_Log_Operation_Enum."Log Alarm") -> ("error out"=w1672:errorcluster)  [unwired: 9 in]
            n681 = Flatten To XML(anything=w1668) -> (xml string=w1669:string)
            n682 = Concatenate Strings("ALARM: " ("text"), w1669) -> (w1670:string)
            n683 = call "Write to Log File.vi"("error in"=w1672, "text"=w1670) -> ()  [unwired: 9 in, 1 out]
          }
        }
        n684 = disable-structure shown="Disabled" {
          frame Disabled {
            # "Example of\nalarm events using\nsame low level VIs."
            n685 = call "DSC Alarm Event Example.vi"() -> ()  [unwired: 12 in]
          }
          frame Enabled {
          }
        }
      }
      event "UI Alarms": Value Change {
        # "Acknowlege the alarms when it's button is clicked"
        n686 = event-data() -> ()  [unwired: 1 in, 1 out]
        n687 = local read "Alarm Model"() -> (w1678:T73[])
        n688 = call <vilib>:"Clear Errors.vi"() -> ("error out"=w1677:errorcluster)  [unwired: 6 in, 1 out]
        n689 = for {
          shift-right: [w1684] -> w1676
          shift-left: w1677 -> [w1685]
          tunnel: "UI Alarms" -> [w1683] mode=indexing
          tunnel: w1678 -> [w1681] mode=indexing
          n690 = Unbundle By Name(w1681) -> ("Alarm"=w1680:T97)
          n691 = Unbundle By Name(w1683) -> ("Ack"=w1682:bool)
          n692 = case shown="True" w1682 {
            tunnel: w1685 -> [w1686 w1690]
            tunnel: [w1686 w1689] -> w1684
            tunnel: w1680 -> [_ w1687]
            frame False {
            }
            frame True {
              n693 = call "Tag FGV.vi"("Operation"=Tag_FGV_Operation_Enum."Ack Alarm", "Data"=w1687, "error in (no error)"=w1690) -> ("error out"=w1689:errorcluster)  [unwired: 5 in, 7 out]
            }
          }
        }
      }
      event "Alarm History Button": Value Change {
        # "Open Alarm History VI"
        # "Don't care if VI is\nalready running."
        n694 = event-data() -> ()  [unwired: 1 in, 1 out]
        n695 = call-by-ref "Start Asynchronous Call"(reference=w1692, "user event"=w1691) -> (reference out=w1694:refnum<vi>, error out=w1693:errorcluster)  [unwired: 12 in]
        n696 = call <vilib>:"Clear Errors.vi"("error in (no error)"=w1693) -> ()  [unwired: 5 in, 2 out]
        n697 = invoke class="VI (strict)" method="FP.Open"(reference=w1694, "State"=T95."Standard") -> ()  [unwired: 3 in, 5 out]
        n698 = disable-structure shown="Disabled" {
          frame Disabled {
            n699 = call "Alarm History.vi"() -> ()  [unwired: 12 in]
          }
          frame Enabled {
          }
        }
      }
      event "Settings": Value Change {
        n700 = event-data() -> ()  [unwired: 1 in, 1 out]
        n701 = call-poly "Enqueue Message.vi"("Message"="Launch Settings Dialog", "Message Queue"=w1700) -> ("error out"=w1702:errorcluster, "dup Message Queue"=w1699:refnum<queue>)  [unwired: 8 in]
      }
      event "Start Log": Value Change {
        n702 = event-data() -> ()  [unwired: 1 in, 1 out]
        n703 = call-poly "Enqueue Message.vi"("Message"="Start Log", "Message Queue"=w1706) -> ("error out"=w1703:errorcluster, "dup Message Queue"=w1705:refnum<queue>)  [unwired: 8 in]
      }
      event "Pause Log Button": Value Change {
        n704 = event-data() -> ()  [unwired: 1 in, 1 out]
        n705 = global write "Main Globals.vi" "Pause Log"("Pause Log Button") -> ()
        n706 = disable-structure shown="Enabled" {
          disable-tunnel: w1713 -> [w1718 w1719]
          disable-tunnel: [w1717 _] -> w1712
          disable-tunnel: [w1716 w1719] -> w1711
          disable-tunnel: "Pause Log Button" -> [w1714 _]
          frame Disabled {
            n707 = call-poly "Enqueue Message.vi"("Message Data"=w1714, "Message"="Pause Log", "Message Queue"=w1718) -> ("error out"=w1717:errorcluster, "dup Message Queue"=w1716:refnum<queue>)  [unwired: 7 in]
          }
          frame Enabled {
          }
        }
      }
      event "E-Stop": Value Change {
        n708 = event-data() -> ()  [unwired: 1 in, 1 out]
        n709 = call-poly "Enqueue Message.vi"("Message"="E-Stop", "Message Queue"=w1724) -> ("error out"=w1723:errorcluster, "dup Message Queue"=w1722:refnum<queue>)  [unwired: 8 in]
      }
      event Menu Selection (User) {
        n710 = event-data() -> ("ItemTag"=w1726:string)  [unwired: 1 in]
        n711 = case shown="\"TCP Setup\"" w1726 {
          tunnel: w1731 -> [_ _ _ w1743 w1746 w1749 w1753 w1755 w1758 w1761 w1765 w1768 w1771 w1776]
          tunnel: [_ _ _ _ _ _ _ _ _ _ _ _ _ TRUE] -> w1730
          tunnel: w1729 -> [_ _ w1741 _ _ _ _ _ _ _ _ _ _ _]
          tunnel: [w1732 w1733 w1740 w1744 w1747 w1750 w1754 w1756 w1759 w1762 w1764 w1767 w1770 w1775] -> w1728
          frame Default {
            n712 = call <vilib>:"Clear Errors.vi"() -> ("error out"=w1732:errorcluster)  [unwired: 6 in, 1 out]
          }
          frame "Open BMP" {
            n713 = call "File Dialog"() -> ("selected path"=w1734:path, "cancelled"=w1735:bool)  [unwired: 12 in, 2 out]
            n714 = case shown="False" w1735 {
              tunnel: w1734 -> [w1737 _]
              frame False {
                n715 = call "Empty Picture"() -> ("empty picture"=w1736:picture)
                n716 = call "Draw BMP at Location.vi"("selected path"=w1737, "picture in"=w1736) -> ("image data"=→"image data":T77, "picture out"=→"Canvas":picture)  [unwired: 7 in, 1 out]
              }
              frame True {
              }
            }
            n717 = call <vilib>:"Clear Errors.vi"() -> ("error out"=w1733:errorcluster)  [unwired: 6 in, 1 out]
          }
          frame "DAQSettings" {
            # "Open the DAQ Settings dialog"
            n718 = call-poly "Enqueue Message.vi"("Message"="DAQ-Settings", "Message Queue"=w1741) -> ("error out"=w1740:errorcluster)  [unwired: 8 in, 1 out]
          }
          frame "Open Campaign" {
            n719 = call-poly "Enqueue Message.vi"("Message"="Open Campaign", "Message Queue"=w1743) -> ("error out"=w1744:errorcluster)  [unwired: 8 in, 1 out]
          }
          frame "Save Campaign" {
            n720 = call-poly "Enqueue Message.vi"("Message"="Save Campaign", "Message Queue"=w1746) -> ("error out"=w1747:errorcluster)  [unwired: 8 in, 1 out]
          }
          frame "Save Campaign As..." {
            n721 = call-poly "Enqueue Message.vi"("Message"="Save Campaign As", "Message Queue"=w1749) -> ("error out"=w1750:errorcluster)  [unwired: 8 in, 1 out]
          }
          frame "FileSettings" {
            # "Open the File Settings dialog"
            n722 = call-poly "Enqueue Message.vi"("Message"="File-Settings", "Message Queue"=w1753) -> ("error out"=w1754:errorcluster)  [unwired: 8 in, 1 out]
          }
          frame "Set Sequence" {
            n723 = call-poly "Enqueue Message.vi"("Message"="Launch Sequence Dialog", "Message Queue"=w1755) -> ("error out"=w1756:errorcluster)  [unwired: 8 in, 1 out]
          }
          frame "Set Data Rate" {
            n724 = call-poly "Enqueue Message.vi"("Message"="Launch Data Rate Dialog", "Message Queue"=w1758) -> ("error out"=w1759:errorcluster)  [unwired: 8 in, 1 out]
          }
          frame "TCP Setup" {
            n725 = call-poly "Enqueue Message.vi"("Message"="Launch TCP Setup Dialog", "Message Queue"=w1761) -> ("error out"=w1762:errorcluster)  [unwired: 8 in, 1 out]
          }
          frame "Reset Global Variables" {
            n726 = call-poly "Enqueue Message.vi"("Message"="Reset Global Variables", "Message Queue"=w1765) -> ("error out"=w1764:errorcluster)  [unwired: 8 in, 1 out]
          }
          frame "Launch Calibration Dialog" {
            n727 = call-poly "Enqueue Message.vi"("Message"="Launch Calibration Dialog", "Message Queue"=w1768) -> ("error out"=w1767:errorcluster)  [unwired: 8 in, 1 out]
          }
          frame "Add Note" {
            n728 = call-poly "Enqueue Message.vi"("Message"="Launch Note Dialog", "Message Queue"=w1771) -> ("error out"=w1770:errorcluster)  [unwired: 8 in, 1 out]
          }
          frame "Exit" {
            w1773 = TRUE  # Priority Message
            n729 = call-poly "Enqueue Message.vi"("Priority Message? (F)"=w1773, "Message"="Exit", "Message Queue"=w1776) -> ("error out"=w1775:errorcluster)  [unwired: 7 in, 1 out]
          }
        }
      }
      event "Canvas": Mouse Enter {
        n730 = event-data() -> ()  [unwired: 1 in, 1 out]
        n731 = Unbundle By Name(w1780) -> ("Drag"=w1781:bool)
        n732 = case shown="False" w1781 {
          tunnel: w1780 -> [w1782 w1785]
          tunnel: [w1782 w1784] -> w1779
          frame False {
          }
          frame True {
            n733 = Bundle By Name(cluster=w1785, "Canvas"=TRUE) -> (w1784:T79)
          }
        }
      }
      event "Canvas": Mouse Leave {
        n734 = event-data() -> ()  [unwired: 1 in, 1 out]
        n735 = Unbundle By Name(w1788) -> ("Canvas"=w1787:bool)
        n736 = case shown="False" w1787 {
          tunnel: w1788 -> [w1790 w1793]
          tunnel: [w1790 w1792] -> w1789
          frame False {
          }
          frame True {
            n737 = Bundle By Name(cluster=w1793, "Canvas"=FALSE) -> (w1792:T79)
          }
        }
      }
      event Panel Close? {
        w1798 = TRUE  # Priority Message
        # "Send the 'Confirm Quit' message if the user closes the panel of the VI. Discard the event so the 'Confirm Quit' message has a chance to run."
        n738 = event-data() -> ()  [unwired: 1 in, 1 out]
        n739 = invoke class="VI" method="FP.Close"() -> ()  [unwired: 3 in, 3 out]
        n740 = call-poly "Enqueue Message.vi"("Priority Message? (F)"=w1798, "Message"="Exit", "Message Queue"=w1797) -> ("error out"=w1794:errorcluster, "dup Message Queue"=w1795:refnum<queue>)  [unwired: 7 in]
        n741 = event-data("Discard?"=TRUE) -> ()  [unwired: 1 in, 1 out]
      }
      event "End Program": Value Change {
        w1805 = FALSE  # Priority Message
        # "Send the 'Confirm Quit' message if the user closes the panel of the VI. Discard the event so the 'Confirm Quit' message has a chance to run."
        n742 = event-data() -> ()  [unwired: 1 in, 1 out]
        n743 = call-poly "Enqueue Message.vi"("Priority Message? (F)"=w1805, "Message"="Exit", "Message Queue"=w1808) -> ("error out"=w1803:errorcluster, "dup Message Queue"=w1802:refnum<queue>)  [unwired: 7 in]
      }
    }
    n744 = call "Error Handler - Event Handling Loop.vi"("error in (no error)"=w1574, "Message Queue"=w1568) -> ("dup error in"=w1573:errorcluster)  [unwired: 8 in, 1 out]
  }
  n745 = invoke class="VI" method="Ctrl Val.Set"(reference=w72, error in=w70, "Control Name"="Message Queues", "Value"=w29) -> (reference out=w71:refnum<vi>, error out=w69:errorcluster)  [unwired: 1 in, 3 out]
  n746 = invoke class="VI" method="Run VI"(reference=w71, error in=w69, "Wait until done"=FALSE ("Wait Until Done"), "Auto Dispose Ref"=FALSE ("Auto Dispose Reference")) -> (reference out=w74:refnum<vi>)  [unwired: 1 in, 4 out]
  n747 = invoke on="Sub Panel" class="SubPnl" method="Insert VI"("VI Ref"=w74) -> (error out=→"error out":errorcluster)  [unwired: 3 in, 3 out]
  n748 = Unregister For Events(event registration refnum=w83, error in=w86) -> (error out=w53:errorcluster)
  n749 = disable-structure shown="Disabled" {
    frame Disabled {
      n750 = call "Feed Module (Main).vi"() -> ()  [unwired: 12 in]
      n751 = call "Tag FGV.vi"() -> ()  [unwired: 6 in, 6 out]
      n752 = call "TT (Main).vi"() -> ()  [unwired: 12 in]
      n753 = call "PT (Main).vi"() -> ()  [unwired: 12 in]
      n754 = call "History Graph Message Loop.vi"() -> ()  [unwired: 11 in, 1 out]
      n755 = call "Scale Module (Main).vi"() -> ()  [unwired: 12 in]
      n756 = call "Log Alarm FGV.vi"() -> ()  [unwired: 11 in, 1 out]
      n757 = call "Pump Module (Main).vi"() -> ()  [unwired: 12 in]
    }
    frame Enabled {
    }
  }
  n758 = Generate User Event(user event=w51, event data cluster=w50, error in=w53) -> (error out=w56:errorcluster)  [unwired: 1 in, 1 out]
  n759 = invoke class="VI (strict)" method="FP.Close"(reference=w52, error in=w56) -> (error out=w55:errorcluster)  [unwired: 1 in, 2 out]
  n760 = call <vilib>:"Clear Errors.vi"("error in (no error)"=w55) -> ("error out"=w54:errorcluster)  [unwired: 5 in, 1 out]
  n761 = Close Reference(reference=w52, error in (no error)=w54) -> ()  [unwired: 1 out]
  n762 = Merge Errors(w53, w87, w36, w35, w34, w33, w32) -> (w85:errorcluster)
  n763 = call "Destroy User Event - Stop.vi"("error in (no error)"=w85, "User Event - Stop"=w84) -> ("error out"=w38:errorcluster)  [unwired: 9 in]
  n764 = call "Close File.vi"("error in"=w38) -> ("error out"=w12:errorcluster)  [unwired: 10 in]
  n765 = Release Queue(queue=w13, error in (no error)=w12) -> (error out=w11:errorcluster)  [unwired: 1 in, 2 out]
  n766 = Release Queue(queue=w14, error in (no error)=w11) -> (error out=w10:errorcluster)  [unwired: 1 in, 2 out]
  n767 = Release Queue(queue=w15, error in (no error)=w10) -> (error out=w9:errorcluster)  [unwired: 1 in, 2 out]
  n768 = for {
    tunnel: w16 -> [w1811] mode=indexing
    tunnel: w9 -> [w1810]
    tunnel: [w1809] -> _ mode=indexing
    tunnel: [w1809] -> w8
    n769 = Release Queue(queue=w1811, error in (no error)=w1810) -> (error out=w1809:errorcluster)  [unwired: 1 in, 2 out]
  }
  n770 = Merge Errors(w8) -> (w7:errorcluster)
  n771 = Release Queue(queue=w17, error in (no error)=w7) -> (error out=w6:errorcluster)  [unwired: 1 in, 2 out]
  n772 = Release Queue(queue=w18, error in (no error)=w6) -> (error out=w5:errorcluster)  [unwired: 1 in, 2 out]
  n773 = Release Queue(queue=w26, error in (no error)=w5) -> (error out=w4:errorcluster)  [unwired: 1 in, 2 out]
  n774 = Release Queue(queue=w27, error in (no error)=w4) -> (error out=w3:errorcluster)  [unwired: 1 in, 2 out]
  n775 = Release Queue(queue=w25, error in (no error)=w3) -> (error out=w2:errorcluster)  [unwired: 1 in, 2 out]
  n776 = Release Queue(queue=w28, error in (no error)=w2) -> (error out=w1:errorcluster)  [unwired: 1 in, 2 out]
  n777 = disable-structure shown="Default" {
    disable-tunnel: w1 -> [_ _]
    frame condition #0 {
      # "Call Quit LabVIEW if running as a built application."
      n778 = Quit LabVIEW() -> ()  [unwired: 1 in]
    }
    frame condition #1 (active) {
    }
  }
